vi "OP_Print_TPS_cluster_20171110.vi"() -> ()   [LabVIEW 2013]
uses:
  <vilib>/addons/database/Connection.llb/DB Tools Open Connec (Path).vi
  <vilib>/addons/database/Connection.llb/Conn Execute.vi
  <vilib>/addons/database/Recordset.llb/Rec Fetch Recordset Data (R).vi
  <vilib>/addons/database/Recordset.llb/Rec Destroy - Connection.vi
  <userlib>/caLab/Private/Get_PV-1D.vi
  <vilib>/Utility/file.llb/Write To Spreadsheet File (string).vi
  <userlib>/caLab/Private/Get_PV.vi
  <vilib>/addons/database/NI_Database_API.lvlib
panel:
  in  "T:Slow\nF:Fast":bool
  in  "Switch Tab":bool=TRUE
  out "Tab Control":enum32{"_____", "           "}(tab)
  out "Cluster":T1={"SR Fill Pattern"=[], "Beam Current(mA"=320.769453, "Beam Lifetime(min)"=354.3939151043138, "Beamsize X(um)"=63.15189373514937, "Beamsize Y(um)"=38.03691397287648, "Tune X(from BPM)"=0.1487279843444227, "Tune Y(from BPM)"=0.2309197651663405, "Mode"="Top-Up", "NuX(from BBF) "=0.15142063757609414, "NuY(from BBF)"=0.22496346361412184, "IU22-23gap(R)"=7.0, "IU22-05gap(R)"=7.372, "IU22-05M"=TRUE, "IU22A-09gap(R)"=8.05, "IU22A-09M"=TRUE, "IU22B-09gap(R)"=40.001, "IU22B-09M"=FALSE, "IUT22-21gap(R)"=7.0, "IUT22-21M"=TRUE, "IU22-23M"=TRUE, "IU22A-25gap(R)"=7.0, "IU22A-25M"=TRUE, "IU22B-25gap(R)"=40.0, "IU22B-25M"=FALSE, "EPU48A-41gap(R)"=65.00055, "EPU48A-41gM"=FALSE, "EPU48B-41gap(R)"=27.450000000000003, "EPU48B-41gM"=TRUE, "EPU46-45gap(R)"=44.99850000000001, "EPU46-45gM"=FALSE, "EPU48A-41phase(R)"=0.00055, "EPU48B-41phase(R)"=0.0, "EPU46-45phase(R)"=5e-05, "Grid volt.(V)[S]"=33.0, "Gun mode"="MBM", "Mod.3 HV(kV)[S]"=35.37999999999996, "SR"="SR_DMB_2017_1024_0300LOCO.data", "BR"="Booster_2017_1023_0900.data", "LI"="Linac_2017_0413_1015.data", "LTB"="LTB_JT_2017_0828_1050.data", "BTS"="BTS_2017_1023_0900.data", "RF2 remote"=TRUE, "RF2 OP mode"=TRUE, "RF2 phase.[S]"=-42.0, "RF Freq.(s)"=499655365.67399085, "RF2 gap volt[S]"=1600.0, "RF3 remote"=TRUE, "RF3 OP mode"=TRUE, "RF3 phase.[S]"=1.1999999999999995, "RF3 gap volt.[S]"=1600.0, "BBF V"=TRUE, "BBF H"=TRUE, "BR ext. kicker1(kV)"=17.666, "BR ext. kicker2(kV)"=17.666, "BR ext. sep.1(V)"=322.14, "BR ext. sep.2(V)"=441.1, "BR inj. sep.(V)"=104.95, "BR inj. kicker(kV)"=13.449999999999969, "SR kicker4(kV)"=7.945, "SR kicker3(kV)"=8.02, "SR kicker2(kV)"=8.142, "SR kicker1(kV)"=8.1, "SR inj. sep.2(V)"=397.2, "SR inj. sep.1(V)"=398.04, "Bucket Start"=100.0, "Bucket Last"=450.0, "Bucket Step"=10.0, "Orbit ILK(P)"=TRUE, "IU22-05 Hutch Enable"=TRUE, "IU22A-09M Hutch Enable"=TRUE, "IUT22-21M Hutch Enable"=TRUE, "IU22-23M Hutch Enable"=TRUE, "IU22A-25M Hutch Enable"=TRUE, "EPU48A-41M Hutch Enable"=TRUE, "EPU46-45M Hutch Enable"=FALSE, "EPU46-45 FE Enable"=TRUE, "EPU48A-41 FE Enable"=TRUE, "IU22A-25 FE Enable"=TRUE, "IU22-23 FE Enable"=TRUE, "IUT22-21 FE Enable"=TRUE, "IU22A-09 FE Enable"=TRUE, "IU22-05 FE Enable"=TRUE, "EPU48A-41pM"=FALSE, "EPU48B-41pM"=TRUE, "EPU46-45pM"=FALSE, "Gun volt.(V)[S]"=23.5, "Width count"=75.0, "2ns step"=2.0, "10ps delay"=150.0, "phase shifter"=130.0015, "Taper"=1.0899999999999999, "05XBPMX 1"=14.279, "09XBPMX 1"=-34.837, "21XBPMX 1"=-36.466, "23XBPMX 1"=-38.547000000000004, "25XBPMX 1"=-40.08, "41XBPMX 1"=-513.551, "45XBPMX 1"=-12.86, "05XBPMY 1"=51.999, "09XBPMY 1"=30.004, "21XBPMY 1"=-4.771, "23XBPMY 1"=19.080000000000002, "25XBPMY 1"=-4.366, "41XBPMY 1"=309.241, "45XBPMY 1"=1.842, "FOFB H"="On", "FOFB V"="On", "time string"="15:45:09", "date"="2017/10/28", "date (last kicker ON)"="2017/10/28", "time string (last kicker ON)"="15:43:52", "Radio Buttons 2"=enum."absolute", "09XBPMX 2"="23.77", "09XBPMY 2"="-18.01", "05XBPMY 2"="-459.85", "05XBPMX 2"="-403.56", "21XBPMY 2"="-134.87", "21XBPMX 2"="-31.92", "23XBPMY 2"="233.82", "23XBPMX 2"="11.09", "25XBPMY 2"="5171.53", "25XBPMX 2"="2152.43", "41XBPMY 2"=" closed", "41XBPMX 2"=" PAB ", "45XBPMX 2"=" Hutch ", "45XBPMY 2"=" closed", "05 mode"="Follow", "09A mode"="Follow", "09B mode"="Follow", "21 mode"="Follow", "23 mode"="Follow", "25A mode"="Follow", "25B mode"="Follow", "41A mode"="Follow", "41B mode"="Follow", "46 mode"="Follow", "BeamCurrent History"={"BPM NO.  1_172"=array[4319 elements], array[4319 elements]}, "SR Beam Current in            hours"=12.0, "RF FB"="On", "BPMX Graph 2"={"Array of X axis  平均分配至各段"=[1.0, 1.1666666666666667, 1.3333333333333333, 1.5, 1.6666666666666665, 1.8333333333333333, 2.0, 2.142857142857143, 2.2857142857142856, 2.4285714285714284, 2.571428571428571, 2.7142857142857144, 2.857142857142857, 3.0, 3.142857142857143, 3.2857142857142856, 3.4285714285714284, 3.571428571428571, 3.7142857142857144, 3.857142857142857, 4.0, 4.125, 4.25, 4.375, 4.5, 4.625, 4.75, 4.875, 5.0, 5.125, 5.25, 5.375, 5.5, 5.625, 5.75, 5.875, 6.0, 6.142857142857143, 6.285714285714286, 6.428571428571429, 6.571428571428571, 6.714285714285714, 6.857142857142857, 7.0, 7.142857142857143, 7.285714285714286, 7.428571428571429, 7.571428571428571, 7.714285714285714, 7.857142857142857, 8.0, 8.142857142857142, 8.285714285714286, 8.428571428571429, 8.571428571428571, 8.714285714285714, 8.857142857142858, 9.0, 9.142857142857142, 9.285714285714286, 9.428571428571429, 9.571428571428571, 9.714285714285714, 9.857142857142858, 10.0, 10.142857142857142, 10.285714285714286, 10.428571428571429, 10.571428571428571, 10.714285714285714, 10.857142857142858, 11.0, 11.142857142857142, 11.285714285714286, 11.428571428571429, 11.571428571428571, 11.714285714285714, 11.857142857142858, 12.0, 12.125, 12.25, 12.375, 12.5, 12.625, 12.75, 12.875, 13.0, 13.125, 13.25, 13.375, 13.5, 13.625, 13.75, 13.875, 14.0, 14.142857142857142, 14.285714285714286, 14.428571428571429, 14.571428571428571, 14.714285714285714, 14.857142857142858, 15.0, 15.142857142857142, 15.285714285714286, 15.428571428571429, 15.571428571428571, 15.714285714285714, 15.857142857142858, 16.0, 16.142857142857142, 16.285714285714285, 16.428571428571427, 16.571428571428573, 16.714285714285715, 16.857142857142858, 17.0, 17.142857142857142, 17.285714285714285, 17.428571428571427, 17.571428571428573, 17.714285714285715, 17.857142857142858, 18.0, 18.142857142857142, 18.285714285714285, 18.428571428571427, 18.571428571428573, 18.714285714285715, 18.857142857142858, 19.0, 19.142857142857142, 19.285714285714285, 19.428571428571427, 19.571428571428573, 19.714285714285715, 19.857142857142858, 20.0, 20.125, 20.25, 20.375, 20.5, 20.625, 20.75, 20.875, 21.0, 21.125, 21.25, 21.375, 21.5, 21.625, 21.75, 21.875, 22.0, 22.142857142857142, 22.285714285714285, 22.428571428571427, 22.571428571428573, 22.714285714285715, 22.857142857142858, 23.0, 23.142857142857142, 23.285714285714285, 23.428571428571427, 23.571428571428573, 23.714285714285715, 23.857142857142858, 24.0, 24.166666666666668, 24.333333333333332, 24.5, 24.666666666666668, 24.833333333333332], [-104.35000000000001, -27.61, -81.269, 31.074, 6.062, -136.0, 99.494, -88.141, -46.889, -165.06900000000002, 6.021, -84.98, 1.75, -8.811, 8.532, -133.949, -96.848, 24.799, 5.059, -100.301, 144.643, -9.353, 21.271, -55.053000000000004, 53.308, 191.175, 158.868, 222.566, -123.501, -26.869, 534.8770000000001, 573.141, -225.076, -6.779, 120.711, -75.419, 85.256, 50.948, -59.4, -203.09900000000002, -20.847, 130.465, -112.508, 76.115, 15.039, -35.207, -105.659, -16.897000000000002, 68.91, -141.159, 107.378, 144.351, -55.053000000000004, -193.076, 129.21, 58.157000000000004, -162.566, 153.643, 28.149, 9.358, -84.211, 85.112, 22.422, -31.252, 89.379, -47.49, 54.793, -68.275, 110.611, -118.584, -371.90500000000003, -20.115000000000002, -329.103, -249.097, -146.817, 118.556, -25.749, -98.32600000000001, 55.269, -122.093, 50.967, -55.89, 88.019, -0.462, -608.1560000000001, -139.752, -304.999, -215.022, 93.23400000000001, 44.699, -65.235, 37.049, -3.491, -169.852, 216.458, 50.398, -92.285, -132.13400000000001, -12.869, 66.74, -188.53300000000002, 148.653, -5.112, -71.334, -177.681, 41.168, -12.532, -184.913, 194.919, 52.414, -75.628, -80.415, -36.814, 105.73100000000001, -104.36800000000001, 110.101, 49.669000000000004, -67.327, -157.372, 29.624000000000002, 22.156, -105.663, 47.799, 11.591000000000001, -75.285, -79.821, 34.331, -24.937, -158.703, 177.15, 200.872, -165.849, -60.67, 20.183, -15.311, -111.206, 107.58800000000001, 26.489, 69.547, -41.230000000000004, 81.986, 54.43, 253.076, 378.43600000000004, -117.003, -304.999, 131.013, 2.21, -158.435, 94.489, 63.017, -82.94500000000001, 99.147, 65.752, -37.261, -102.577, 41.791000000000004, 66.599, -163.73, 160.137, -7.15, -51.275, -140.353, 33.772, 54.203, -147.597, 128.696, 58.22, -47.144, -184.493, 56.980000000000004, 67.437, -54.227000000000004, -0.031]}, "BPMY Graph 2"={"Array of X axis  平均分配至各段"=[1.0, 1.1666666666666667, 1.3333333333333333, 1.5, 1.6666666666666665, 1.8333333333333333, 2.0, 2.142857142857143, 2.2857142857142856, 2.4285714285714284, 2.571428571428571, 2.7142857142857144, 2.857142857142857, 3.0, 3.142857142857143, 3.2857142857142856, 3.4285714285714284, 3.571428571428571, 3.7142857142857144, 3.857142857142857, 4.0, 4.125, 4.25, 4.375, 4.5, 4.625, 4.75, 4.875, 5.0, 5.125, 5.25, 5.375, 5.5, 5.625, 5.75, 5.875, 6.0, 6.142857142857143, 6.285714285714286, 6.428571428571429, 6.571428571428571, 6.714285714285714, 6.857142857142857, 7.0, 7.142857142857143, 7.285714285714286, 7.428571428571429, 7.571428571428571, 7.714285714285714, 7.857142857142857, 8.0, 8.142857142857142, 8.285714285714286, 8.428571428571429, 8.571428571428571, 8.714285714285714, 8.857142857142858, 9.0, 9.142857142857142, 9.285714285714286, 9.428571428571429, 9.571428571428571, 9.714285714285714, 9.857142857142858, 10.0, 10.142857142857142, 10.285714285714286, 10.428571428571429, 10.571428571428571, 10.714285714285714, 10.857142857142858, 11.0, 11.142857142857142, 11.285714285714286, 11.428571428571429, 11.571428571428571, 11.714285714285714, 11.857142857142858, 12.0, 12.125, 12.25, 12.375, 12.5, 12.625, 12.75, 12.875, 13.0, 13.125, 13.25, 13.375, 13.5, 13.625, 13.75, 13.875, 14.0, 14.142857142857142, 14.285714285714286, 14.428571428571429, 14.571428571428571, 14.714285714285714, 14.857142857142858, 15.0, 15.142857142857142, 15.285714285714286, 15.428571428571429, 15.571428571428571, 15.714285714285714, 15.857142857142858, 16.0, 16.142857142857142, 16.285714285714285, 16.428571428571427, 16.571428571428573, 16.714285714285715, 16.857142857142858, 17.0, 17.142857142857142, 17.285714285714285, 17.428571428571427, 17.571428571428573, 17.714285714285715, 17.857142857142858, 18.0, 18.142857142857142, 18.285714285714285, 18.428571428571427, 18.571428571428573, 18.714285714285715, 18.857142857142858, 19.0, 19.142857142857142, 19.285714285714285, 19.428571428571427, 19.571428571428573, 19.714285714285715, 19.857142857142858, 20.0, 20.125, 20.25, 20.375, 20.5, 20.625, 20.75, 20.875, 21.0, 21.125, 21.25, 21.375, 21.5, 21.625, 21.75, 21.875, 22.0, 22.142857142857142, 22.285714285714285, 22.428571428571427, 22.571428571428573, 22.714285714285715, 22.857142857142858, 23.0, 23.142857142857142, 23.285714285714285, 23.428571428571427, 23.571428571428573, 23.714285714285715, 23.857142857142858, 24.0, 24.166666666666668, 24.333333333333332, 24.5, 24.666666666666668, 24.833333333333332], [-143.858, -13.775, -13.785, 122.665, -66.475, 31.541, 2.118, -24.67, 28.275000000000002, 0.139, -36.578, -28.396, 48.925000000000004, 9.287, -3.412, 70.053, -21.479, 14.89, -7.234, 5.521, -3.164, 19.558, -37.538000000000004, 37.11, -77.159, -13.755, 77.63, 28.249000000000002, -209.114, -44.569, 92.851, 173.641, -70.156, -22.722, 17.795, -6.59, 25.654, -41.882, 53.713, 9.237, -26.164, 18.357, 63.695, -8.542, 5.183, -5.99, 9.508000000000001, -5.462, -29.446, 36.574, -52.552, 51.439, -48.502, 0.73, -23.836000000000002, -3.648, -9.628, -5.485, -68.679, 95.486, -62.041000000000004, 54.633, -58.791000000000004, 68.305, -49.682, 29.838, -8.459, 3.213, -5.561, -80.617, 58.144, 15.346, -158.743, -40.726, 5.259, 3.258, 41.128, -54.377, 5.01, 18.84, 11.403, -20.73, 21.792, -17.296, 27.29, 0.783, -6.804, -137.476, 116.70700000000001, -6.929, 17.846, -3.586, 11.754, 6.341, 0.292, -0.911, -8.236, -5.312, 14.939, -29.945, 30.573, -9.991, -49.344, 82.117, -27.45, 22.291, -6.636, -9.389, 10.034, -14.218, 14.215, -7.3, 12.409, -44.302, 50.197, -36.089, -9.120000000000001, 45.881, 14.836, -27.324, 10.765, -10.139, -33.252, 2.737, -9.99, -6.019, -53.329, -28.159, 2.676, -36.9, -2.372, 8.92, 13.599, -25.723, -16.436, 7.722, -0.088, -29.122, 32.814, -20.521, 30.155, -45.734, 36.611000000000004, 74.528, 68.482, -22.548000000000002, -31.398, 134.603, -45.587, -0.981, -40.156, 24.441, 20.477, -31.424, 19.5, -11.789, 16.394000000000002, -38.567, 9.523, 0.09, -0.058, -4.8500000000000005, 11.71, 25.637, -10.51, -18.101, -12.389000000000001, 95.417, -138.726, 30.355, 96.245, -48.666000000000004, 40.851, -0.71]}, "gap value："=0, "BR Fill Pattern"=[], "time string (last INJ) "=""} {"SR Beam Current in            hours" min=1.0 max=24.0 step=1.0 format="%#_2f"; "45XBPMY 1" format="%#.2f"; "41XBPMY 1" format="%#.2f"; "25XBPMY 1" format="%#.2f"; "23XBPMY 1" format="%#.2f"; "21XBPMY 1" format="%#.2f"; "09XBPMY 1" format="%#.2f"; "05XBPMY 1" format="%#.2f"; "45XBPMX 1" format="%#.2f"; "41XBPMX 1" format="%#.2f"; "25XBPMX 1" format="%#.2f"; "23XBPMX 1" format="%#.2f"; "21XBPMX 1" format="%#.2f"; "09XBPMX 1" format="%#.2f"; "05XBPMX 1" format="%#.2f"; "Taper" format="%#.4f"; "phase shifter" format="%#.3f"; "10ps delay" format="%#.1f"; "2ns step" format="%#.1f"; "Width count" format="%#.1f"; "Gun volt.(V)[S]" format="%#.1f"; "Bucket Step" format="%#.2f"; "Bucket Last" format="%#.2f"; "Bucket Start" format="%#.2f"; "BR ext. kicker1(kV)" format="%#.2f"; "BR ext. kicker2(kV)" format="%#.2f"; "BR ext. sep.1(V)" format="%#.2f"; "BR ext. sep.2(V)" format="%#.2f"; "BR inj. sep.(V)" format="%#.3f"; "BR inj. kicker(kV)" format="%#.3f"; "SR kicker4(kV)" format="%#.2f"; "SR kicker3(kV)" format="%#.2f"; "SR kicker2(kV)" format="%#.2f"; "SR kicker1(kV)" format="%#.2f"; "SR inj. sep.2(V)" format="%#.2f"; "SR inj. sep.1(V)" format="%#.2f"; "RF3 gap volt.[S]" format="%#.0f"; "RF3 phase.[S]" format="%#.1f"; "RF2 gap volt[S]" format="%#.0f"; "RF Freq.(s)" format="%#.1f"; "RF2 phase.[S]" format="%#.1f"; "Mod.3 HV(kV)[S]" format="%#.3f"; "Grid volt.(V)[S]" format="%#.1f"; "EPU46-45phase(R)" format="%#.4f"; "EPU48B-41phase(R)" format="%#.4f"; "EPU48A-41phase(R)" format="%#.4f"; "EPU46-45gap(R)" format="%#.4f"; "EPU48B-41gap(R)" format="%#.4f"; "EPU48A-41gap(R)" format="%#.4f"; "IU22B-25gap(R)" format="%#.4f"; "IU22A-25gap(R)" format="%#.4f"; "IUT22-21gap(R)" format="%#.4f"; "IU22B-09gap(R)" format="%#.4f"; "IU22A-09gap(R)" format="%#.4f"; "IU22-05gap(R)" format="%#.4f"; "IU22-23gap(R)" format="%#.4f"; "NuY(from BBF)" format="%#.4f"; "NuX(from BBF)" format="%#.4f"; "Tune Y(from BPM)" format="%#.4f"; "Tune X(from BPM)" format="%#.4f"; "Beamsize Y(um)" format="%#.2f"; "Beamsize X(um)" format="%#.2f"; "Beam Lifetime(min)" format="%#.3f"; "Beam Current(mA" format="%#.3f"}
  out "Diff list":string[][](array[string])
  out "EVENTs":i32
  out "check loop":i32
  in  "Check period":i32=10 min=0 max=10
  out "Program Start Time":dbl=3592021508.642459
  out "dT":u32=325
  out "PV list":string[](array[string])=["LI-ES-CPS-01:SETMODE", "LI-ES-CPS-01:PULSEMODE", "LI-ES-BPS-01:SETU:GRID", "LI-ES-BPS-01:SETU:SBM", "LI-ES-BPS-01:SETU:MBM", "LI-RF-CAB-07:SET:MODE", "LI-RF-HVP-11:SET:U", "LI-RF-CAB-09:SET:MODE", "LI-RF-HVP-21:SET:U", "LI-RF-CAB-11:SET:MODE", "LI-RF-HVP-31:SET:U", "LI-RF-WGA-01:SET:POS", "LI-RF-WGA-02:SET:POS", "LI-RF-WGA-03:SET:POS", "LI-RF-SFT-01:SET:POS", "LI-RF-SFT-02:SET:POS", "LI-RF-SFT-03:SET:POS", "LI-RF-CTR-01:ES:SET:DEG", "LI-RF-CTR-01:SP:SET:DEG", "LI-RF-CTR-01:K123:SET:DEG", "LI-RF-CTR-01:K1:SET:DEG", "LI-RF-CTR-01:K3:SET:DEG", "LI-RF-AMP-01:SET:PWR", "LI-RF-AMP-02:SET:PWR", "LI-MA-SPS-01:SET:I", "LI-MA-SPS-02:SET:I", "LI-MA-SPS-03:SET:I", "LI-MA-SPS-04:SET:I", "LI-MA-SPS-05:SET:I", "LI-MA-SPS-06:SET:I", "LI-MA-SPS-07:SET:I", "LI-MA-SPS-08:SET:I", "LI-MA-SPS-09:SET:I", "LI-MA-SPS-10:SET:I", "LI-MA-SPS-11:SET:I", "LI-MA-SPS-12:SET:I", "LI-MA-SPS-13:SET:I", "LI-MA-SPS-14:SET:I", "LI-MA-SPS-15:SET:I", "LI-MA-SPS-16:SET:I", "LI-MA-STP-01:SET:I", "LI-MA-STP-02:SET:I", "LI-MA-STP-03:SET:I", "LI-MA-STP-04:SET:I", "LI-MA-STP-05:SET:I", "LI-MA-STP-06:SET:I", "LI-MA-STP-07:SET:I", "LI-MA-STP-08:SET:I", "LI-MA-STP-09:SET:I", "LI-MA-STP-10:SET:I", "LI-MA-STP-11:SET:I", "LI-MA-STP-12:SET:I", "LI-MA-STP-13:SET:I", "LI-MA-STP-14:SET:I", "LI-MA-STP-15:SET:I", "LI-MA-STP-16:SET:I", "LI-MA-QPS-01:SET:I", "LI-MA-QPS-02:SET:I", "LI-MA-QPS-03:SET:I", "LI-MA-QPS-04:SET:I", "LI-MA-QPS-05:SET:I", "LI-MA-QPS-06:SET:I", "CPCITM-TI-EVRTG:Pulse7DelaySet", "CPCITM-TI-EVRTG:Pulse7WidthSet", "CPCITM-TI-EVRTG:GTX7CtrlGTXPHSet", "CPCITM-TI-EVRTG:GTX7DlySet", "CPCITM-TI-EVRTG:Pulse6DelaySet", "CPCITM-TI-EVRTG:Pulse6WidthSet", "CPCITM-TI-EVRTG:GTX6CtrlGTXPHSet", "CPCITM-TI-EVRTG:GTX6DlySet", "CPCILI-TI-EVR:Pulse2DelaySet", "CPCILI-TI-EVR:Pulse2WidthSet", "CPCILI-TI-EVR:Pulse3DelaySet", "CPCILI-TI-EVR:Pulse3WidthSet", "CPCILI-TI-EVR:Pulse4DelaySet", "CPCILI-TI-EVR:Pulse4WidthSet", "CPCILI-TI-EVR:Pulse5DelaySet", "CPCILI-TI-EVR:Pulse5WidthSet", "CPCILI-TI-EVR:Pulse6DelaySet", "CPCILI-TI-EVR:Pulse6WidthSet", "CPCILI-TI-EVR:Pulse7DelaySet", "CPCILI-TI-EVR:Pulse7WidthSet", "CPCILI-TI-EVR:Pulse8DelaySet", "CPCILI-TI-EVR:Pulse8WidthSet", "CPCILI-TI-EVR:Pulse9DelaySet", "CPCILI-TI-EVR:Pulse9WidthSet", "CPCITM-TI-EVRTG:GTX6DlySet", "CPCITM-TI-EVRTG:GTX7DlySet", "LTB-PS-HC-1:setI", "LTB-PS-HC-2:setI", "LTB-PS-HC-3:setI", "LTB-PS-HC-4:setI", "LTB-PS-HC-5:setI", "LTB-PS-VC-1:setI", "LTB-PS-VC-2:setI", "LTB-PS-VC-3:setI", "LTB-PS-VC-4:setI", "LTB-PS-VC-5:setI", "LTB-PS-VC-6:setI", "LTB-PS-VC-7:setI", "LTB-PS-Q1A:setI", "LTB-PS-Q1B:setI", "LTB-PS-Q1C:setI", "LTB-PS-Q2A:setI", "LTB-PS-Q2B:setI", "LTB-PS-Q2C:setI", "LTB-PS-Q3A:setI", "LTB-PS-Q3B:setI", "LTB-PS-Q4A:setI", "LTB-PS-Q4B:setI", "LTB-PS-QQ:setI", "LTB-PS-BEND-1:setI", "LTB-PS-VC-2a:setI", "LTB-PS-HC-3a:setI", "LTB-PS-HC-3b:setI", "LTB-PS-HC-4a:setI", "LTB-PS-HC-5a:setI", "LI-DI-SLIT-motor:axis2Position1", "LI-DI-SLIT-motor:axis1Position1", "BR-PS-HC-101:setI", "BR-PS-HC-102:setI", "BR-PS-HC-103:setI", "BR-PS-HC-104:setI", "BR-PS-HC-105:setI", "BR-PS-HC-106:setI", "BR-PS-HC-107:setI", "BR-PS-HC-108:setI", "BR-PS-HC-109:setI", "BR-PS-HC-110:setI", "BR-PS-HC-201:setI", "BR-PS-HC-202:setI", "BR-PS-HC-203:setI", "BR-PS-HC-204:setI", "BR-PS-HC-205:setI", "BR-PS-HC-206:setI", "BR-PS-HC-207:setI", "BR-PS-HC-208:setI", "BR-PS-HC-209:setI", "BR-PS-HC-210:setI", "BR-PS-HC-301:setI", "BR-PS-HC-302:setI", "BR-PS-HC-303:setI", "BR-PS-HC-304:setI", "BR-PS-HC-305:setI", "BR-PS-HC-306:setI", "BR-PS-HC-307:setI", "BR-PS-HC-308:setI", "BR-PS-HC-309:setI", "BR-PS-HC-310:setI", "BR-PS-HC-401:setI", "BR-PS-HC-402:setI", "BR-PS-HC-403:setI", "BR-PS-HC-404:setI", "BR-PS-HC-405:setI", "BR-PS-HC-406:setI", "BR-PS-HC-407:setI", "BR-PS-HC-408:setI", "BR-PS-HC-409:setI", "BR-PS-HC-410:setI", "BR-PS-HC-501:setI", "BR-PS-HC-502:setI", "BR-PS-HC-503:setI", "BR-PS-HC-504:setI", "BR-PS-HC-505:setI", "BR-PS-HC-506:setI", "BR-PS-HC-507:setI", "BR-PS-HC-508:setI", "BR-PS-HC-509:setI", "BR-PS-HC-510:setI", "BR-PS-HC-601:setI", "BR-PS-HC-602:setI", "BR-PS-HC-603:setI", "BR-PS-HC-603a:setI", "BR-PS-HC-604:setI", "BR-PS-HC-605:setI", "BR-PS-HC-606:setI", "BR-PS-HC-606a:setI", "BR-PS-HC-607:setI", "BR-PS-HC-608:setI", "BR-PS-HC-609:setI", "BR-PS-HC-610:setI", "BR-PS-VC-101:setI", "BR-PS-VC-102:setI", "BR-PS-VC-103:setI", "BR-PS-VC-104:setI", "BR-PS-VC-105:setI", "BR-PS-VC-106:setI", "BR-PS-VC-201:setI", "BR-PS-VC-202:setI", "BR-PS-VC-203:setI", "BR-PS-VC-204:setI", "BR-PS-VC-205:setI", "BR-PS-VC-206:setI", "BR-PS-VC-301:setI", "BR-PS-VC-302:setI", "BR-PS-VC-303:setI", "BR-PS-VC-304:setI", "BR-PS-VC-305:setI", "BR-PS-VC-306:setI", "BR-PS-VC-401:setI", "BR-PS-VC-402:setI", "BR-PS-VC-403:setI", "BR-PS-VC-404:setI", "BR-PS-VC-405:setI", "BR-PS-VC-406:setI", "BR-PS-VC-501:setI", "BR-PS-VC-502:setI", "BR-PS-VC-503:setI", "BR-PS-VC-504:setI", "BR-PS-VC-505:setI", "BR-PS-VC-506:setI", "BR-PS-VC-601:setI", "BR-PS-VC-602:setI", "BR-PS-VC-602a:setI", "BR-PS-VC-603:setI", "BR-PS-VC-604:setI", "BR-PS-VC-604a:setI", "BR-PS-VC-605:setI", "BR-PS-VC-606:setI", "BR-PS-VC-100a:setI", "BR-PS-SD:setI", "BR-PS-SF:setI", "cpsc_027:AO:SLOW_SET:CH:1", "cpsc_037:AO:SLOW_SET:CH:3", "BR-RF-LLRF:setStationPhase", "TI-INJ-PROC:setTinj", "BR-PS-INJ-SE:setHV", "CPCIPM-TI-EVR:Pulse1DelaySet", "BR-PS-INJ-KI:setHV", "CPCIPM-TI-EVR:Pulse2DelaySet", "BR-PS-QF:setWfDC", "BR-PS-QM:setWfDC", "BR-PS-Q1:setWfDC", "BR-PS-Q2:setWfDC", "BR-PS-BEND:setWfDC", "BTS-PS-HC-1:setI", "BTS-PS-HC-2:setI", "BTS-PS-HC-3:setI", "BTS-PS-HC-4:setI", "BTS-PS-HC-5:setI", "BTS-PS-VC-2:setI", "BTS-PS-VC-3:setI", "BTS-PS-VC-4:setI", "BTS-PS-VC-5:setI", "BTS-PS-VC-6:setI", "BTS-PS-Q1A:setI", "BTS-PS-Q1B:setI", "BTS-PS-Q1C:setI", "BTS-PS-Q2A:setI", "BTS-PS-Q2B:setI", "BTS-PS-Q2C:setI", "BTS-PS-Q3A:setI", "BTS-PS-BEND-1:setI", "BTS-PS-BEND-2:setI", "BR-PS-EXT-K1:setHV", "BR-PS-EXT-K2:setHV", "SR-PS-INJ-SE1:setHV", "SR-PS-INJ-SE2:setHV", "SR-PS-INJ-K1:setHV", "SR-PS-INJ-K2:setHV", "SR-PS-INJ-K3:setHV", "SR-PS-INJ-K4:setHV", "CPCIPM-TI-EVR:Pulse4DelaySet", "CPCIPM-TI-EVR:Pulse5DelaySet", "CPCIPM-TI-EVR:Pulse3DelaySet", "CPCIPM-TI-EVR:Pulse6DelaySet", "CPCIPM-TI-EVR:Pulse7DelaySet", "T560:setADelay", "T560:setBDelay", "T560:setCDelay", "T560:setDDelay", "CPCIPM-TI-EVR:Pulse4DelaySet", "CPCIPM-TI-EVR:Pulse5DelaySet", "BR-PS-EXT-SE1:setHV", "BR-PS-EXT-SE2:setHV", "CPCIPM-TI-EVR:Pulse3DelaySet", "CPCIPM-TI-EVR:Pulse11DelaySet", "SR-PS-BEND:setI", "SR-PS-HC-011:setI", "SR-PS-HC-012:setI", "SR-PS-HC-013:setI", "SR-PS-HC-014:setI", "SR-PS-HC-015:setI", "SR-PS-HC-016:setI", "SR-PS-HC-017:setI", "SR-PS-HC-021:setI", "SR-PS-HC-022:setI", "SR-PS-HC-023:setI", "SR-PS-HC-024:setI", "SR-PS-HC-025:setI", "SR-PS-HC-026:setI", "SR-PS-HC-027:setI", "SR-PS-HC-031:setI", "SR-PS-HC-032:setI", "SR-PS-HC-033:setI", "SR-PS-HC-034:setI", "SR-PS-HC-035:setI", "SR-PS-HC-036:setI", "SR-PS-HC-037:setI", "SR-PS-HC-041:setI", "SR-PS-HC-042:setI", "SR-PS-HC-043:setI", "SR-PS-HC-044:setI", "SR-PS-HC-045:setI", "SR-PS-HC-046:setI", "SR-PS-HC-047:setI", "SR-PS-HC-051:setI", "SR-PS-HC-052:setI", "SR-PS-HC-053:setI", "SR-PS-HC-054:setI", "SR-PS-HC-055:setI", "SR-PS-HC-056:setI", "SR-PS-HC-057:setI", "SR-PS-HC-061:setI", "SR-PS-HC-062:setI", "SR-PS-HC-063:setI", "SR-PS-HC-064:setI", "SR-PS-HC-065:setI", "SR-PS-HC-066:setI", "SR-PS-HC-067:setI", "SR-PS-HC-071:setI", "SR-PS-HC-072:setI", "SR-PS-HC-073:setI", "SR-PS-HC-074:setI", "SR-PS-HC-075:setI", "SR-PS-HC-076:setI", "SR-PS-HC-077:setI", "SR-PS-HC-081:setI", "SR-PS-HC-082:setI", "SR-PS-HC-083:setI", "SR-PS-HC-084:setI", "SR-PS-HC-085:setI", "SR-PS-HC-086:setI", "SR-PS-HC-087:setI", "SR-PS-HC-091:setI", "SR-PS-HC-092:setI", "SR-PS-HC-093:setI", "SR-PS-HC-094:setI", "SR-PS-HC-095:setI", "SR-PS-HC-096:setI", "SR-PS-HC-097:setI", "SR-PS-HC-101:setI", "SR-PS-HC-102:setI", "SR-PS-HC-103:setI", "SR-PS-HC-104:setI", "SR-PS-HC-105:setI", "SR-PS-HC-106:setI", "SR-PS-HC-107:setI", "SR-PS-HC-111:setI", "SR-PS-HC-112:setI", "SR-PS-HC-113:setI", "SR-PS-HC-114:setI", "SR-PS-HC-115:setI", "SR-PS-HC-116:setI", "SR-PS-HC-117:setI", "SR-PS-HC-121:setI", "SR-PS-HC-122:setI", "SR-PS-HC-123:setI", "SR-PS-HC-124:setI", "SR-PS-HC-125:setI", "SR-PS-HC-126:setI", "SR-PS-HC-127:setI", "SR-PS-HC-131:setI", "SR-PS-HC-132:setI", "SR-PS-HC-133:setI", "SR-PS-HC-134:setI", "SR-PS-HC-135:setI", "SR-PS-HC-136:setI", "SR-PS-HC-137:setI", "SR-PS-HC-141:setI", "SR-PS-HC-142:setI", "SR-PS-HC-143:setI", "SR-PS-HC-144:setI", "SR-PS-HC-145:setI", "SR-PS-HC-146:setI", "SR-PS-HC-147:setI", "SR-PS-HC-151:setI", "SR-PS-HC-152:setI", "SR-PS-HC-153:setI", "SR-PS-HC-154:setI", "SR-PS-HC-155:setI", "SR-PS-HC-156:setI", "SR-PS-HC-157:setI", "SR-PS-HC-161:setI", "SR-PS-HC-162:setI", "SR-PS-HC-163:setI", "SR-PS-HC-164:setI", "SR-PS-HC-165:setI", "SR-PS-HC-166:setI", "SR-PS-HC-167:setI", "SR-PS-HC-171:setI", "SR-PS-HC-172:setI", "SR-PS-HC-173:setI", "SR-PS-HC-174:setI", "SR-PS-HC-175:setI", "SR-PS-HC-176:setI", "SR-PS-HC-177:setI", "SR-PS-HC-181:setI", "SR-PS-HC-182:setI", "SR-PS-HC-183:setI", "SR-PS-HC-184:setI", "SR-PS-HC-185:setI", "SR-PS-HC-186:setI", "SR-PS-HC-187:setI", "SR-PS-HC-191:setI", "SR-PS-HC-192:setI", "SR-PS-HC-193:setI", "SR-PS-HC-194:setI", "SR-PS-HC-195:setI", "SR-PS-HC-196:setI", "SR-PS-HC-197:setI", "SR-PS-HC-201:setI", "SR-PS-HC-202:setI", "SR-PS-HC-203:setI", "SR-PS-HC-204:setI", "SR-PS-HC-205:setI", "SR-PS-HC-206:setI", "SR-PS-HC-207:setI", "SR-PS-HC-211:setI", "SR-PS-HC-212:setI", "SR-PS-HC-213:setI", "SR-PS-HC-214:setI", "SR-PS-HC-215:setI", "SR-PS-HC-216:setI", "SR-PS-HC-217:setI", "SR-PS-HC-221:setI", "SR-PS-HC-222:setI", "SR-PS-HC-223:setI", "SR-PS-HC-224:setI", "SR-PS-HC-225:setI", "SR-PS-HC-226:setI", "SR-PS-HC-227:setI", "SR-PS-HC-231:setI", "SR-PS-HC-232:setI", "SR-PS-HC-233:setI", "SR-PS-HC-234:setI", "SR-PS-HC-235:setI", "SR-PS-HC-236:setI", "SR-PS-HC-237:setI", "SR-PS-HC-241:setI", "SR-PS-HC-242:setI", "SR-PS-HC-243:setI", "SR-PS-HC-244:setI", "SR-PS-HC-245:setI", "SR-PS-HC-246:setI", "SR-PS-HC-247:setI", "SR-PS-VC-011:setI", "SR-PS-VC-012:setI", "SR-PS-VC-013:setI", "SR-PS-VC-014:setI", "SR-PS-VC-015:setI", "SR-PS-VC-016:setI", "SR-PS-VC-017:setI", "SR-PS-VC-021:setI", "SR-PS-VC-022:setI", "SR-PS-VC-023:setI", "SR-PS-VC-024:setI", "SR-PS-VC-025:setI", "SR-PS-VC-026:setI", "SR-PS-VC-027:setI", "SR-PS-VC-031:setI", "SR-PS-VC-032:setI", "SR-PS-VC-033:setI", "SR-PS-VC-034:setI", "SR-PS-VC-035:setI", "SR-PS-VC-036:setI", "SR-PS-VC-037:setI", "SR-PS-VC-041:setI", "SR-PS-VC-042:setI", "SR-PS-VC-043:setI", "SR-PS-VC-044:setI", "SR-PS-VC-045:setI", "SR-PS-VC-046:setI", "SR-PS-VC-047:setI", "SR-PS-VC-051:setI", "SR-PS-VC-052:setI", "SR-PS-VC-053:setI", "SR-PS-VC-054:setI", "SR-PS-VC-055:setI", "SR-PS-VC-056:setI", "SR-PS-VC-057:setI", "SR-PS-VC-061:setI", "SR-PS-VC-062:setI", "SR-PS-VC-063:setI", "SR-PS-VC-064:setI", "SR-PS-VC-065:setI", "SR-PS-VC-066:setI", "SR-PS-VC-067:setI", "SR-PS-VC-071:setI", "SR-PS-VC-072:setI", "SR-PS-VC-073:setI", "SR-PS-VC-074:setI", "SR-PS-VC-075:setI", "SR-PS-VC-076:setI", "SR-PS-VC-077:setI", "SR-PS-VC-081:setI", "SR-PS-VC-082:setI", "SR-PS-VC-083:setI", "SR-PS-VC-084:setI", "SR-PS-VC-085:setI", "SR-PS-VC-086:setI", "SR-PS-VC-087:setI", "SR-PS-VC-091:setI", "SR-PS-VC-092:setI", "SR-PS-VC-093:setI", "SR-PS-VC-094:setI", "SR-PS-VC-095:setI", "SR-PS-VC-096:setI", "SR-PS-VC-097:setI", "SR-PS-VC-101:setI", "SR-PS-VC-102:setI", "SR-PS-VC-103:setI", "SR-PS-VC-104:setI", "SR-PS-VC-105:setI", "SR-PS-VC-106:setI", "SR-PS-VC-107:setI", "SR-PS-VC-111:setI", "SR-PS-VC-112:setI", "SR-PS-VC-113:setI", "SR-PS-VC-114:setI", "SR-PS-VC-115:setI", "SR-PS-VC-116:setI", "SR-PS-VC-117:setI", "SR-PS-VC-121:setI", "SR-PS-VC-122:setI", "SR-PS-VC-123:setI", "SR-PS-VC-124:setI", "SR-PS-VC-125:setI", "SR-PS-VC-126:setI", "SR-PS-VC-127:setI", "SR-PS-VC-131:setI", "SR-PS-VC-132:setI", "SR-PS-VC-133:setI", "SR-PS-VC-134:setI", "SR-PS-VC-135:setI", "SR-PS-VC-136:setI", "SR-PS-VC-137:setI", "SR-PS-VC-141:setI", "SR-PS-VC-142:setI", "SR-PS-VC-143:setI", "SR-PS-VC-144:setI", "SR-PS-VC-145:setI", "SR-PS-VC-146:setI", "SR-PS-VC-147:setI", "SR-PS-VC-151:setI", "SR-PS-VC-152:setI", "SR-PS-VC-153:setI", "SR-PS-VC-154:setI", "SR-PS-VC-155:setI", "SR-PS-VC-156:setI", "SR-PS-VC-157:setI", "SR-PS-VC-161:setI", "SR-PS-VC-162:setI", "SR-PS-VC-163:setI", "SR-PS-VC-164:setI", "SR-PS-VC-165:setI", "SR-PS-VC-166:setI", "SR-PS-VC-167:setI", "SR-PS-VC-171:setI", "SR-PS-VC-172:setI", "SR-PS-VC-173:setI", "SR-PS-VC-174:setI", "SR-PS-VC-175:setI", "SR-PS-VC-176:setI", "SR-PS-VC-177:setI", "SR-PS-VC-181:setI", "SR-PS-VC-182:setI", "SR-PS-VC-183:setI", "SR-PS-VC-184:setI", "SR-PS-VC-185:setI", "SR-PS-VC-186:setI", "SR-PS-VC-187:setI", "SR-PS-VC-191:setI", "SR-PS-VC-192:setI", "SR-PS-VC-193:setI", "SR-PS-VC-194:setI", "SR-PS-VC-195:setI", "SR-PS-VC-196:setI", "SR-PS-VC-197:setI", "SR-PS-VC-201:setI", "SR-PS-VC-202:setI", "SR-PS-VC-203:setI", "SR-PS-VC-204:setI", "SR-PS-VC-205:setI", "SR-PS-VC-206:setI", "SR-PS-VC-207:setI", "SR-PS-VC-211:setI", "SR-PS-VC-212:setI", "SR-PS-VC-213:setI", "SR-PS-VC-214:setI", "SR-PS-VC-215:setI", "SR-PS-VC-216:setI", "SR-PS-VC-217:setI", "SR-PS-VC-221:setI", "SR-PS-VC-222:setI", "SR-PS-VC-223:setI", "SR-PS-VC-224:setI", "SR-PS-VC-225:setI", "SR-PS-VC-226:setI", "SR-PS-VC-227:setI", "SR-PS-VC-231:setI", "SR-PS-VC-232:setI", "SR-PS-VC-233:setI", "SR-PS-VC-234:setI", "SR-PS-VC-235:setI", "SR-PS-VC-236:setI", "SR-PS-VC-237:setI", "SR-PS-VC-241:setI", "SR-PS-VC-242:setI", "SR-PS-VC-243:setI", "SR-PS-VC-244:setI", "SR-PS-VC-245:setI", "SR-PS-VC-246:setI", "SR-PS-VC-247:setI", "SR-PS-QL1-0101:setI", "SR-PS-QL2-0102:setI", "SR-PS-QL3-0103:setI", "SR-PS-QS4-0104:setI", "SR-PS-QS5-0105:setI", "SR-PS-QS5-0106:setI", "SR-PS-QS4-0107:setI", "SR-PS-QS3-0108:setI", "SR-PS-QS2-0109:setI", "SR-PS-QS1-0110:setI", "SR-PS-QS1-0201:setI", "SR-PS-QS2-0202:setI", "SR-PS-QS3-0203:setI", "SR-PS-QS4-0204:setI", "SR-PS-QS5-0205:setI", "SR-PS-QS5-0206:setI", "SR-PS-QS4-0207:setI", "SR-PS-QS3-0208:setI", "SR-PS-QS2-0209:setI", "SR-PS-QS1-0210:setI", "SR-PS-QS1-0301:setI", "SR-PS-QS2-0302:setI", "SR-PS-QS3-0303:setI", "SR-PS-QS4-0304:setI", "SR-PS-QS5-0305:setI", "SR-PS-QS5-0306:setI", "SR-PS-QS4-0307:setI", "SR-PS-QS3-0308:setI", "SR-PS-QS2-0309:setI", "SR-PS-QS1-0310:setI", "SR-PS-QS1-0401:setI", "SR-PS-QS2-0402:setI", "SR-PS-QS3-0403:setI", "SR-PS-QS4-0404:setI", "SR-PS-QS5-0405:setI", "SR-PS-QS5-0406:setI", "SR-PS-QS4-0407:setI", "SR-PS-QL3-0408:setI", "SR-PS-QL2-0409:setI", "SR-PS-QL1-0410:setI", "SR-PS-QL1-0501:setI", "SR-PS-QL2-0502:setI", "SR-PS-QL3-0503:setI", "SR-PS-QS4-0504:setI", "SR-PS-QS5-0505:setI", "SR-PS-QS5-0506:setI", "SR-PS-QS4-0507:setI", "SR-PS-QS3-0508:setI", "SR-PS-QS2-0509:setI", "SR-PS-QS1-0510:setI", "SR-PS-QS1-0601:setI", "SR-PS-QS2-0602:setI", "SR-PS-QS3-0603:setI", "SR-PS-QS4-0604:setI", "SR-PS-QS5-0605:setI", "SR-PS-QS5-0606:setI", "SR-PS-QS4-0607:setI", "SR-PS-QS3-0608:setI", "SR-PS-QS2-0609:setI", "SR-PS-QS1-0610:setI", "SR-PS-QS1-0701:setI", "SR-PS-QS2-0702:setI", "SR-PS-QS3-0703:setI", "SR-PS-QS4-0704:setI", "SR-PS-QS5-0705:setI", "SR-PS-QS5-0706:setI", "SR-PS-QS4-0707:setI", "SR-PS-QS3-0708:setI", "SR-PS-QS2-0709:setI", "SR-PS-QS1-0710:setI", "SR-PS-QS1-0801:setI", "SR-PS-QS2-0802:setI", "SR-PS-QS3-0803:setI", "SR-PS-QS4-0804:setI", "SR-PS-QS5-0805:setI", "SR-PS-QS5-0806:setI", "SR-PS-QS4-0807:setI", "SR-PS-QL3-0808:setI", "SR-PS-QL2-0809:setI", "SR-PS-QL1-0810:setI", "SR-PS-QL1-0901:setI", "SR-PS-QL2-0902:setI", "SR-PS-QL3-0903:setI", "SR-PS-QS4-0904:setI", "SR-PS-QS5-0905:setI", "SR-PS-QS5-0906:setI", "SR-PS-QS4-0907:setI", "SR-PS-QS3-0908:setI", "SR-PS-QS2-0909:setI", "SR-PS-QS1-0910:setI", "SR-PS-QS1-1001:setI", "SR-PS-QS2-1002:setI", "SR-PS-QS3-1003:setI", "SR-PS-QS4-1004:setI", "SR-PS-QS5-1005:setI", "SR-PS-QS5-1006:setI", "SR-PS-QS4-1007:setI", "SR-PS-QS3-1008:setI", "SR-PS-QS2-1009:setI", "SR-PS-QS1-1010:setI", "SR-PS-QS1-1101:setI", "SR-PS-QS2-1102:setI", "SR-PS-QS3-1103:setI", "SR-PS-QS4-1104:setI", "SR-PS-QS5-1105:setI", "SR-PS-QS5-1106:setI", "SR-PS-QS4-1107:setI", "SR-PS-QS3-1108:setI", "SR-PS-QS2-1109:setI", "SR-PS-QS1-1110:setI", "SR-PS-QS1-1201:setI", "SR-PS-QS2-1202:setI", "SR-PS-QS3-1203:setI", "SR-PS-QS4-1204:setI", "SR-PS-QS5-1205:setI", "SR-PS-QS5-1206:setI", "SR-PS-QS4-1207:setI", "SR-PS-QL3-1208:setI", "SR-PS-QL2-1209:setI", "SR-PS-QL1-1210:setI", "SR-PS-QL1-1301:setI", "SR-PS-QL2-1302:setI", "SR-PS-QL3-1303:setI", "SR-PS-QS4-1304:setI", "SR-PS-QS5-1305:setI", "SR-PS-QS5-1306:setI", "SR-PS-QS4-1307:setI", "SR-PS-QS3-1308:setI", "SR-PS-QS2-1309:setI", "SR-PS-QS1-1310:setI", "SR-PS-QS1-1401:setI", "SR-PS-QS2-1402:setI", "SR-PS-QS3-1403:setI", "SR-PS-QS4-1404:setI", "SR-PS-QS5-1405:setI", "SR-PS-QS5-1406:setI", "SR-PS-QS4-1407:setI", "SR-PS-QS3-1408:setI", "SR-PS-QS2-1409:setI", "SR-PS-QS1-1410:setI", "SR-PS-QS1-1501:setI", "SR-PS-QS2-1502:setI", "SR-PS-QS3-1503:setI", "SR-PS-QS4-1504:setI", "SR-PS-QS5-1505:setI", "SR-PS-QS5-1506:setI", "SR-PS-QS4-1507:setI", "SR-PS-QS3-1508:setI", "SR-PS-QS2-1509:setI", "SR-PS-QS1-1510:setI", "SR-PS-QS1-1601:setI", "SR-PS-QS2-1602:setI", "SR-PS-QS3-1603:setI", "SR-PS-QS4-1604:setI", "SR-PS-QS5-1605:setI", "SR-PS-QS5-1606:setI", "SR-PS-QS4-1607:setI", "SR-PS-QL3-1608:setI", "SR-PS-QL2-1609:setI", "SR-PS-QL1-1610:setI", "SR-PS-QL1-1701:setI", "SR-PS-QL2-1702:setI", "SR-PS-QL3-1703:setI", "SR-PS-QS4-1704:setI", "SR-PS-QS5-1705:setI", "SR-PS-QS5-1706:setI", "SR-PS-QS4-1707:setI", "SR-PS-QS3-1708:setI", "SR-PS-QS2-1709:setI", "SR-PS-QS1-1710:setI", "SR-PS-QS1-1801:setI", "SR-PS-QS2-1802:setI", "SR-PS-QS3-1803:setI", "SR-PS-QS4-1804:setI", "SR-PS-QS5-1805:setI", "SR-PS-QS5-1806:setI", "SR-PS-QS4-1807:setI", "SR-PS-QS3-1808:setI", "SR-PS-QS2-1809:setI", "SR-PS-QS1-1810:setI", "SR-PS-QS1-1901:setI", "SR-PS-QS2-1902:setI", "SR-PS-QS3-1903:setI", "SR-PS-QS4-1904:setI", "SR-PS-QS5-1905:setI", "SR-PS-QS5-1906:setI", "SR-PS-QS4-1907:setI", "SR-PS-QS3-1908:setI", "SR-PS-QS2-1909:setI", "SR-PS-QS1-1910:setI", "SR-PS-QS1-2001:setI", "SR-PS-QS2-2002:setI", "SR-PS-QS3-2003:setI", "SR-PS-QS4-2004:setI", "SR-PS-QS5-2005:setI", "SR-PS-QS5-2006:setI", "SR-PS-QS4-2007:setI", "SR-PS-QL3-2008:setI", "SR-PS-QL2-2009:setI", "SR-PS-QL1-2010:setI", "SR-PS-QL1-2101:setI", "SR-PS-QL2-2102:setI", "SR-PS-QL3-2103:setI", "SR-PS-QS4-2104:setI", "SR-PS-QS5-2105:setI", "SR-PS-QS5-2106:setI", "SR-PS-QS4-2107:setI", "SR-PS-QS3-2108:setI", "SR-PS-QS2-2109:setI", "SR-PS-QS1-2110:setI", "SR-PS-QS1-2201:setI", "SR-PS-QS2-2202:setI", "SR-PS-QS3-2203:setI", "SR-PS-QS4-2204:setI", "SR-PS-QS5-2205:setI", "SR-PS-QS5-2206:setI", "SR-PS-QS4-2207:setI", "SR-PS-QS3-2208:setI", "SR-PS-QS2-2209:setI", "SR-PS-QS1-2210:setI", "SR-PS-QS1-2301:setI", "SR-PS-QS2-2302:setI", "SR-PS-QS3-2303:setI", "SR-PS-QS4-2304:setI", "SR-PS-QS5-2305:setI", "SR-PS-QS5-2306:setI", "SR-PS-QS4-2307:setI", "SR-PS-QS3-2308:setI", "SR-PS-QS2-2309:setI", "SR-PS-QS1-2310:setI", "SR-PS-QS1-2401:setI", "SR-PS-QS2-2402:setI", "SR-PS-QS3-2403:setI", "SR-PS-QS4-2404:setI", "SR-PS-QS5-2405:setI", "SR-PS-QS5-2406:setI", "SR-PS-QS4-2407:setI", "SR-PS-QL3-2408:setI", "SR-PS-QL2-2409:setI", "SR-PS-QL1-2410:setI", "SR-PS-S1-011:setI", "SR-PS-S2-012:setI", "SR-PS-SD-013:setI", "SR-PS-SF-014:setI", "SR-PS-SD-015:setI", "SR-PS-S4-016:setI", "SR-PS-S3-017:setI", "SR-PS-S5-021:setI", "SR-PS-S6-022:setI", "SR-PS-SD-023:setI", "SR-PS-SF-024:setI", "SR-PS-SD-025:setI", "SR-PS-S6-026:setI", "SR-PS-S5-027:setI", "SR-PS-S5-031:setI", "SR-PS-S6-032:setI", "SR-PS-SD-033:setI", "SR-PS-SF-034:setI", "SR-PS-SD-035:setI", "SR-PS-S6-036:setI", "SR-PS-S5-037:setI", "SR-PS-S3-041:setI", "SR-PS-S4-042:setI", "SR-PS-SD-043:setI", "SR-PS-SF-044:setI", "SR-PS-SD-045:setI", "SR-PS-S2-046:setI", "SR-PS-S1-047:setI", "SR-PS-S1-051:setI", "SR-PS-S2-052:setI", "SR-PS-SD-053:setI", "SR-PS-SF-054:setI", "SR-PS-SD-055:setI", "SR-PS-S4-056:setI", "SR-PS-S3-057:setI", "SR-PS-S5-061:setI", "SR-PS-S6-062:setI", "SR-PS-SD-063:setI", "SR-PS-SF-064:setI", "SR-PS-SD-065:setI", "SR-PS-S6-066:setI", "SR-PS-S5-067:setI", "SR-PS-S5-071:setI", "SR-PS-S6-072:setI", "SR-PS-SD-073:setI", "SR-PS-SF-074:setI", "SR-PS-SD-075:setI", "SR-PS-S6-076:setI", "SR-PS-S5-077:setI", "SR-PS-S3-081:setI", "SR-PS-S4-082:setI", "SR-PS-SD-083:setI", "SR-PS-SF-084:setI", "SR-PS-SD-085:setI", "SR-PS-S2-086:setI", "SR-PS-S1-087:setI", "SR-PS-S1-091:setI", "SR-PS-S2-092:setI", "SR-PS-SD-093:setI", "SR-PS-SF-094:setI", "SR-PS-SD-095:setI", "SR-PS-S4-096:setI", "SR-PS-S3-097:setI", "SR-PS-S5-101:setI", "SR-PS-S6-102:setI", "SR-PS-SD-103:setI", "SR-PS-SF-104:setI", "SR-PS-SD-105:setI", "SR-PS-S6-106:setI", "SR-PS-S5-107:setI", "SR-PS-S5-111:setI", "SR-PS-S6-112:setI", "SR-PS-SD-113:setI", "SR-PS-SF-114:setI", "SR-PS-SD-115:setI", "SR-PS-S6-116:setI", "SR-PS-S5-117:setI", "SR-PS-S3-121:setI", "SR-PS-S4-122:setI", "SR-PS-SD-123:setI", "SR-PS-SF-124:setI", "SR-PS-SD-125:setI", "SR-PS-S2-126:setI", "SR-PS-S1-127:setI", "SR-PS-S1-131:setI", "SR-PS-S2-132:setI", "SR-PS-SD-133:setI", "SR-PS-SF-134:setI", "SR-PS-SD-135:setI", "SR-PS-S4-136:setI", "SR-PS-S3-137:setI", "SR-PS-S5-141:setI", "SR-PS-S6-142:setI", "SR-PS-SD-143:setI", "SR-PS-SF-144:setI", "SR-PS-SD-145:setI", "SR-PS-S6-146:setI", "SR-PS-S5-147:setI", "SR-PS-S5-151:setI", "SR-PS-S6-152:setI", "SR-PS-SD-153:setI", "SR-PS-SF-154:setI", "SR-PS-SD-155:setI", "SR-PS-S6-156:setI", "SR-PS-S5-157:setI", "SR-PS-S3-161:setI", "SR-PS-S4-162:setI", "SR-PS-SD-163:setI", "SR-PS-SF-164:setI", "SR-PS-SD-165:setI", "SR-PS-S2-166:setI", "SR-PS-S1-167:setI", "SR-PS-S1-171:setI", "SR-PS-S2-172:setI", "SR-PS-SD-173:setI", "SR-PS-SF-174:setI", "SR-PS-SD-175:setI", "SR-PS-S4-176:setI", "SR-PS-S3-177:setI", "SR-PS-S5-181:setI", "SR-PS-S6-182:setI", "SR-PS-SD-183:setI", "SR-PS-SF-184:setI", "SR-PS-SD-185:setI", "SR-PS-S6-186:setI", "SR-PS-S5-187:setI", "SR-PS-S5-191:setI", "SR-PS-S6-192:setI", "SR-PS-SD-193:setI", "SR-PS-SF-194:setI", "SR-PS-SD-195:setI", "SR-PS-S6-196:setI", "SR-PS-S5-197:setI", "SR-PS-S3-201:setI", "SR-PS-S4-202:setI", "SR-PS-SD-203:setI", "SR-PS-SF-204:setI", "SR-PS-SD-205:setI", "SR-PS-S2-206:setI", "SR-PS-S1-207:setI", "SR-PS-S1-211:setI", "SR-PS-S2-212:setI", "SR-PS-SD-213:setI", "SR-PS-SF-214:setI", "SR-PS-SD-215:setI", "SR-PS-S4-216:setI", "SR-PS-S3-217:setI", "SR-PS-S5-221:setI", "SR-PS-S6-222:setI", "SR-PS-SD-223:setI", "SR-PS-SF-224:setI", "SR-PS-SD-225:setI", "SR-PS-S6-226:setI", "SR-PS-S5-227:setI", "SR-PS-S5-231:setI", "SR-PS-S6-232:setI", "SR-PS-SD-233:setI", "SR-PS-SF-234:setI", "SR-PS-SD-235:setI", "SR-PS-S6-236:setI", "SR-PS-S5-237:setI", "SR-PS-S3-241:setI", "SR-PS-S4-242:setI", "SR-PS-SD-243:setI", "SR-PS-SF-244:setI", "SR-PS-SD-245:setI", "SR-PS-S2-246:setI", "SR-PS-S1-247:setI", "SR-PS-SKEW-011:setI", "SR-PS-SKEW-012:setI", "SR-PS-SKEW-013:setI", "SR-PS-SKEW-014:setI", "SR-PS-SKEW-015:setI", "SR-PS-SKEW-016:setI", "SR-PS-SKEW-017:setI", "SR-PS-SKEW-021:setI", "SR-PS-SKEW-022:setI", "SR-PS-SKEW-023:setI", "SR-PS-SKEW-024:setI", "SR-PS-SKEW-025:setI", "SR-PS-SKEW-026:setI", "SR-PS-SKEW-027:setI", "SR-PS-SKEW-031:setI", "SR-PS-SKEW-032:setI", "SR-PS-SKEW-033:setI", "SR-PS-SKEW-034:setI", "SR-PS-SKEW-035:setI", "SR-PS-SKEW-036:setI", "SR-PS-SKEW-037:setI", "SR-PS-SKEW-041:setI", "SR-PS-SKEW-042:setI", "SR-PS-SKEW-043:setI", "SR-PS-SKEW-044:setI", "SR-PS-SKEW-045:setI", "SR-PS-SKEW-046:setI", "SR-PS-SKEW-047:setI", "SR-PS-SKEW-051:setI", "SR-PS-SKEW-052:setI", "SR-PS-SKEW-053:setI", "SR-PS-SKEW-054:setI", "SR-PS-SKEW-055:setI", "SR-PS-SKEW-056:setI", "SR-PS-SKEW-057:setI", "SR-PS-SKEW-061:setI", "SR-PS-SKEW-062:setI", "SR-PS-SKEW-063:setI", "SR-PS-SKEW-064:setI", "SR-PS-SKEW-065:setI", "SR-PS-SKEW-066:setI", "SR-PS-SKEW-067:setI", "SR-PS-SKEW-071:setI", "SR-PS-SKEW-072:setI", "SR-PS-SKEW-073:setI", "SR-PS-SKEW-074:setI", "SR-PS-SKEW-075:setI", "SR-PS-SKEW-076:setI", "SR-PS-SKEW-077:setI", "SR-PS-SKEW-081:setI", "SR-PS-SKEW-082:setI", "SR-PS-SKEW-083:setI", "SR-PS-SKEW-084:setI", "SR-PS-SKEW-085:setI", "SR-PS-SKEW-086:setI", "SR-PS-SKEW-087:setI", "SR-PS-SKEW-091:setI", "SR-PS-SKEW-092:setI", "SR-PS-SKEW-093:setI", "SR-PS-SKEW-094:setI", "SR-PS-SKEW-095:setI", "SR-PS-SKEW-096:setI", "SR-PS-SKEW-097:setI", "SR-PS-SKEW-101:setI", "SR-PS-SKEW-102:setI", "SR-PS-SKEW-103:setI", "SR-PS-SKEW-104:setI", "SR-PS-SKEW-105:setI", "SR-PS-SKEW-106:setI", "SR-PS-SKEW-107:setI", "SR-PS-SKEW-111:setI", "SR-PS-SKEW-112:setI", "SR-PS-SKEW-113:setI", "SR-PS-SKEW-114:setI", "SR-PS-SKEW-115:setI", "SR-PS-SKEW-116:setI", "SR-PS-SKEW-117:setI", "SR-PS-SKEW-121:setI", "SR-PS-SKEW-122:setI", "SR-PS-SKEW-123:setI", "SR-PS-SKEW-124:setI", "SR-PS-SKEW-125:setI", "SR-PS-SKEW-126:setI", "SR-PS-SKEW-127:setI", "SR-PS-SKEW-131:setI", "SR-PS-SKEW-132:setI", "SR-PS-SKEW-133:setI", "SR-PS-SKEW-134:setI", "SR-PS-SKEW-135:setI", "SR-PS-SKEW-136:setI", "SR-PS-SKEW-137:setI", "SR-PS-SKEW-141:setI", "SR-PS-SKEW-142:setI", "SR-PS-SKEW-143:setI", "SR-PS-SKEW-144:setI", "SR-PS-SKEW-145:setI", "SR-PS-SKEW-146:setI", "SR-PS-SKEW-147:setI", "SR-PS-SKEW-151:setI", "SR-PS-SKEW-152:setI", "SR-PS-SKEW-153:setI", "SR-PS-SKEW-154:setI", "SR-PS-SKEW-155:setI", "SR-PS-SKEW-156:setI", "SR-PS-SKEW-157:setI", "SR-PS-SKEW-161:setI", "SR-PS-SKEW-162:setI", "SR-PS-SKEW-163:setI", "SR-PS-SKEW-164:setI", "SR-PS-SKEW-165:setI", "SR-PS-SKEW-166:setI", "SR-PS-SKEW-167:setI", "SR-PS-SKEW-171:setI", "SR-PS-SKEW-172:setI", "SR-PS-SKEW-173:setI", "SR-PS-SKEW-174:setI", "SR-PS-SKEW-175:setI", "SR-PS-SKEW-176:setI", "SR-PS-SKEW-177:setI", "SR-PS-SKEW-181:setI", "SR-PS-SKEW-182:setI", "SR-PS-SKEW-183:setI", "SR-PS-SKEW-184:setI", "SR-PS-SKEW-185:setI", "SR-PS-SKEW-186:setI", "SR-PS-SKEW-187:setI", "SR-PS-SKEW-191:setI", "SR-PS-SKEW-192:setI", "SR-PS-SKEW-193:setI", "SR-PS-SKEW-194:setI", "SR-PS-SKEW-195:setI", "SR-PS-SKEW-196:setI", "SR-PS-SKEW-197:setI", "SR-PS-SKEW-201:setI", "SR-PS-SKEW-202:setI", "SR-PS-SKEW-203:setI", "SR-PS-SKEW-204:setI", "SR-PS-SKEW-205:setI", "SR-PS-SKEW-206:setI", "SR-PS-SKEW-207:setI", "SR-PS-SKEW-211:setI", "SR-PS-SKEW-212:setI", "SR-PS-SKEW-213:setI", "SR-PS-SKEW-214:setI", "SR-PS-SKEW-215:setI", "SR-PS-SKEW-216:setI", "SR-PS-SKEW-217:setI", "SR-PS-SKEW-221:setI", "SR-PS-SKEW-222:setI", "SR-PS-SKEW-223:setI", "SR-PS-SKEW-224:setI", "SR-PS-SKEW-225:setI", "SR-PS-SKEW-226:setI", "SR-PS-SKEW-227:setI", "SR-PS-SKEW-231:setI", "SR-PS-SKEW-232:setI", "SR-PS-SKEW-233:setI", "SR-PS-SKEW-234:setI", "SR-PS-SKEW-235:setI", "SR-PS-SKEW-236:setI", "SR-PS-SKEW-237:setI", "SR-PS-SKEW-241:setI", "SR-PS-SKEW-242:setI", "SR-PS-SKEW-243:setI", "SR-PS-SKEW-244:setI", "SR-PS-SKEW-245:setI", "SR-PS-SKEW-246:setI", "SR-PS-SKEW-247:setI", "SR-RF2-LLRF:setGapVoltage", "SR-RF2-LLRF:setStationPhase", "SR-RF3-LLRF:setGapVoltage", "SR-RF3-LLRF:setStationPhase", "SR-PS-DMB09-Q1:setI", "SR-PS-DMB09-Q2:setI", "SR-PS-DMB09-Q3:setI", "SR-PS-DMB25-Q1:setI", "SR-PS-DMB25-Q2:setI", "SR-PS-DMB25-Q3:setI", "SR-PS-DMB41-Q1:setI", "SR-PS-DMB41-Q2:setI", "SR-PS-DMB41-Q3:setI", "SR-PS-DMB09-HC1:setI", "SR-PS-DMB09-HC2:setI", "SR-PS-DMB09-VC1:setI", "SR-PS-DMB09-VC2:setI", "SR-PS-DMB25-HC1:setI", "SR-PS-DMB25-HC2:setI", "SR-PS-DMB25-VC1:setI", "SR-PS-DMB25-VC2:setI", "SR-PS-DMB41-HC1:setI", "SR-PS-DMB41-HC2:setI", "SR-PS-DMB41-VC1:setI", "SR-PS-DMB41-VC2:setI", "SR-ID-IU22-05:setGap", "SR-ID-IU22A-09:setGap", "SR-ID-IU22B-09:setGap", "SR-ID-IUT22-21:setGap", "SR-ID-IU22-23:setGap", "SR-ID-IU22A-25:setGap", "SR-ID-IU22B-25:setGap", "SR-ID-EPU48A-41:setGap", "SR-ID-EPU48A-41:setPhase", "SR-ID-EPU48B-41:setGap", "SR-ID-EPU48B-41:setPhase", "SR-ID-EPU46-45:setGap", "SR-ID-EPU46-45:setPhase", "SR-ID-IUT22-21:setGapTaper", "SR-ID-EPU48PS-41:setGap", "SR-ID-IU22-05:gapMotorOff", "SR-ID-IU22A-09:gapMotorOff", "SR-ID-IU22B-09:gapMotorOff", "SR-ID-IUT22-21:gapMotorOff", "SR-ID-IU22-23:gapMotorOff", "SR-ID-IU22A-25:gapMotorOff", "SR-ID-IU22B-25:gapMotorOff", "SR-ID-EPU48A-41:gapMotorOff", "SR-ID-EPU48B-41:gapMotorOff", "SR-ID-EPU46-45:gapMotorOff", "SR-ID-EPU48A-41:phaseMotorOff", "SR-ID-EPU48B-41:phaseMotorOff", "SR-ID-EPU46-45:phaseMotorOff", "SR-DI-FOFB-H:setStatus", "SR-DI-FOFB-V:setStatus", "IGPF:TPSX:FBCTRL", "IGPF:TPSY:FBCTRL", "TPS-SR-022:bpm3:ilk:enabled", "SR-DI-ANGLE-ILK:StatusX", "SR-DI-ANGLE-ILK:StatusY", "SR-DI-RF-FB:setStatus", "SR-ID-EPU48-TFF:status", "SR-ID-EPU48-CFF:status", "SR-ID-EPU46-TFF:status", "SR-ID-EPU46-CFF:status", "TI-INJ-PROC:TopupHiLowStart"]
  out "result":string="Beam Trip Events \nTatal Counts: 0"
  in  "last ? Hrs":dbl=12.0 min=1.0 max=24.0 step=1.0
  in  "Trip Evt B":bool
  in  "Show Check list Button":bool=TRUE
  in  "View Diff Button":bool
  in  "Save Lattice Button":bool
  in  "Refresh B":bool
  out "x = y?":bool
  out "NOW time":string="15:45:10"
  out "NOW date":string="2017/10/28"
  in  "Save Button":bool
  out "error out 3":errorcluster
  in  "stop":bool
  out "time kickeron":string="15:43:52"
  out "date kickeron":string="2017/10/28"
  out "Orbit ILK(A)":bool
  out "Orbit INT. Ang Active":bool
  out "Orbit INT.Ang. On":bool
  out "Orbit INT. Pos Active":bool
  out "Orbit INT.Pos. On":bool
  in  "Copy Button":bool
  in  "Print Button":bool
  in  "Help Button":bool
  in  "Open Button":bool
  # "TPS OP Handover Information"
  # "Others"
  # "Additional Functions"
  # "Time："
  # "follow"
  # "歷史電流圖\ntrip次數?\n輻射劑量?\n平均氣壓\n目前最高累計劑量\n最近一次觸發時BR電流及WCM數值"
  # "Valve  Status"
  # "TFF"
  # "CFF"
  # "SM Status"
  # "TPS Operational Handover Information v1.4.7"
  # "SR Status"
  # "Feedback"
  # "Pulse Mag"
  # "LINAC"
  # "x8(ns)"
  # "x2(ns)"
  # "x0.01(ns)"
  # "RF Status"
  # "Hz"
  # "(kV)"
  # "(kV)"
  # "Changeliang@LOP.NSRRC"
  # "BR Fill Pattern"
  # "SR Fill Pattern"
  # "Lattice Files in Using"
  # "ID &Beamline [R]"
  # "Gap\nmm"
  # "Motor"
  # "Phase"
  # "FE/Hutch"
  # "Mode"
  # "Phase\nShifter"
  # "XBPM1X\num"
  # "XBPM1Y\num"
  # "XBPM2X\num"
  # "XBPM2Y\num"
  # "Note"
  # "05"
  # "09"
  # "Taper(enc)"
  # "21"
  # "23"
  # "25"
  # "41"
  # "45"
  # "SR Orbit"
  # "BPMX"
  # "BPMY"
  # "SR Beam Current History"
  # "ns"
  # "threshold:0.05mA"
  # "Adjusted History\n#Note: This file recorded PVs(set values) that were changed during this time.\n#(RF frequency was not recorded in this file)"
  # "Event Time"
  # "PV_name"
  # "Ori_Value"
  # "New_Value"
  # "hrs"
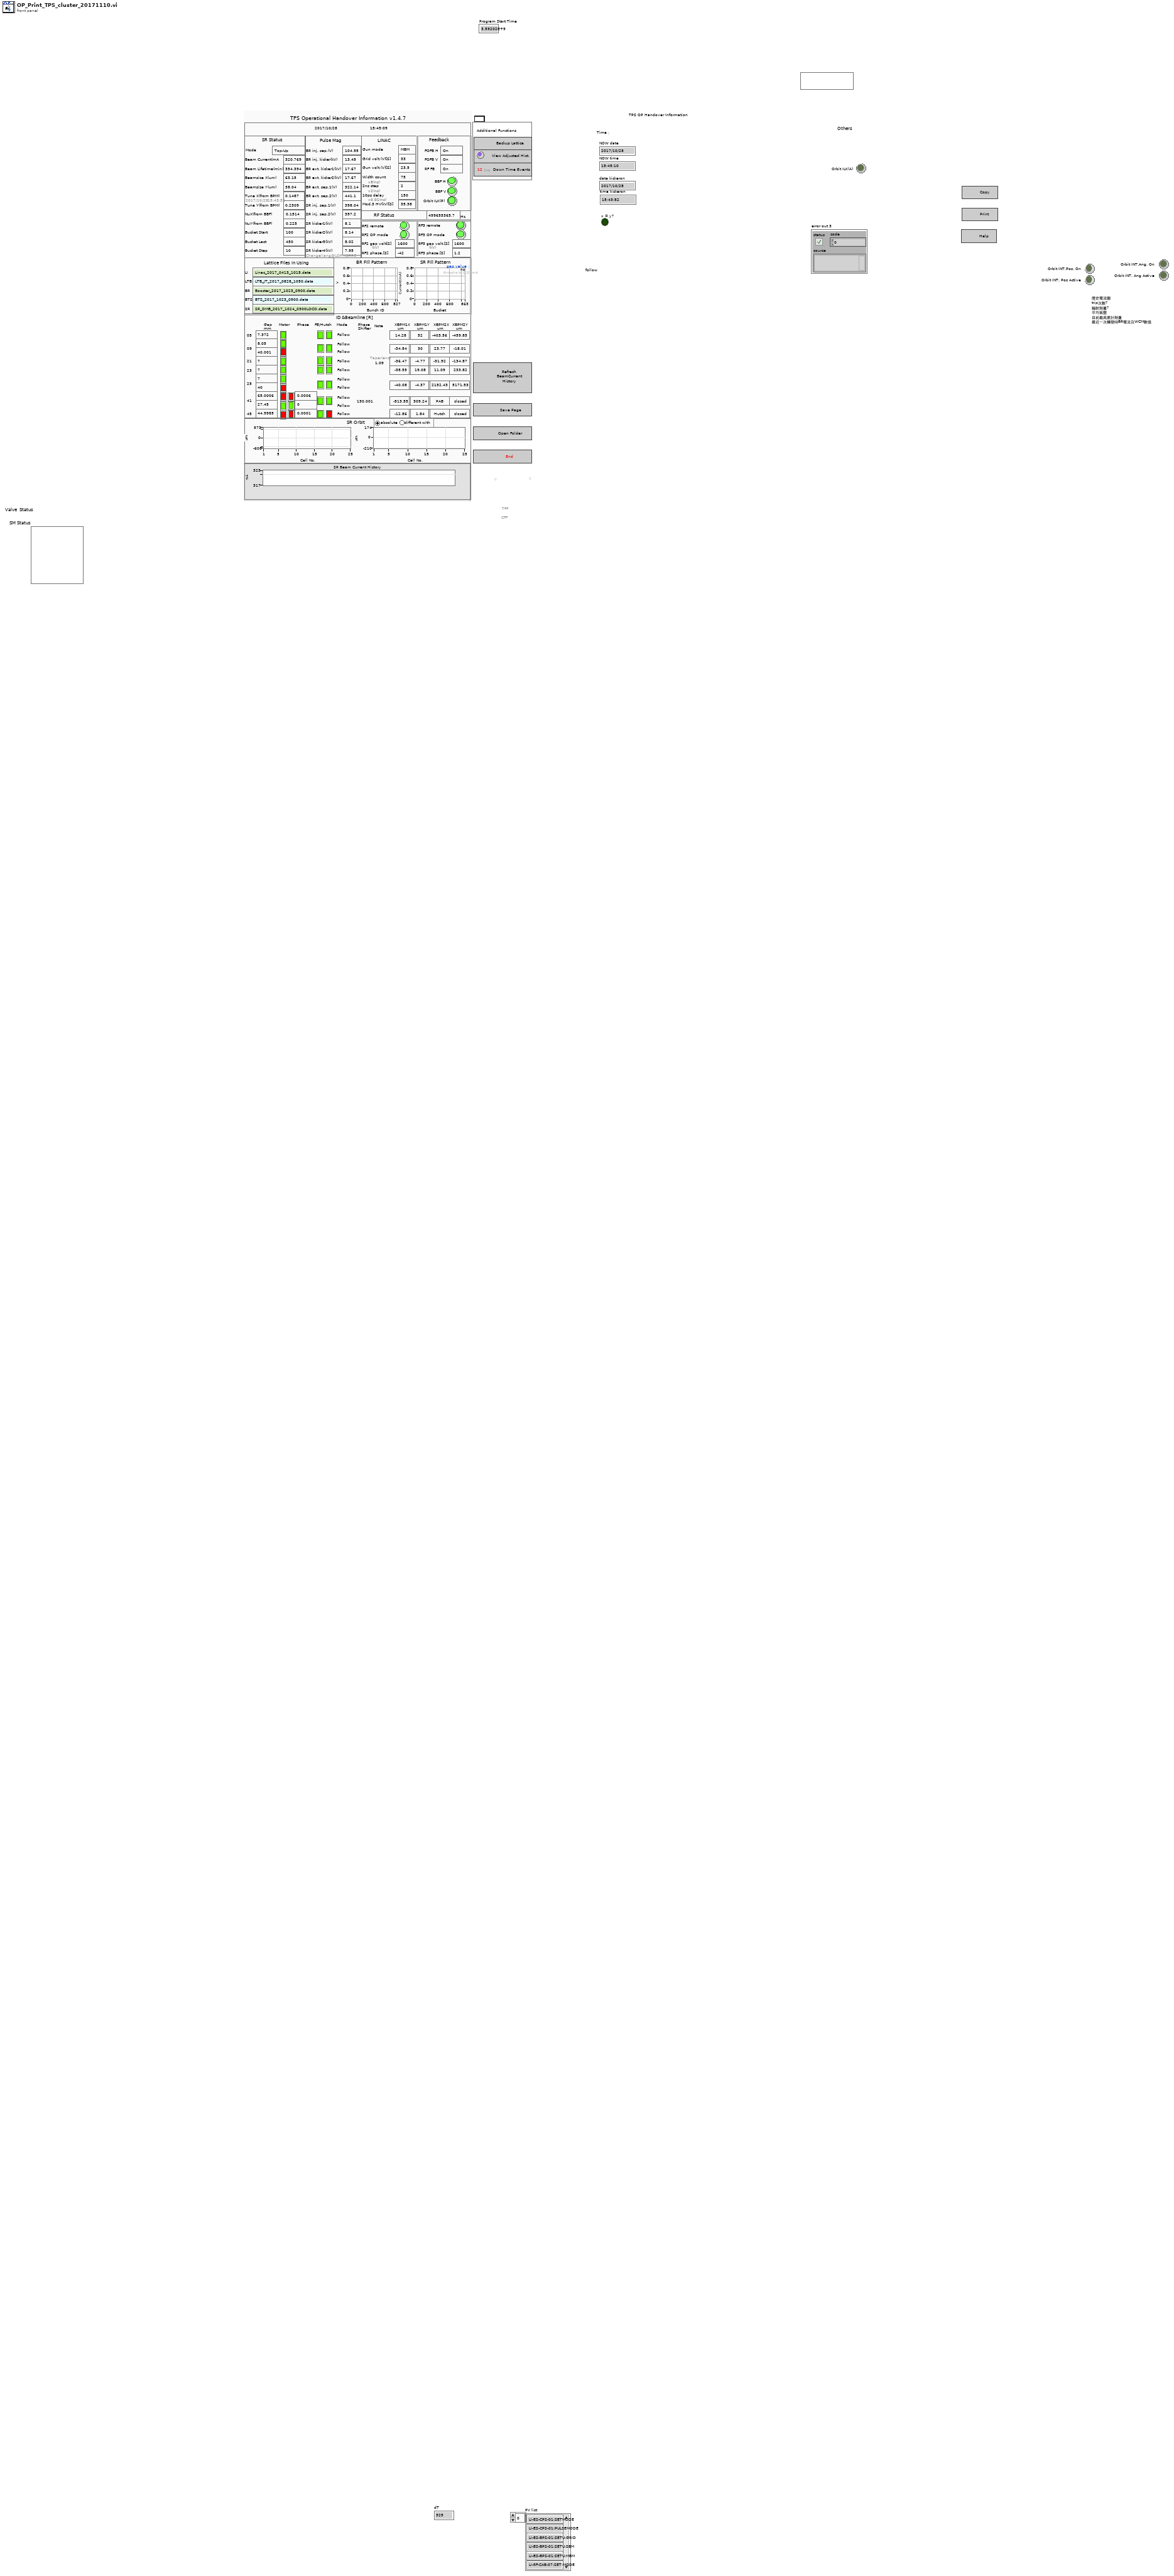
[diagram p1: front panel]
types:
  T1 = cluster{"SR Fill Pattern":dbl[], "Beam Current(mA":dbl, "Beam Lifetime(min)":dbl, "Beamsize X(um)":dbl, "Beamsize Y(um)":dbl, "Tune X(from BPM)":dbl, "Tune Y(from BPM)":dbl, "Mode":string, "NuX(from BBF) ":dbl, "NuY(from BBF)":dbl, "IU22-23gap(R)":dbl, "IU22-05gap(R)":dbl, "IU22-05M":bool, "IU22A-09gap(R)":dbl, "IU22A-09M":bool, "IU22B-09gap(R)":dbl, "IU22B-09M":bool, "IUT22-21gap(R)":dbl, "IUT22-21M":bool, "IU22-23M":bool, "IU22A-25gap(R)":dbl, "IU22A-25M":bool, "IU22B-25gap(R)":dbl, "IU22B-25M":bool, "EPU48A-41gap(R)":dbl, "EPU48A-41gM":bool, "EPU48B-41gap(R)":dbl, "EPU48B-41gM":bool, "EPU46-45gap(R)":dbl, "EPU46-45gM":bool, "EPU48A-41phase(R)":dbl, "EPU48B-41phase(R)":dbl, "EPU46-45phase(R)":dbl, "Grid volt.(V)[S]":dbl, "Gun mode":string, "Mod.3 HV(kV)[S]":dbl, "SR":string, "BR":string, "LI":string, "LTB":string, "BTS":string, "RF2 remote":bool, "RF2 OP mode":bool, "RF2 phase.[S]":dbl, "RF Freq.(s)":dbl, "RF2 gap volt[S]":dbl, "RF3 remote":bool, "RF3 OP mode":bool, "RF3 phase.[S]":dbl, "RF3 gap volt.[S]":dbl, "BBF V":bool, "BBF H":bool, "BR ext. kicker1(kV)":dbl, "BR ext. kicker2(kV)":dbl, "BR ext. sep.1(V)":dbl, "BR ext. sep.2(V)":dbl, "BR inj. sep.(V)":dbl, "BR inj. kicker(kV)":dbl, "SR kicker4(kV)":dbl, "SR kicker3(kV)":dbl, "SR kicker2(kV)":dbl, "SR kicker1(kV)":dbl, "SR inj. sep.2(V)":dbl, "SR inj. sep.1(V)":dbl, "Bucket Start":dbl, "Bucket Last":dbl, "Bucket Step":dbl, "Orbit ILK(P)":bool, "IU22-05 Hutch Enable":bool, "IU22A-09M Hutch Enable":bool, "IUT22-21M Hutch Enable":bool, "IU22-23M Hutch Enable":bool, "IU22A-25M Hutch Enable":bool, "EPU48A-41M Hutch Enable":bool, "EPU46-45M Hutch Enable":bool, "EPU46-45 FE Enable":bool, "EPU48A-41 FE Enable":bool, "IU22A-25 FE Enable":bool, "IU22-23 FE Enable":bool, "IUT22-21 FE Enable":bool, "IU22A-09 FE Enable":bool, "IU22-05 FE Enable":bool, "EPU48A-41pM":bool, "EPU48B-41pM":bool, "EPU46-45pM":bool, "Gun volt.(V)[S]":dbl, "Width count":dbl, "2ns step":dbl, "10ps delay":dbl, "phase shifter":dbl, "Taper":dbl, "05XBPMX 1":dbl, "09XBPMX 1":dbl, "21XBPMX 1":dbl, "23XBPMX 1":dbl, "25XBPMX 1":dbl, "41XBPMX 1":dbl, "45XBPMX 1":dbl, "05XBPMY 1":dbl, "09XBPMY 1":dbl, "21XBPMY 1":dbl, "23XBPMY 1":dbl, "25XBPMY 1":dbl, "41XBPMY 1":dbl, "45XBPMY 1":dbl, "FOFB H":string, "FOFB V":string, "time string":string, "date":string, "date (last kicker ON)":string, "time string (last kicker ON)":string, "Radio Buttons 2":enum32{"absolute", "different with"}, "09XBPMX 2":string, "09XBPMY 2":string, "05XBPMY 2":string, "05XBPMX 2":string, "21XBPMY 2":string, "21XBPMX 2":string, "23XBPMY 2":string, "23XBPMX 2":string, "25XBPMY 2":string, "25XBPMX 2":string, "41XBPMY 2":string, "41XBPMX 2":string, "45XBPMX 2":string, "45XBPMY 2":string, "05 mode":string, "09A mode":string, "09B mode":string, "21 mode":string, "23 mode":string, "25A mode":string, "25B mode":string, "41A mode":string, "41B mode":string, "46 mode":string, "BeamCurrent History":cluster{"BPM NO.  1_172":dbl[], dbl[]}, "SR Beam Current in            hours":dbl, "RF FB":string, "BPMX Graph 2":cluster{"Array of X axis  平均分配至各段":dbl[], dbl[]}, "BPMY Graph 2":cluster{"Array of X axis  平均分配至各段":dbl[], dbl[]}, "gap value：":i32, "BR Fill Pattern":dbl[], "time string (last INJ) ":string}
  T2 = typedef "NI_Database_API.lvlib/Conn ObjectReference.ctl" = refnum<k1>
  T3 = typedef "NI_Database_API.lvlib/Rec ObjectReference.ctl" = refnum<k1>
  T4 = typedef "imagedata.ctl" = cluster{"image type":i32, "image depth":i32, "image":u8[], "mask":u8[], "colors":u32[], "Rectangle":cluster{"left":i16, "top":i16, "right":i16, "bottom":i16}}
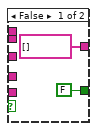
[diagram p3: hidden frame]
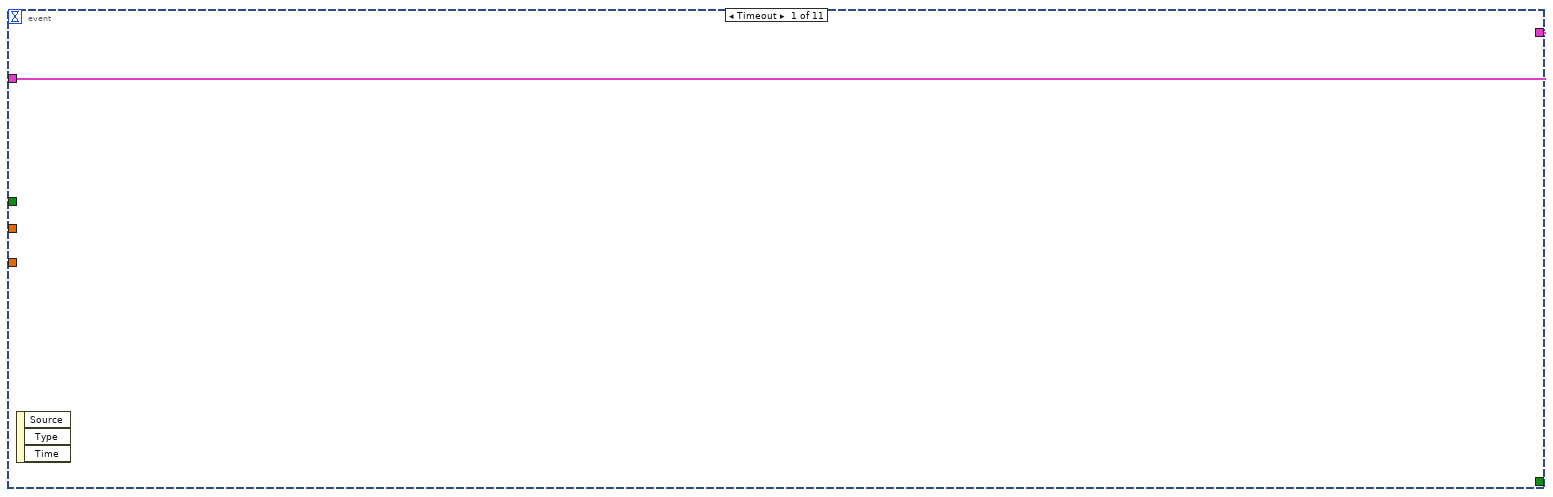
[diagram p6: hidden frame]
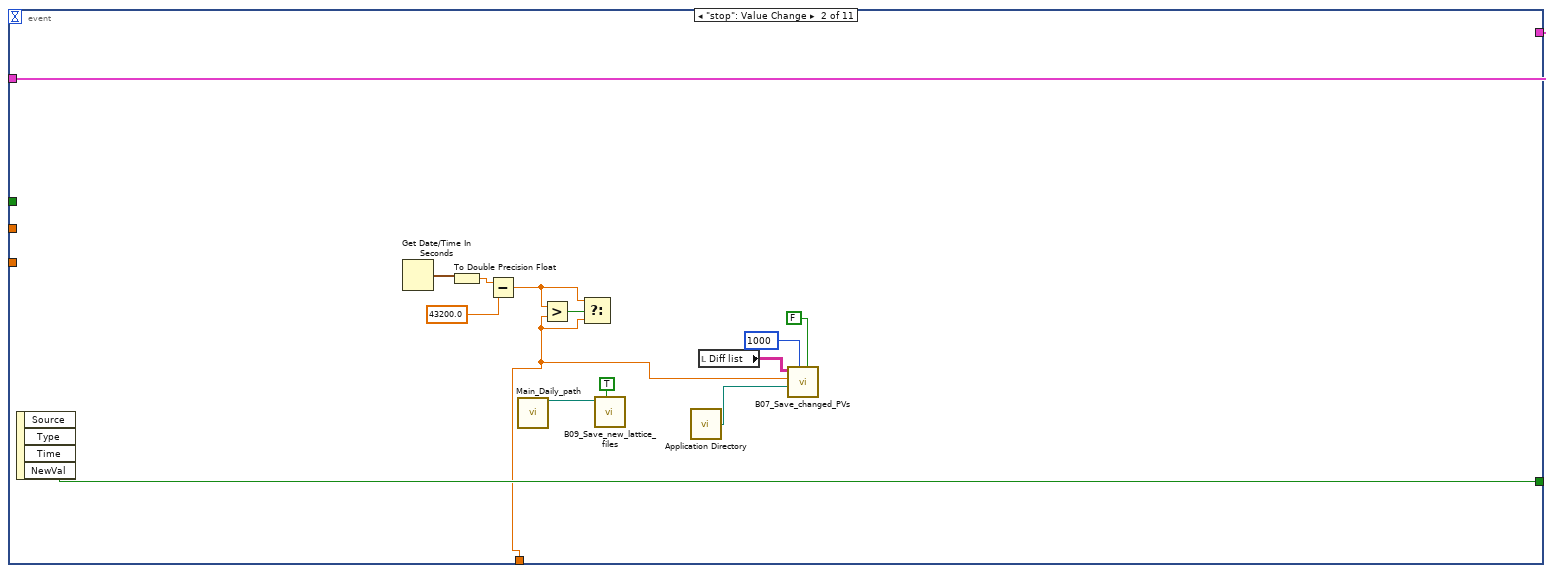
[diagram p7: hidden frame]
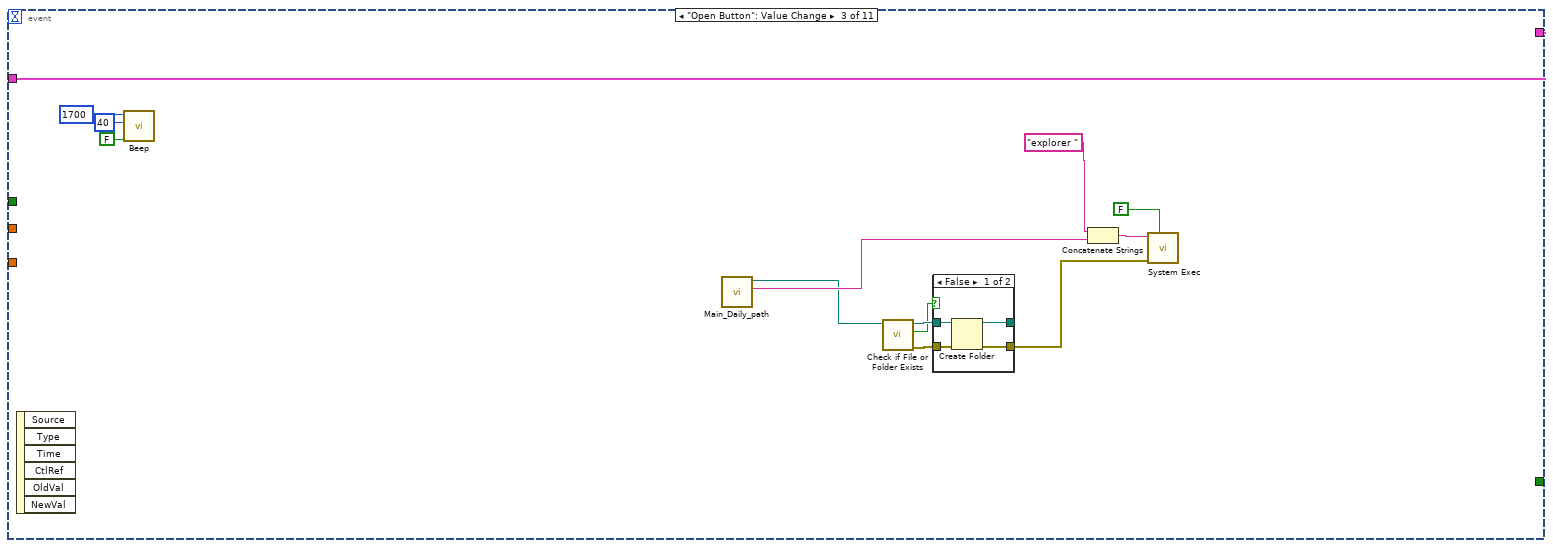
[diagram p8: hidden frame]
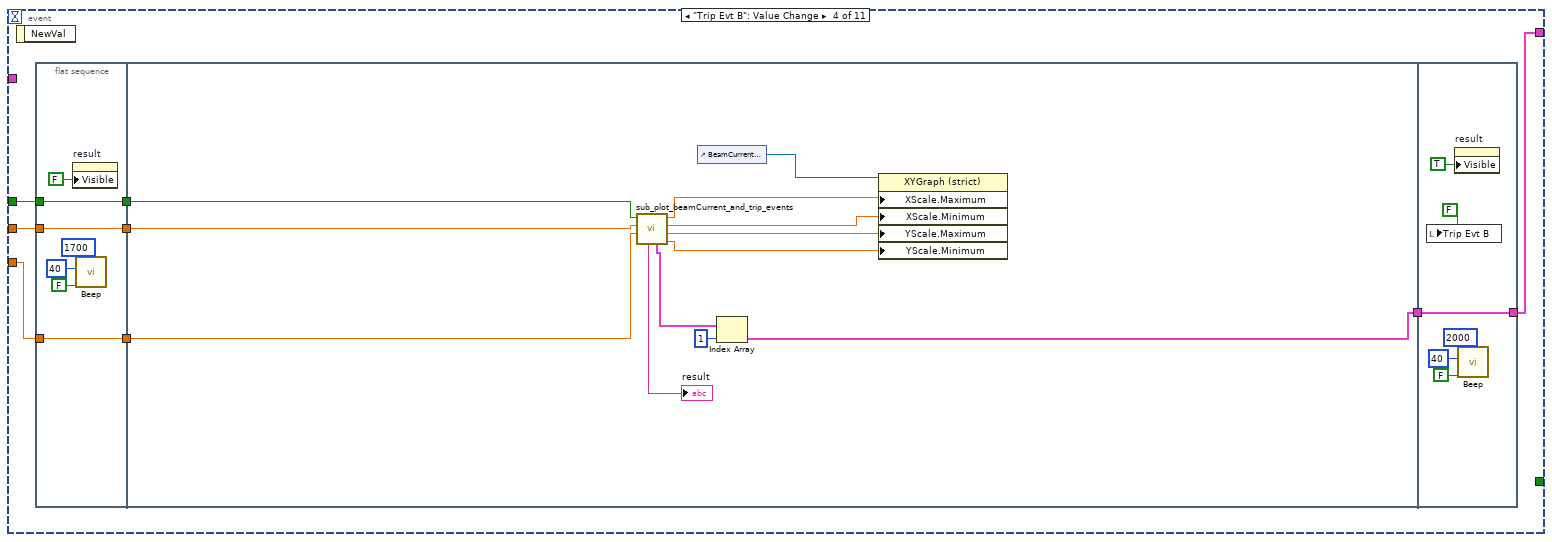
[diagram p10: hidden frame]
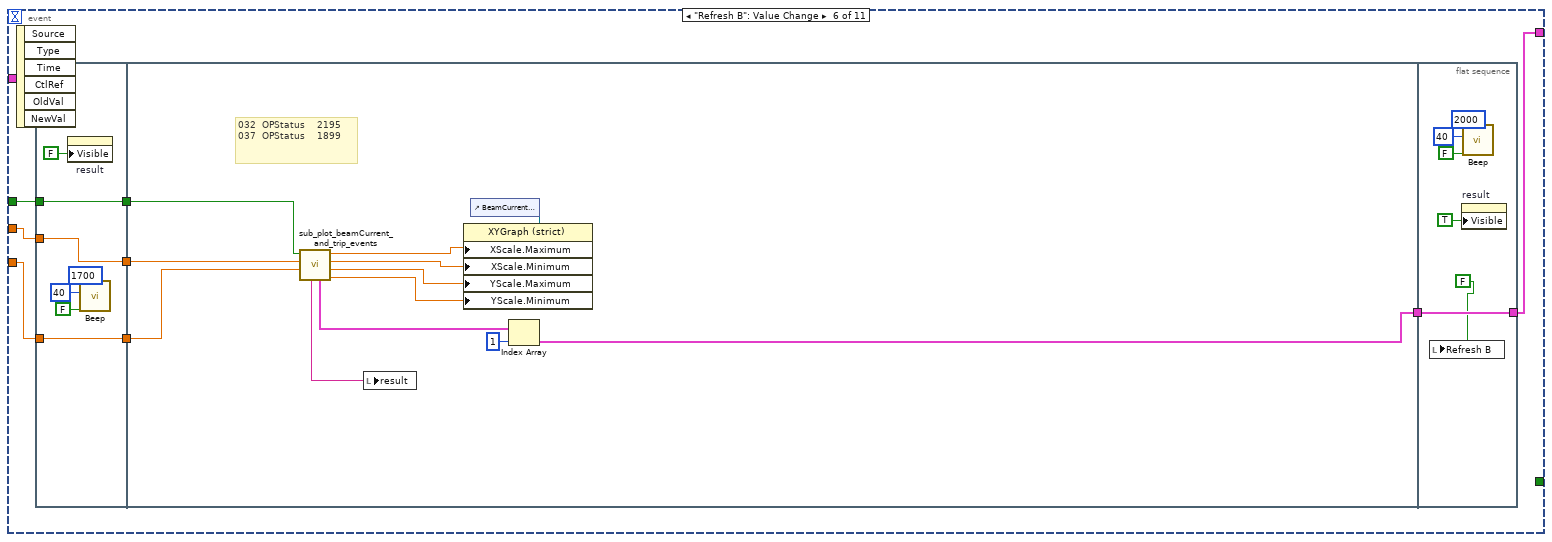
[diagram p11: hidden frame]
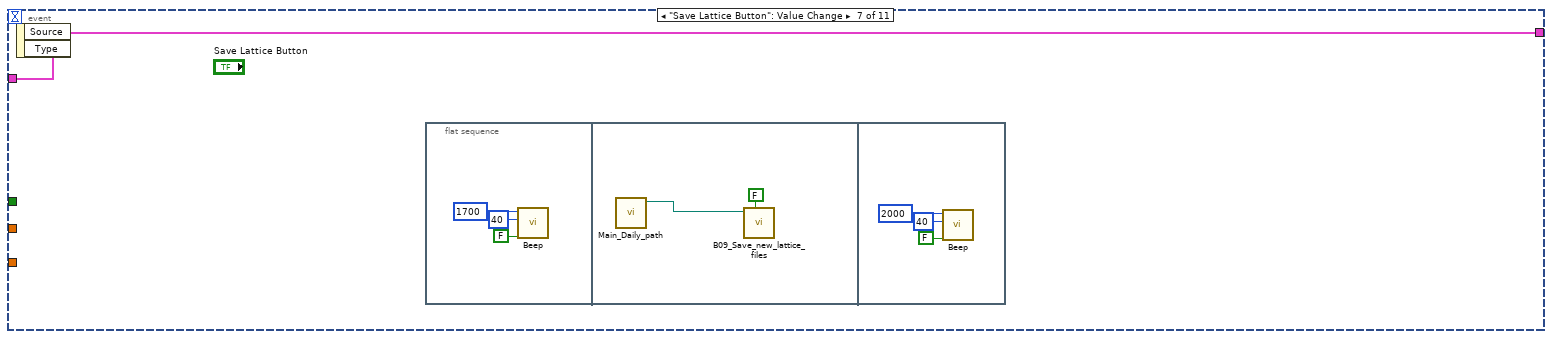
[diagram p12: hidden frame]
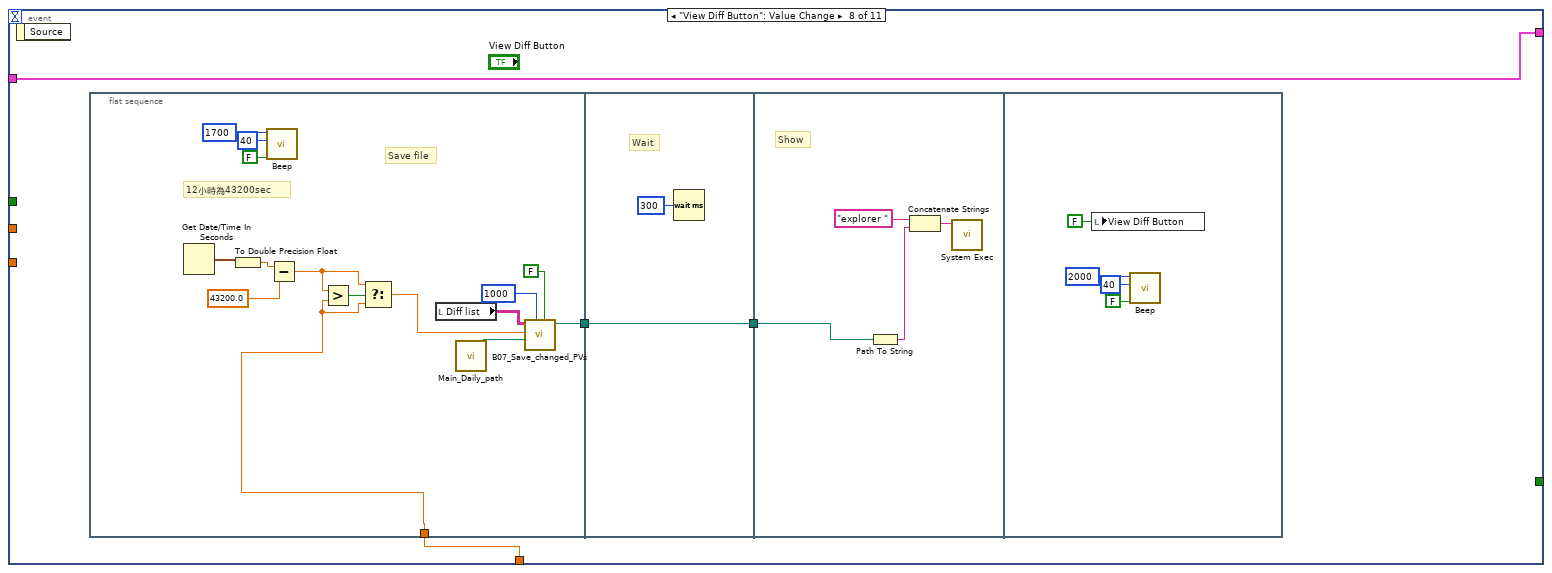
[diagram p13: hidden frame]
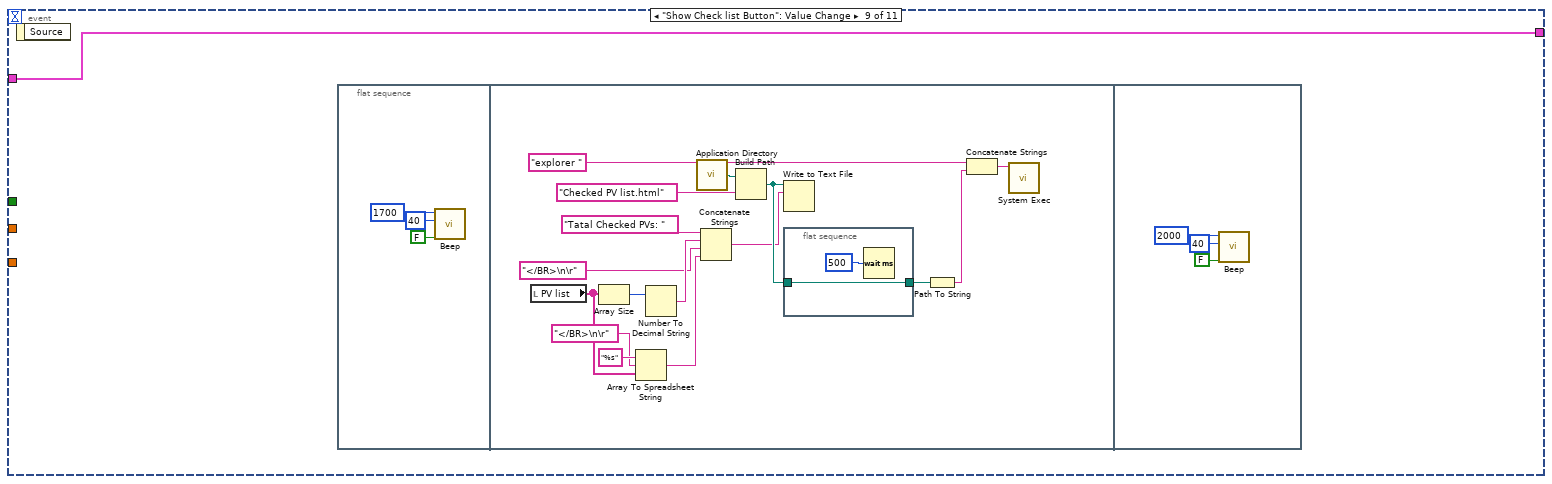
[diagram p14: hidden frame]
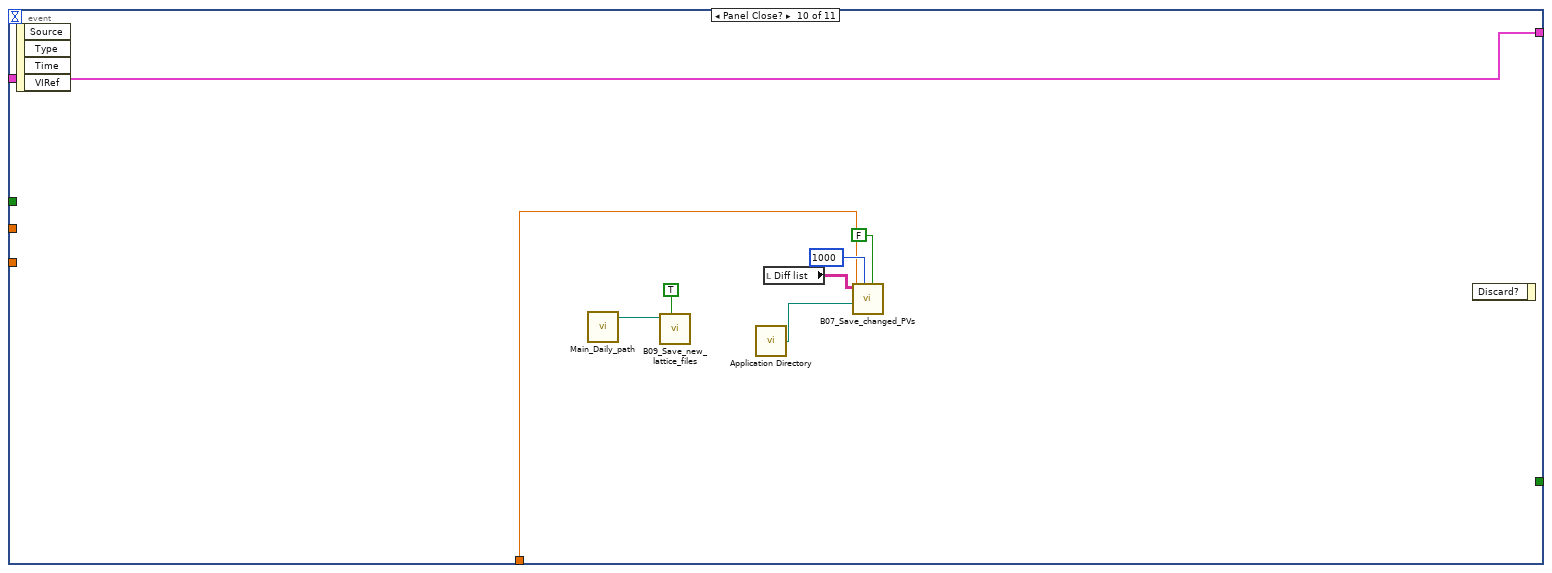
[diagram p15: hidden frame]
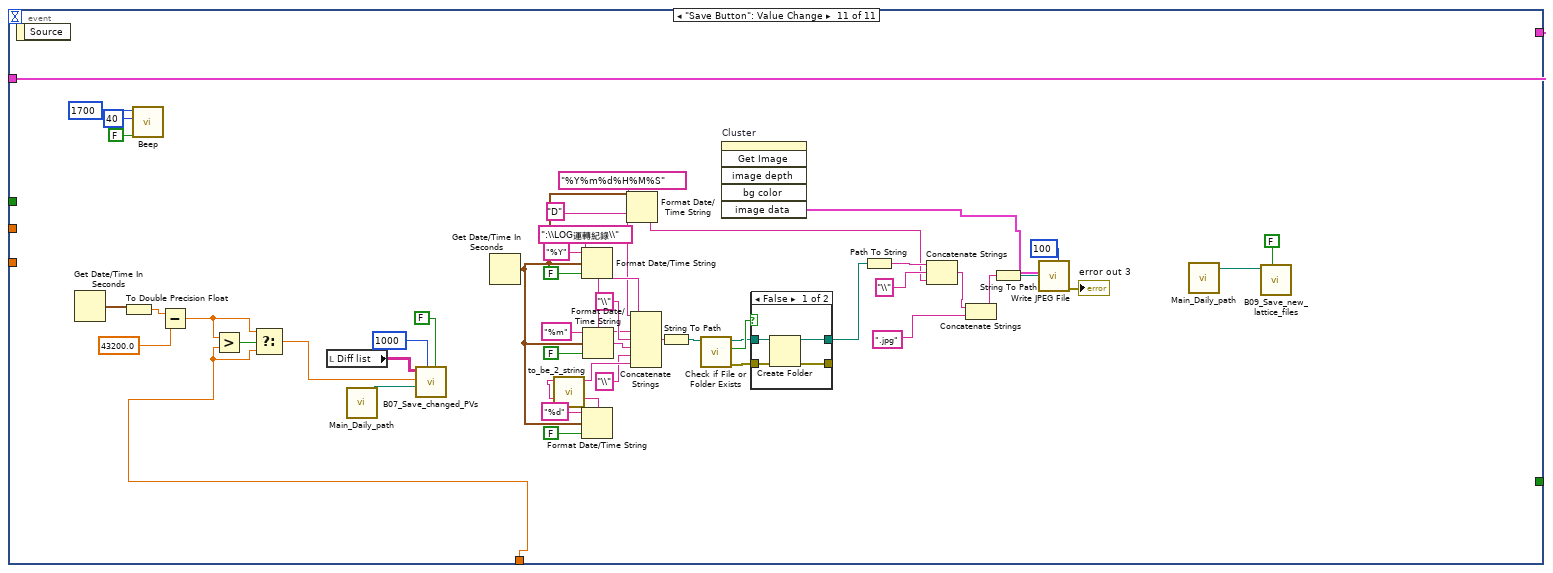
[diagram p16: hidden frame]
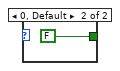
[diagram p18: hidden frame]
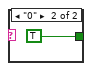
[diagram p19: hidden frame]
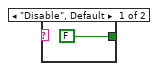
[diagram p20: hidden frame]
diagram:
  w1 = string[] ["BR-PS-HC-101:setI", "BR-PS-HC-102:setI", "BR-PS-HC-103:setI", "BR-PS-HC-104:setI", "BR-PS-HC-105:setI", "BR-PS-HC-106:setI", "BR-PS-HC-107:setI", "BR-PS-HC-108:setI", "BR-PS-HC-109:setI", "BR-PS-HC-110:setI", "BR-PS-HC-201:setI", "BR-PS-HC-202:setI", "BR-PS-HC-203:setI", "BR-PS-HC-204:setI", "BR-PS-HC-205:setI", "BR-PS-HC-206:setI", "BR-PS-HC-207:setI", "BR-PS-HC-208:setI", "BR-PS-HC-209:setI", "BR-PS-HC-210:setI", "BR-PS-HC-301:setI", "BR-PS-HC-302:setI", "BR-PS-HC-303:setI", "BR-PS-HC-304:setI", "BR-PS-HC-305:setI", "BR-PS-HC-306:setI", "BR-PS-HC-307:setI", "BR-PS-HC-308:setI", "BR-PS-HC-309:setI", "BR-PS-HC-310:setI", "BR-PS-HC-401:setI", "BR-PS-HC-402:setI", "BR-PS-HC-403:setI", "BR-PS-HC-404:setI", "BR-PS-HC-405:setI", "BR-PS-HC-406:setI", "BR-PS-HC-407:setI", "BR-PS-HC-408:setI", "BR-PS-HC-409:setI", "BR-PS-HC-410:setI", "BR-PS-HC-501:setI", "BR-PS-HC-502:setI", "BR-PS-HC-503:setI", "BR-PS-HC-504:setI", "BR-PS-HC-505:setI", "BR-PS-HC-506:setI", "BR-PS-HC-507:setI", "BR-PS-HC-508:setI", "BR-PS-HC-509:setI", "BR-PS-HC-510:setI", "BR-PS-HC-601:setI", "BR-PS-HC-602:setI", "BR-PS-HC-603:setI", "BR-PS-HC-603a:setI", "BR-PS-HC-604:setI", "BR-PS-HC-605:setI", "BR-PS-HC-606:setI", "BR-PS-HC-606a:setI", "BR-PS-HC-607:setI", "BR-PS-HC-608:setI", "BR-PS-HC-609:setI", "BR-PS-HC-610:setI", "BR-PS-VC-101:setI", "BR-PS-VC-102:setI", "BR-PS-VC-103:setI", "BR-PS-VC-104:setI", "BR-PS-VC-105:setI", "BR-PS-VC-106:setI", "BR-PS-VC-201:setI", "BR-PS-VC-202:setI", "BR-PS-VC-203:setI", "BR-PS-VC-204:setI", "BR-PS-VC-205:setI", "BR-PS-VC-206:setI", "BR-PS-VC-301:setI", "BR-PS-VC-302:setI", "BR-PS-VC-303:setI", "BR-PS-VC-304:setI", "BR-PS-VC-305:setI", "BR-PS-VC-306:setI", "BR-PS-VC-401:setI", "BR-PS-VC-402:setI", "BR-PS-VC-403:setI", "BR-PS-VC-404:setI", "BR-PS-VC-405:setI", "BR-PS-VC-406:setI", "BR-PS-VC-501:setI", "BR-PS-VC-502:setI", "BR-PS-VC-503:setI", "BR-PS-VC-504:setI", "BR-PS-VC-505:setI", "BR-PS-VC-506:setI", "BR-PS-VC-601:setI", "BR-PS-VC-602:setI", "BR-PS-VC-602a:setI", "BR-PS-VC-603:setI", "BR-PS-VC-604:setI", "BR-PS-VC-604a:setI", "BR-PS-VC-605:setI", "BR-PS-VC-606:setI", "BR-PS-VC-100a:setI", "BR-PS-SD:setI", "BR-PS-SF:setI", "cpsc_027:AO:SLOW_SET:CH:1", "BR-RF-LLRF:setStationPhase", "TI-INJ-PROC:setTinj", "BR-PS-INJ-SE:setHV", "CPCIPM-TI-EVR:Pulse1DelaySet", "BR-PS-INJ-KI:setHV", "CPCIPM-TI-EVR:Pulse2DelaySet", "BR-PS-QF:setWfDC", "BR-PS-QM:setWfDC", "BR-PS-Q1:setWfDC", "BR-PS-Q2:setWfDC", "BR-PS-BEND:setWfDC"]  # PV nanes (BR_without_Wf, cpsc_037:AO:SLOW_SET:CH:3)
  w2 = string[] ["LI-ES-CPS-01:SETMODE", "LI-ES-CPS-01:PULSEMODE", "LI-ES-BPS-01:SETU:GRID", "LI-ES-BPS-01:SETU:SBM", "LI-ES-BPS-01:SETU:MBM", "LI-RF-CAB-07:SET:MODE", "LI-RF-HVP-11:SET:U", "LI-RF-CAB-09:SET:MODE", "LI-RF-HVP-21:SET:U", "LI-RF-HVP-31:SET:U", "LI-RF-WGA-01:SET:POS", "LI-RF-WGA-02:SET:POS", "LI-RF-WGA-03:SET:POS", "LI-RF-SFT-01:SET:POS", "LI-RF-SFT-02:SET:POS", "LI-RF-SFT-03:SET:POS", "LI-RF-CTR-01:ES:SET:DEG", "LI-RF-CTR-01:SP:SET:DEG", "LI-RF-CTR-01:K123:SET:DEG", "LI-RF-CTR-01:K1:SET:DEG", "LI-RF-CTR-01:K3:SET:DEG", "LI-RF-AMP-01:SET:PWR", "LI-RF-AMP-02:SET:PWR", "LI-MA-SPS-01:SET:I", "LI-MA-SPS-02:SET:I", "LI-MA-SPS-03:SET:I", "LI-MA-SPS-04:SET:I", "LI-MA-SPS-05:SET:I", "LI-MA-SPS-06:SET:I", "LI-MA-SPS-07:SET:I", "LI-MA-SPS-08:SET:I", "LI-MA-SPS-09:SET:I", "LI-MA-SPS-10:SET:I", "LI-MA-SPS-11:SET:I", "LI-MA-SPS-12:SET:I", "LI-MA-SPS-13:SET:I", "LI-MA-SPS-14:SET:I", "LI-MA-SPS-15:SET:I", "LI-MA-SPS-16:SET:I", "LI-MA-STP-01:SET:I", "LI-MA-STP-02:SET:I", "LI-MA-STP-03:SET:I", "LI-MA-STP-04:SET:I", "LI-MA-STP-05:SET:I", "LI-MA-STP-06:SET:I", "LI-MA-STP-07:SET:I", "LI-MA-STP-08:SET:I", "LI-MA-STP-09:SET:I", "LI-MA-STP-10:SET:I", "LI-MA-STP-11:SET:I", "LI-MA-STP-12:SET:I", "LI-MA-STP-13:SET:I", "LI-MA-STP-14:SET:I", "LI-MA-STP-15:SET:I", "LI-MA-STP-16:SET:I", "LI-MA-QPS-01:SET:I", "LI-MA-QPS-02:SET:I", "LI-MA-QPS-03:SET:I", "LI-MA-QPS-04:SET:I", "LI-MA-QPS-05:SET:I", "LI-MA-QPS-06:SET:I", "CPCITM-TI-EVRTG:Pulse7DelaySet", "CPCITM-TI-EVRTG:Pulse7WidthSet", "CPCITM-TI-EVRTG:GTX7DlySet", "CPCITM-TI-EVRTG:Pulse6DelaySet", "CPCITM-TI-EVRTG:Pulse6WidthSet", "CPCITM-TI-EVRTG:GTX6DlySet", "CPCILI-TI-EVR:Pulse2DelaySet", "CPCILI-TI-EVR:Pulse2WidthSet", "CPCILI-TI-EVR:Pulse3DelaySet", "CPCILI-TI-EVR:Pulse3WidthSet", "CPCILI-TI-EVR:Pulse4DelaySet", "CPCILI-TI-EVR:Pulse4WidthSet", "CPCILI-TI-EVR:Pulse5DelaySet", "CPCILI-TI-EVR:Pulse5WidthSet", "CPCILI-TI-EVR:Pulse6DelaySet", "CPCILI-TI-EVR:Pulse6WidthSet", "CPCILI-TI-EVR:Pulse7DelaySet", "CPCILI-TI-EVR:Pulse7WidthSet", "CPCILI-TI-EVR:Pulse8DelaySet", "CPCILI-TI-EVR:Pulse8WidthSet", "CPCILI-TI-EVR:Pulse9DelaySet", "CPCILI-TI-EVR:Pulse9WidthSet", "CPCITM-TI-EVRTG:GTX6DlySet", "CPCITM-TI-EVRTG:GTX7DlySet"]  # PV nanes(LINAC) without 3 set
  w3 = string[] ["TI-INJ-PROC:TopupHiLowStart", "TI-INJ-PROC:setBucketAddressStart", "TI-INJ-PROC:setBucketAddressLast", "TI-INJ-PROC:setBucketAddressStep", "TI-INJ-PROC:setPreCycle", "TI-INJ-PROC:setPostCycle", "TI-INJ-PROC:setBeamCurrentTopupHi", "TI-INJ-PROC:setBeamCurrentTopupLo", "TI-INJ-PROC:setSingleBunchAddr", "TI-INJ-PROC:setSingleInjCycle", "TI-INJ-PROC:setSingleBeamCurrent"]  # PV nanes(Others)
  w4 = string[] ["SR-ID-IU22-05:setECMode", "SR-ID-IU22A-09:setECMode", "SR-ID-IU22B-09:setECMode", "SR-ID-IUT22-21:setECMode", "SR-ID-IU22-23:setECMode", "SR-ID-IU22A-25:setECMode", "SR-ID-IU22B-25:setECMode", "SR-ID-EPU48A-41:setECMode", "SR-ID-EPU48B-41:setECMode", "SR-ID-EPU46-45:setECMode"]  # ID_mode
  (unwired) "cpsc_037:AO:SLOW_SET:CH:3" ("regular expression")
  w5 = string[] ["SR-DI-XPC-40:cam:AcquireTime", "SR-DI-XPC-40:cam:Gain"]  # Port40
  w6 = string[] ["LI:controlState0", "TI-INJ-PROC:trig-BRAC-ONOFF", "SR:controlState0"]  # Power Saving
  (unwired) "CPCITM-TI-EVRTG:GTX6CtrlGTXPHSet" ("regular expression")
  (unwired) "CPCITM-TI-EVRTG:GTX7CtrlGTXPHSet" ("regular expression")
  w9 = string[] ["SR-ID-IU22-05:gapMotorOff", "SR-ID-IU22A-09:gapMotorOff", "SR-ID-IU22B-09:gapMotorOff", "SR-ID-IUT22-21:gapMotorOff", "SR-ID-IU22-23:gapMotorOff", "SR-ID-IU22A-25:gapMotorOff", "SR-ID-IU22B-25:gapMotorOff", "SR-ID-EPU48A-41:gapMotorOff", "SR-ID-EPU48B-41:gapMotorOff", "SR-ID-EPU46-45:gapMotorOff", "SR-ID-EPU48A-41:phaseMotorOff", "SR-ID-EPU48B-41:phaseMotorOff", "SR-ID-EPU46-45:phaseMotorOff"]  # ID MO
  w8 = string[] ["SR-ID-IU22-05:setGap", "SR-ID-IU22A-09:setGap", "SR-ID-IU22B-09:setGap", "SR-ID-IUT22-21:setGap", "SR-ID-IU22-23:setGap", "SR-ID-IU22A-25:setGap", "SR-ID-IU22B-25:setGap", "SR-ID-EPU48A-41:setGap", "SR-ID-EPU48A-41:setPhase", "SR-ID-EPU48B-41:setGap", "SR-ID-EPU48B-41:setPhase", "SR-ID-EPU46-45:setGap", "SR-ID-EPU46-45:setPhase", "SR-ID-IUT22-21:getGapTaper", "SR-ID-EPU48PS-41:setGap", "SR-ID-IUT22-21:setGapMode"]  # PV nanes(ID gap_phase_Taper_)
  w17 = string[] ["SR-PS-BEND:setI", "SR-PS-HC-011:setI", "SR-PS-HC-012:setI", "SR-PS-HC-013:setI", "SR-PS-HC-014:setI", "SR-PS-HC-015:setI", "SR-PS-HC-016:setI", "SR-PS-HC-017:setI", "SR-PS-HC-021:setI", "SR-PS-HC-022:setI", "SR-PS-HC-023:setI", "SR-PS-HC-024:setI", "SR-PS-HC-025:setI", "SR-PS-HC-026:setI", "SR-PS-HC-027:setI", "SR-PS-HC-031:setI", "SR-PS-HC-032:setI", "SR-PS-HC-033:setI", "SR-PS-HC-034:setI", "SR-PS-HC-035:setI", "SR-PS-HC-036:setI", "SR-PS-HC-037:setI", "SR-PS-HC-041:setI", "SR-PS-HC-042:setI", "SR-PS-HC-043:setI", "SR-PS-HC-044:setI", "SR-PS-HC-045:setI", "SR-PS-HC-046:setI", "SR-PS-HC-047:setI", "SR-PS-HC-051:setI", "SR-PS-HC-052:setI", "SR-PS-HC-053:setI", "SR-PS-HC-054:setI", "SR-PS-HC-055:setI", "SR-PS-HC-056:setI", "SR-PS-HC-057:setI", "SR-PS-HC-061:setI", "SR-PS-HC-062:setI", "SR-PS-HC-063:setI", "SR-PS-HC-064:setI", "SR-PS-HC-065:setI", "SR-PS-HC-066:setI", "SR-PS-HC-067:setI", "SR-PS-HC-071:setI", "SR-PS-HC-072:setI", "SR-PS-HC-073:setI", "SR-PS-HC-074:setI", "SR-PS-HC-075:setI", "SR-PS-HC-076:setI", "SR-PS-HC-077:setI", "SR-PS-HC-081:setI", "SR-PS-HC-082:setI", "SR-PS-HC-083:setI", "SR-PS-HC-084:setI", "SR-PS-HC-085:setI", "SR-PS-HC-086:setI", "SR-PS-HC-087:setI", "SR-PS-HC-091:setI", "SR-PS-HC-092:setI", "SR-PS-HC-093:setI", "SR-PS-HC-094:setI", "SR-PS-HC-095:setI", "SR-PS-HC-096:setI", "SR-PS-HC-097:setI", "SR-PS-HC-101:setI", "SR-PS-HC-102:setI", "SR-PS-HC-103:setI", "SR-PS-HC-104:setI", "SR-PS-HC-105:setI", "SR-PS-HC-106:setI", "SR-PS-HC-107:setI", "SR-PS-HC-111:setI", "SR-PS-HC-112:setI", "SR-PS-HC-113:setI", "SR-PS-HC-114:setI", "SR-PS-HC-115:setI", "SR-PS-HC-116:setI", "SR-PS-HC-117:setI", "SR-PS-HC-121:setI", "SR-PS-HC-122:setI", "SR-PS-HC-123:setI", "SR-PS-HC-124:setI", "SR-PS-HC-125:setI", "SR-PS-HC-126:setI", "SR-PS-HC-127:setI", "SR-PS-HC-131:setI", "SR-PS-HC-132:setI", "SR-PS-HC-133:setI", "SR-PS-HC-134:setI", "SR-PS-HC-135:setI", "SR-PS-HC-136:setI", "SR-PS-HC-137:setI", "SR-PS-HC-141:setI", "SR-PS-HC-142:setI", "SR-PS-HC-143:setI", "SR-PS-HC-144:setI", "SR-PS-HC-145:setI", "SR-PS-HC-146:setI", "SR-PS-HC-147:setI", "SR-PS-HC-151:setI", "SR-PS-HC-152:setI", "SR-PS-HC-153:setI", "SR-PS-HC-154:setI", "SR-PS-HC-155:setI", "SR-PS-HC-156:setI", "SR-PS-HC-157:setI", "SR-PS-HC-161:setI", "SR-PS-HC-162:setI", "SR-PS-HC-163:setI", "SR-PS-HC-164:setI", "SR-PS-HC-165:setI", "SR-PS-HC-166:setI", "SR-PS-HC-167:setI", "SR-PS-HC-171:setI", "SR-PS-HC-172:setI", "SR-PS-HC-173:setI", "SR-PS-HC-174:setI", "SR-PS-HC-175:setI", "SR-PS-HC-176:setI", "SR-PS-HC-177:setI", "SR-PS-HC-181:setI", "SR-PS-HC-182:setI", "SR-PS-HC-183:setI", "SR-PS-HC-184:setI", "SR-PS-HC-185:setI", "SR-PS-HC-186:setI", "SR-PS-HC-187:setI", "SR-PS-HC-191:setI", "SR-PS-HC-192:setI", "SR-PS-HC-193:setI", "SR-PS-HC-194:setI", "SR-PS-HC-195:setI", "SR-PS-HC-196:setI", "SR-PS-HC-197:setI", "SR-PS-HC-201:setI", "SR-PS-HC-202:setI", "SR-PS-HC-203:setI", "SR-PS-HC-204:setI", "SR-PS-HC-205:setI", "SR-PS-HC-206:setI", "SR-PS-HC-207:setI", "SR-PS-HC-211:setI", "SR-PS-HC-212:setI", "SR-PS-HC-213:setI", "SR-PS-HC-214:setI", "SR-PS-HC-215:setI", "SR-PS-HC-216:setI", "SR-PS-HC-217:setI", "SR-PS-HC-221:setI", "SR-PS-HC-222:setI", "SR-PS-HC-223:setI", "SR-PS-HC-224:setI", "SR-PS-HC-225:setI", "SR-PS-HC-226:setI", "SR-PS-HC-227:setI", "SR-PS-HC-231:setI", "SR-PS-HC-232:setI", "SR-PS-HC-233:setI", "SR-PS-HC-234:setI", "SR-PS-HC-235:setI", "SR-PS-HC-236:setI", "SR-PS-HC-237:setI", "SR-PS-HC-241:setI", "SR-PS-HC-242:setI", "SR-PS-HC-243:setI", "SR-PS-HC-244:setI", "SR-PS-HC-245:setI", "SR-PS-HC-246:setI", "SR-PS-HC-247:setI", "SR-PS-VC-011:setI", "SR-PS-VC-012:setI", "SR-PS-VC-013:setI", "SR-PS-VC-014:setI", "SR-PS-VC-015:setI", "SR-PS-VC-016:setI", "SR-PS-VC-017:setI", "SR-PS-VC-021:setI", "SR-PS-VC-022:setI", "SR-PS-VC-023:setI", "SR-PS-VC-024:setI", "SR-PS-VC-025:setI", "SR-PS-VC-026:setI", "SR-PS-VC-027:setI", "SR-PS-VC-031:setI", "SR-PS-VC-032:setI", "SR-PS-VC-033:setI", "SR-PS-VC-034:setI", "SR-PS-VC-035:setI", "SR-PS-VC-036:setI", "SR-PS-VC-037:setI", "SR-PS-VC-041:setI", "SR-PS-VC-042:setI", "SR-PS-VC-043:setI", "SR-PS-VC-044:setI", "SR-PS-VC-045:setI", "SR-PS-VC-046:setI", "SR-PS-VC-047:setI", "SR-PS-VC-051:setI", "SR-PS-VC-052:setI", "SR-PS-VC-053:setI", "SR-PS-VC-054:setI", "SR-PS-VC-055:setI", "SR-PS-VC-056:setI", "SR-PS-VC-057:setI", "SR-PS-VC-061:setI", "SR-PS-VC-062:setI", "SR-PS-VC-063:setI", "SR-PS-VC-064:setI", "SR-PS-VC-065:setI", "SR-PS-VC-066:setI", "SR-PS-VC-067:setI", "SR-PS-VC-071:setI", "SR-PS-VC-072:setI", "SR-PS-VC-073:setI", "SR-PS-VC-074:setI", "SR-PS-VC-075:setI", "SR-PS-VC-076:setI", "SR-PS-VC-077:setI", "SR-PS-VC-081:setI", "SR-PS-VC-082:setI", "SR-PS-VC-083:setI", "SR-PS-VC-084:setI", "SR-PS-VC-085:setI", "SR-PS-VC-086:setI", "SR-PS-VC-087:setI", "SR-PS-VC-091:setI", "SR-PS-VC-092:setI", "SR-PS-VC-093:setI", "SR-PS-VC-094:setI", "SR-PS-VC-095:setI", "SR-PS-VC-096:setI", "SR-PS-VC-097:setI", "SR-PS-VC-101:setI", "SR-PS-VC-102:setI", "SR-PS-VC-103:setI", "SR-PS-VC-104:setI", "SR-PS-VC-105:setI", "SR-PS-VC-106:setI", "SR-PS-VC-107:setI", "SR-PS-VC-111:setI", "SR-PS-VC-112:setI", "SR-PS-VC-113:setI", "SR-PS-VC-114:setI", "SR-PS-VC-115:setI", "SR-PS-VC-116:setI", "SR-PS-VC-117:setI", "SR-PS-VC-121:setI", "SR-PS-VC-122:setI", "SR-PS-VC-123:setI", "SR-PS-VC-124:setI", "SR-PS-VC-125:setI", "SR-PS-VC-126:setI", "SR-PS-VC-127:setI", "SR-PS-VC-131:setI", "SR-PS-VC-132:setI", "SR-PS-VC-133:setI", "SR-PS-VC-134:setI", "SR-PS-VC-135:setI", "SR-PS-VC-136:setI", "SR-PS-VC-137:setI", "SR-PS-VC-141:setI", "SR-PS-VC-142:setI", "SR-PS-VC-143:setI", "SR-PS-VC-144:setI", "SR-PS-VC-145:setI", "SR-PS-VC-146:setI", "SR-PS-VC-147:setI", "SR-PS-VC-151:setI", "SR-PS-VC-152:setI", "SR-PS-VC-153:setI", "SR-PS-VC-154:setI", "SR-PS-VC-155:setI", "SR-PS-VC-156:setI", "SR-PS-VC-157:setI", "SR-PS-VC-161:setI", "SR-PS-VC-162:setI", "SR-PS-VC-163:setI", "SR-PS-VC-164:setI", "SR-PS-VC-165:setI", "SR-PS-VC-166:setI", "SR-PS-VC-167:setI", "SR-PS-VC-171:setI", "SR-PS-VC-172:setI", "SR-PS-VC-173:setI", "SR-PS-VC-174:setI", "SR-PS-VC-175:setI", "SR-PS-VC-176:setI", "SR-PS-VC-177:setI", "SR-PS-VC-181:setI", "SR-PS-VC-182:setI", "SR-PS-VC-183:setI", "SR-PS-VC-184:setI", "SR-PS-VC-185:setI", "SR-PS-VC-186:setI", "SR-PS-VC-187:setI", "SR-PS-VC-191:setI", "SR-PS-VC-192:setI", "SR-PS-VC-193:setI", "SR-PS-VC-194:setI", "SR-PS-VC-195:setI", "SR-PS-VC-196:setI", "SR-PS-VC-197:setI", "SR-PS-VC-201:setI", "SR-PS-VC-202:setI", "SR-PS-VC-203:setI", "SR-PS-VC-204:setI", "SR-PS-VC-205:setI", "SR-PS-VC-206:setI", "SR-PS-VC-207:setI", "SR-PS-VC-211:setI", "SR-PS-VC-212:setI", "SR-PS-VC-213:setI", "SR-PS-VC-214:setI", "SR-PS-VC-215:setI", "SR-PS-VC-216:setI", "SR-PS-VC-217:setI", "SR-PS-VC-221:setI", "SR-PS-VC-222:setI", "SR-PS-VC-223:setI", "SR-PS-VC-224:setI", "SR-PS-VC-225:setI", "SR-PS-VC-226:setI", "SR-PS-VC-227:setI", "SR-PS-VC-231:setI", "SR-PS-VC-232:setI", "SR-PS-VC-233:setI", "SR-PS-VC-234:setI", "SR-PS-VC-235:setI", "SR-PS-VC-236:setI", "SR-PS-VC-237:setI", "SR-PS-VC-241:setI", "SR-PS-VC-242:setI", "SR-PS-VC-243:setI", "SR-PS-VC-244:setI", "SR-PS-VC-245:setI", "SR-PS-VC-246:setI", "SR-PS-VC-247:setI", "SR-PS-QL1-0101:setI", "SR-PS-QL2-0102:setI", "SR-PS-QL3-0103:setI", "SR-PS-QS4-0104:setI", "SR-PS-QS5-0105:setI", "SR-PS-QS5-0106:setI", "SR-PS-QS4-0107:setI", "SR-PS-QS3-0108:setI", "SR-PS-QS2-0109:setI", "SR-PS-QS1-0110:setI", "SR-PS-QS1-0201:setI", "SR-PS-QS2-0202:setI", "SR-PS-QS3-0203:setI", "SR-PS-QS4-0204:setI", "SR-PS-QS5-0205:setI", "SR-PS-QS5-0206:setI", "SR-PS-QS4-0207:setI", "SR-PS-QS3-0208:setI", "SR-PS-QS2-0209:setI", "SR-PS-QS1-0210:setI", "SR-PS-QS1-0301:setI", "SR-PS-QS2-0302:setI", "SR-PS-QS3-0303:setI", "SR-PS-QS4-0304:setI", "SR-PS-QS5-0305:setI", "SR-PS-QS5-0306:setI", "SR-PS-QS4-0307:setI", "SR-PS-QS3-0308:setI", "SR-PS-QS2-0309:setI", "SR-PS-QS1-0310:setI", "SR-PS-QS1-0401:setI", "SR-PS-QS2-0402:setI", "SR-PS-QS3-0403:setI", "SR-PS-QS4-0404:setI", "SR-PS-QS5-0405:setI", "SR-PS-QS5-0406:setI", "SR-PS-QS4-0407:setI", "SR-PS-QL3-0408:setI", "SR-PS-QL2-0409:setI", "SR-PS-QL1-0410:setI", "SR-PS-QL1-0501:setI", "SR-PS-QL2-0502:setI", "SR-PS-QL3-0503:setI", "SR-PS-QS4-0504:setI", "SR-PS-QS5-0505:setI", "SR-PS-QS5-0506:setI", "SR-PS-QS4-0507:setI", "SR-PS-QS3-0508:setI", "SR-PS-QS2-0509:setI", "SR-PS-QS1-0510:setI", "SR-PS-QS1-0601:setI", "SR-PS-QS2-0602:setI", "SR-PS-QS3-0603:setI", "SR-PS-QS4-0604:setI", "SR-PS-QS5-0605:setI", "SR-PS-QS5-0606:setI", "SR-PS-QS4-0607:setI", "SR-PS-QS3-0608:setI", "SR-PS-QS2-0609:setI", "SR-PS-QS1-0610:setI", "SR-PS-QS1-0701:setI", "SR-PS-QS2-0702:setI", "SR-PS-QS3-0703:setI", "SR-PS-QS4-0704:setI", "SR-PS-QS5-0705:setI", "SR-PS-QS5-0706:setI", "SR-PS-QS4-0707:setI", "SR-PS-QS3-0708:setI", "SR-PS-QS2-0709:setI", "SR-PS-QS1-0710:setI", "SR-PS-QS1-0801:setI", "SR-PS-QS2-0802:setI", "SR-PS-QS3-0803:setI", "SR-PS-QS4-0804:setI", "SR-PS-QS5-0805:setI", "SR-PS-QS5-0806:setI", "SR-PS-QS4-0807:setI", "SR-PS-QL3-0808:setI", "SR-PS-QL2-0809:setI", "SR-PS-QL1-0810:setI", "SR-PS-QL1-0901:setI", "SR-PS-QL2-0902:setI", "SR-PS-QL3-0903:setI", "SR-PS-QS4-0904:setI", "SR-PS-QS5-0905:setI", "SR-PS-QS5-0906:setI", "SR-PS-QS4-0907:setI", "SR-PS-QS3-0908:setI", "SR-PS-QS2-0909:setI", "SR-PS-QS1-0910:setI", "SR-PS-QS1-1001:setI", "SR-PS-QS2-1002:setI", "SR-PS-QS3-1003:setI", "SR-PS-QS4-1004:setI", "SR-PS-QS5-1005:setI", "SR-PS-QS5-1006:setI", "SR-PS-QS4-1007:setI", "SR-PS-QS3-1008:setI", "SR-PS-QS2-1009:setI", "SR-PS-QS1-1010:setI", "SR-PS-QS1-1101:setI", "SR-PS-QS2-1102:setI", "SR-PS-QS3-1103:setI", "SR-PS-QS4-1104:setI", "SR-PS-QS5-1105:setI", "SR-PS-QS5-1106:setI", "SR-PS-QS4-1107:setI", "SR-PS-QS3-1108:setI", "SR-PS-QS2-1109:setI", "SR-PS-QS1-1110:setI", "SR-PS-QS1-1201:setI", "SR-PS-QS2-1202:setI", "SR-PS-QS3-1203:setI", "SR-PS-QS4-1204:setI", "SR-PS-QS5-1205:setI", "SR-PS-QS5-1206:setI", "SR-PS-QS4-1207:setI", "SR-PS-QL3-1208:setI", "SR-PS-QL2-1209:setI", "SR-PS-QL1-1210:setI", "SR-PS-QL1-1301:setI", "SR-PS-QL2-1302:setI", "SR-PS-QL3-1303:setI", "SR-PS-QS4-1304:setI", "SR-PS-QS5-1305:setI", "SR-PS-QS5-1306:setI", "SR-PS-QS4-1307:setI", "SR-PS-QS3-1308:setI", "SR-PS-QS2-1309:setI", "SR-PS-QS1-1310:setI", "SR-PS-QS1-1401:setI", "SR-PS-QS2-1402:setI", "SR-PS-QS3-1403:setI", "SR-PS-QS4-1404:setI", "SR-PS-QS5-1405:setI", "SR-PS-QS5-1406:setI", "SR-PS-QS4-1407:setI", "SR-PS-QS3-1408:setI", "SR-PS-QS2-1409:setI", "SR-PS-QS1-1410:setI", "SR-PS-QS1-1501:setI", "SR-PS-QS2-1502:setI", "SR-PS-QS3-1503:setI", "SR-PS-QS4-1504:setI", "SR-PS-QS5-1505:setI", "SR-PS-QS5-1506:setI", "SR-PS-QS4-1507:setI", "SR-PS-QS3-1508:setI", "SR-PS-QS2-1509:setI", "SR-PS-QS1-1510:setI", "SR-PS-QS1-1601:setI", "SR-PS-QS2-1602:setI", "SR-PS-QS3-1603:setI", "SR-PS-QS4-1604:setI", "SR-PS-QS5-1605:setI", "SR-PS-QS5-1606:setI", "SR-PS-QS4-1607:setI", "SR-PS-QL3-1608:setI", "SR-PS-QL2-1609:setI", "SR-PS-QL1-1610:setI", "SR-PS-QL1-1701:setI", "SR-PS-QL2-1702:setI", "SR-PS-QL3-1703:setI", "SR-PS-QS4-1704:setI", "SR-PS-QS5-1705:setI", "SR-PS-QS5-1706:setI", "SR-PS-QS4-1707:setI", "SR-PS-QS3-1708:setI", "SR-PS-QS2-1709:setI", "SR-PS-QS1-1710:setI", "SR-PS-QS1-1801:setI", "SR-PS-QS2-1802:setI", "SR-PS-QS3-1803:setI", "SR-PS-QS4-1804:setI", "SR-PS-QS5-1805:setI", "SR-PS-QS5-1806:setI", "SR-PS-QS4-1807:setI", "SR-PS-QS3-1808:setI", "SR-PS-QS2-1809:setI", "SR-PS-QS1-1810:setI", "SR-PS-QS1-1901:setI", "SR-PS-QS2-1902:setI", "SR-PS-QS3-1903:setI", "SR-PS-QS4-1904:setI", "SR-PS-QS5-1905:setI", "SR-PS-QS5-1906:setI", "SR-PS-QS4-1907:setI", "SR-PS-QS3-1908:setI", "SR-PS-QS2-1909:setI", "SR-PS-QS1-1910:setI", "SR-PS-QS1-2001:setI", "SR-PS-QS2-2002:setI", "SR-PS-QS3-2003:setI", "SR-PS-QS4-2004:setI", "SR-PS-QS5-2005:setI", "SR-PS-QS5-2006:setI", "SR-PS-QS4-2007:setI", "SR-PS-QL3-2008:setI", "SR-PS-QL2-2009:setI", "SR-PS-QL1-2010:setI", "SR-PS-QL1-2101:setI", "SR-PS-QL2-2102:setI", "SR-PS-QL3-2103:setI", "SR-PS-QS4-2104:setI", "SR-PS-QS5-2105:setI", "SR-PS-QS5-2106:setI", "SR-PS-QS4-2107:setI", "SR-PS-QS3-2108:setI", "SR-PS-QS2-2109:setI", "SR-PS-QS1-2110:setI", "SR-PS-QS1-2201:setI", "SR-PS-QS2-2202:setI", "SR-PS-QS3-2203:setI", "SR-PS-QS4-2204:setI", "SR-PS-QS5-2205:setI", "SR-PS-QS5-2206:setI", "SR-PS-QS4-2207:setI", "SR-PS-QS3-2208:setI", "SR-PS-QS2-2209:setI", "SR-PS-QS1-2210:setI", "SR-PS-QS1-2301:setI", "SR-PS-QS2-2302:setI", "SR-PS-QS3-2303:setI", "SR-PS-QS4-2304:setI", "SR-PS-QS5-2305:setI", "SR-PS-QS5-2306:setI", "SR-PS-QS4-2307:setI", "SR-PS-QS3-2308:setI", "SR-PS-QS2-2309:setI", "SR-PS-QS1-2310:setI", "SR-PS-QS1-2401:setI", "SR-PS-QS2-2402:setI", "SR-PS-QS3-2403:setI", "SR-PS-QS4-2404:setI", "SR-PS-QS5-2405:setI", "SR-PS-QS5-2406:setI", "SR-PS-QS4-2407:setI", "SR-PS-QL3-2408:setI", "SR-PS-QL2-2409:setI", "SR-PS-QL1-2410:setI", "SR-PS-S1-011:setI", "SR-PS-S2-012:setI", "SR-PS-SD-013:setI", "SR-PS-SF-014:setI", "SR-PS-SD-015:setI", "SR-PS-S4-016:setI", "SR-PS-S3-017:setI", "SR-PS-S5-021:setI", "SR-PS-S6-022:setI", "SR-PS-SD-023:setI", "SR-PS-SF-024:setI", "SR-PS-SD-025:setI", "SR-PS-S6-026:setI", "SR-PS-S5-027:setI", "SR-PS-S5-031:setI", "SR-PS-S6-032:setI", "SR-PS-SD-033:setI", "SR-PS-SF-034:setI", "SR-PS-SD-035:setI", "SR-PS-S6-036:setI", "SR-PS-S5-037:setI", "SR-PS-S3-041:setI", "SR-PS-S4-042:setI", "SR-PS-SD-043:setI", "SR-PS-SF-044:setI", "SR-PS-SD-045:setI", "SR-PS-S2-046:setI", "SR-PS-S1-047:setI", "SR-PS-S1-051:setI", "SR-PS-S2-052:setI", "SR-PS-SD-053:setI", "SR-PS-SF-054:setI", "SR-PS-SD-055:setI", "SR-PS-S4-056:setI", "SR-PS-S3-057:setI", "SR-PS-S5-061:setI", "SR-PS-S6-062:setI", "SR-PS-SD-063:setI", "SR-PS-SF-064:setI", "SR-PS-SD-065:setI", "SR-PS-S6-066:setI", "SR-PS-S5-067:setI", "SR-PS-S5-071:setI", "SR-PS-S6-072:setI", "SR-PS-SD-073:setI", "SR-PS-SF-074:setI", "SR-PS-SD-075:setI", "SR-PS-S6-076:setI", "SR-PS-S5-077:setI", "SR-PS-S3-081:setI", "SR-PS-S4-082:setI", "SR-PS-SD-083:setI", "SR-PS-SF-084:setI", "SR-PS-SD-085:setI", "SR-PS-S2-086:setI", "SR-PS-S1-087:setI", "SR-PS-S1-091:setI", "SR-PS-S2-092:setI", "SR-PS-SD-093:setI", "SR-PS-SF-094:setI", "SR-PS-SD-095:setI", "SR-PS-S4-096:setI", "SR-PS-S3-097:setI", "SR-PS-S5-101:setI", "SR-PS-S6-102:setI", "SR-PS-SD-103:setI", "SR-PS-SF-104:setI", "SR-PS-SD-105:setI", "SR-PS-S6-106:setI", "SR-PS-S5-107:setI", "SR-PS-S5-111:setI", "SR-PS-S6-112:setI", "SR-PS-SD-113:setI", "SR-PS-SF-114:setI", "SR-PS-SD-115:setI", "SR-PS-S6-116:setI", "SR-PS-S5-117:setI", "SR-PS-S3-121:setI", "SR-PS-S4-122:setI", "SR-PS-SD-123:setI", "SR-PS-SF-124:setI", "SR-PS-SD-125:setI", "SR-PS-S2-126:setI", "SR-PS-S1-127:setI", "SR-PS-S1-131:setI", "SR-PS-S2-132:setI", "SR-PS-SD-133:setI", "SR-PS-SF-134:setI", "SR-PS-SD-135:setI", "SR-PS-S4-136:setI", "SR-PS-S3-137:setI", "SR-PS-S5-141:setI", "SR-PS-S6-142:setI", "SR-PS-SD-143:setI", "SR-PS-SF-144:setI", "SR-PS-SD-145:setI", "SR-PS-S6-146:setI", "SR-PS-S5-147:setI", "SR-PS-S5-151:setI", "SR-PS-S6-152:setI", "SR-PS-SD-153:setI", "SR-PS-SF-154:setI", "SR-PS-SD-155:setI", "SR-PS-S6-156:setI", "SR-PS-S5-157:setI", "SR-PS-S3-161:setI", "SR-PS-S4-162:setI", "SR-PS-SD-163:setI", "SR-PS-SF-164:setI", "SR-PS-SD-165:setI", "SR-PS-S2-166:setI", "SR-PS-S1-167:setI", "SR-PS-S1-171:setI", "SR-PS-S2-172:setI", "SR-PS-SD-173:setI", "SR-PS-SF-174:setI", "SR-PS-SD-175:setI", "SR-PS-S4-176:setI", "SR-PS-S3-177:setI", "SR-PS-S5-181:setI", "SR-PS-S6-182:setI", "SR-PS-SD-183:setI", "SR-PS-SF-184:setI", "SR-PS-SD-185:setI", "SR-PS-S6-186:setI", "SR-PS-S5-187:setI", "SR-PS-S5-191:setI", "SR-PS-S6-192:setI", "SR-PS-SD-193:setI", "SR-PS-SF-194:setI", "SR-PS-SD-195:setI", "SR-PS-S6-196:setI", "SR-PS-S5-197:setI", "SR-PS-S3-201:setI", "SR-PS-S4-202:setI", "SR-PS-SD-203:setI", "SR-PS-SF-204:setI", "SR-PS-SD-205:setI", "SR-PS-S2-206:setI", "SR-PS-S1-207:setI", "SR-PS-S1-211:setI", "SR-PS-S2-212:setI", "SR-PS-SD-213:setI", "SR-PS-SF-214:setI", "SR-PS-SD-215:setI", "SR-PS-S4-216:setI", "SR-PS-S3-217:setI", "SR-PS-S5-221:setI", "SR-PS-S6-222:setI", "SR-PS-SD-223:setI", "SR-PS-SF-224:setI", "SR-PS-SD-225:setI", "SR-PS-S6-226:setI", "SR-PS-S5-227:setI", "SR-PS-S5-231:setI", "SR-PS-S6-232:setI", "SR-PS-SD-233:setI", "SR-PS-SF-234:setI", "SR-PS-SD-235:setI", "SR-PS-S6-236:setI", "SR-PS-S5-237:setI", "SR-PS-S3-241:setI", "SR-PS-S4-242:setI", "SR-PS-SD-243:setI", "SR-PS-SF-244:setI", "SR-PS-SD-245:setI", "SR-PS-S2-246:setI", "SR-PS-S1-247:setI", "SR-PS-SKEW-011:setI", "SR-PS-SKEW-012:setI", "SR-PS-SKEW-013:setI", "SR-PS-SKEW-014:setI", "SR-PS-SKEW-015:setI", "SR-PS-SKEW-016:setI", "SR-PS-SKEW-017:setI", "SR-PS-SKEW-021:setI", "SR-PS-SKEW-022:setI", "SR-PS-SKEW-023:setI", "SR-PS-SKEW-024:setI", "SR-PS-SKEW-025:setI", "SR-PS-SKEW-026:setI", "SR-PS-SKEW-027:setI", "SR-PS-SKEW-031:setI", "SR-PS-SKEW-032:setI", "SR-PS-SKEW-033:setI", "SR-PS-SKEW-034:setI", "SR-PS-SKEW-035:setI", "SR-PS-SKEW-036:setI", "SR-PS-SKEW-037:setI", "SR-PS-SKEW-041:setI", "SR-PS-SKEW-042:setI", "SR-PS-SKEW-043:setI", "SR-PS-SKEW-044:setI", "SR-PS-SKEW-045:setI", "SR-PS-SKEW-046:setI", "SR-PS-SKEW-047:setI", "SR-PS-SKEW-051:setI", "SR-PS-SKEW-052:setI", "SR-PS-SKEW-053:setI", "SR-PS-SKEW-054:setI", "SR-PS-SKEW-055:setI", "SR-PS-SKEW-056:setI", "SR-PS-SKEW-057:setI", "SR-PS-SKEW-061:setI", "SR-PS-SKEW-062:setI", "SR-PS-SKEW-063:setI", "SR-PS-SKEW-064:setI", "SR-PS-SKEW-065:setI", "SR-PS-SKEW-066:setI", "SR-PS-SKEW-067:setI", "SR-PS-SKEW-071:setI", "SR-PS-SKEW-072:setI", "SR-PS-SKEW-073:setI", "SR-PS-SKEW-074:setI", "SR-PS-SKEW-075:setI", "SR-PS-SKEW-076:setI", "SR-PS-SKEW-077:setI", "SR-PS-SKEW-081:setI", "SR-PS-SKEW-082:setI", "SR-PS-SKEW-083:setI", "SR-PS-SKEW-084:setI", "SR-PS-SKEW-085:setI", "SR-PS-SKEW-086:setI", "SR-PS-SKEW-087:setI", "SR-PS-SKEW-091:setI", "SR-PS-SKEW-092:setI", "SR-PS-SKEW-093:setI", "SR-PS-SKEW-094:setI", "SR-PS-SKEW-095:setI", "SR-PS-SKEW-096:setI", "SR-PS-SKEW-097:setI", "SR-PS-SKEW-101:setI", "SR-PS-SKEW-102:setI", "SR-PS-SKEW-103:setI", "SR-PS-SKEW-104:setI", "SR-PS-SKEW-105:setI", "SR-PS-SKEW-106:setI", "SR-PS-SKEW-107:setI", "SR-PS-SKEW-111:setI", "SR-PS-SKEW-112:setI", "SR-PS-SKEW-113:setI", "SR-PS-SKEW-114:setI", "SR-PS-SKEW-115:setI", "SR-PS-SKEW-116:setI", "SR-PS-SKEW-117:setI", "SR-PS-SKEW-121:setI", "SR-PS-SKEW-122:setI", "SR-PS-SKEW-123:setI", "SR-PS-SKEW-124:setI", "SR-PS-SKEW-125:setI", "SR-PS-SKEW-126:setI", "SR-PS-SKEW-127:setI", "SR-PS-SKEW-131:setI", "SR-PS-SKEW-132:setI", "SR-PS-SKEW-133:setI", "SR-PS-SKEW-134:setI", "SR-PS-SKEW-135:setI", "SR-PS-SKEW-136:setI", "SR-PS-SKEW-137:setI", "SR-PS-SKEW-141:setI", "SR-PS-SKEW-142:setI", "SR-PS-SKEW-143:setI", "SR-PS-SKEW-144:setI", "SR-PS-SKEW-145:setI", "SR-PS-SKEW-146:setI", "SR-PS-SKEW-147:setI", "SR-PS-SKEW-151:setI", "SR-PS-SKEW-152:setI", "SR-PS-SKEW-153:setI", "SR-PS-SKEW-154:setI", "SR-PS-SKEW-155:setI", "SR-PS-SKEW-156:setI", "SR-PS-SKEW-157:setI", "SR-PS-SKEW-161:setI", "SR-PS-SKEW-162:setI", "SR-PS-SKEW-163:setI", "SR-PS-SKEW-164:setI", "SR-PS-SKEW-165:setI", "SR-PS-SKEW-166:setI", "SR-PS-SKEW-167:setI", "SR-PS-SKEW-171:setI", "SR-PS-SKEW-172:setI", "SR-PS-SKEW-173:setI", "SR-PS-SKEW-174:setI", "SR-PS-SKEW-175:setI", "SR-PS-SKEW-176:setI", "SR-PS-SKEW-177:setI", "SR-PS-SKEW-181:setI", "SR-PS-SKEW-182:setI", "SR-PS-SKEW-183:setI", "SR-PS-SKEW-184:setI", "SR-PS-SKEW-185:setI", "SR-PS-SKEW-186:setI", "SR-PS-SKEW-187:setI", "SR-PS-SKEW-191:setI", "SR-PS-SKEW-192:setI", "SR-PS-SKEW-193:setI", "SR-PS-SKEW-194:setI", "SR-PS-SKEW-195:setI", "SR-PS-SKEW-196:setI", "SR-PS-SKEW-197:setI", "SR-PS-SKEW-201:setI", "SR-PS-SKEW-202:setI", "SR-PS-SKEW-203:setI", "SR-PS-SKEW-204:setI", "SR-PS-SKEW-205:setI", "SR-PS-SKEW-206:setI", "SR-PS-SKEW-207:setI", "SR-PS-SKEW-211:setI", "SR-PS-SKEW-212:setI", "SR-PS-SKEW-213:setI", "SR-PS-SKEW-214:setI", "SR-PS-SKEW-215:setI", "SR-PS-SKEW-216:setI", "SR-PS-SKEW-217:setI", "SR-PS-SKEW-221:setI", "SR-PS-SKEW-222:setI", "SR-PS-SKEW-223:setI", "SR-PS-SKEW-224:setI", "SR-PS-SKEW-225:setI", "SR-PS-SKEW-226:setI", "SR-PS-SKEW-227:setI", "SR-PS-SKEW-231:setI", "SR-PS-SKEW-232:setI", "SR-PS-SKEW-233:setI", "SR-PS-SKEW-234:setI", "SR-PS-SKEW-235:setI", "SR-PS-SKEW-236:setI", "SR-PS-SKEW-237:setI", "SR-PS-SKEW-241:setI", "SR-PS-SKEW-242:setI", "SR-PS-SKEW-243:setI", "SR-PS-SKEW-244:setI", "SR-PS-SKEW-245:setI", "SR-PS-SKEW-246:setI", "SR-PS-SKEW-247:setI", "SR-RF2-LLRF:setGapVoltage", "SR-RF2-LLRF:setStationPhase", "SR-RF3-LLRF:setGapVoltage", "SR-RF3-LLRF:setStationPhase", "SR-PS-DMB09-Q1:setI", "SR-PS-DMB09-Q2:setI", "SR-PS-DMB09-Q3:setI", "SR-PS-DMB25-Q1:setI", "SR-PS-DMB25-Q2:setI", "SR-PS-DMB25-Q3:setI", "SR-PS-DMB41-Q1:setI", "SR-PS-DMB41-Q2:setI", "SR-PS-DMB41-Q3:setI", "SR-PS-DMB09-HC1:setI", "SR-PS-DMB09-HC2:setI", "SR-PS-DMB09-VC1:setI", "SR-PS-DMB09-VC2:setI", "SR-PS-DMB25-HC1:setI", "SR-PS-DMB25-HC2:setI", "SR-PS-DMB25-VC1:setI", "SR-PS-DMB25-VC2:setI", "SR-PS-DMB41-HC1:setI", "SR-PS-DMB41-HC2:setI", "SR-PS-DMB41-VC1:setI", "SR-PS-DMB41-VC2:setI"]  # PV nanes(SR)
  w15 = string[] ["LTB-PS-HC-1:setI", "LTB-PS-HC-2:setI", "LTB-PS-HC-3:setI", "LTB-PS-HC-4:setI", "LTB-PS-HC-5:setI", "LTB-PS-VC-1:setI", "LTB-PS-VC-2:setI", "LTB-PS-VC-3:setI", "LTB-PS-VC-4:setI", "LTB-PS-VC-5:setI", "LTB-PS-VC-6:setI", "LTB-PS-VC-7:setI", "LTB-PS-Q1A:setI", "LTB-PS-Q1B:setI", "LTB-PS-Q1C:setI", "LTB-PS-Q2A:setI", "LTB-PS-Q2B:setI", "LTB-PS-Q2C:setI", "LTB-PS-Q3A:setI", "LTB-PS-Q3B:setI", "LTB-PS-Q4A:setI", "LTB-PS-Q4B:setI", "LTB-PS-QQ:setI", "LTB-PS-BEND-1:setI", "LTB-PS-VC-2a:setI", "LTB-PS-HC-3a:setI", "LTB-PS-HC-3b:setI", "LTB-PS-HC-4a:setI", "LTB-PS-HC-5a:setI", "LI-DI-SLIT-motor:axis2Position1", "LI-DI-SLIT-motor:axis1Position1"]  # PV nanes(LTB)
  w16 = string[] ["BTS-PS-HC-1:setI", "BTS-PS-HC-2:setI", "BTS-PS-HC-3:setI", "BTS-PS-HC-4:setI", "BTS-PS-HC-5:setI", "BTS-PS-VC-2:setI", "BTS-PS-VC-3:setI", "BTS-PS-VC-4:setI", "BTS-PS-VC-5:setI", "BTS-PS-VC-6:setI", "BTS-PS-Q1A:setI", "BTS-PS-Q1B:setI", "BTS-PS-Q1C:setI", "BTS-PS-Q2A:setI", "BTS-PS-Q2B:setI", "BTS-PS-Q2C:setI", "BTS-PS-Q3A:setI", "BTS-PS-BEND-1:setI", "BTS-PS-BEND-2:setI", "BR-PS-EXT-K1:setHV", "BR-PS-EXT-K2:setHV", "SR-PS-INJ-SE1:setHV", "SR-PS-INJ-SE2:setHV", "SR-PS-INJ-K1:setHV", "SR-PS-INJ-K2:setHV", "SR-PS-INJ-K3:setHV", "SR-PS-INJ-K4:setHV", "CPCIPM-TI-EVR:Pulse4DelaySet", "CPCIPM-TI-EVR:Pulse5DelaySet", "CPCIPM-TI-EVR:Pulse3DelaySet", "CPCIPM-TI-EVR:Pulse6DelaySet", "CPCIPM-TI-EVR:Pulse7DelaySet", "T560:setADelay", "T560:setBDelay", "T560:setCDelay", "T560:setDDelay", "CPCIPM-TI-EVR:Pulse4DelaySet", "CPCIPM-TI-EVR:Pulse5DelaySet", "BR-PS-EXT-SE1:setHV", "BR-PS-EXT-SE2:setHV", "CPCIPM-TI-EVR:Pulse3DelaySet", "CPCIPM-TI-EVR:Pulse11DelaySet"]  # PV nanes(BTS)
  w19 = FALSE ("Trip Evt B")
  (unwired) string[] ["FE-DI-XBPM-051:SA:SA_X_MONITOR", "FE-DI-XBPM-051:SA:SA_Y_MONITOR", "FE-DI-XBPM-091:SA:SA_X_MONITOR", "FE-DI-XBPM-091:SA:SA_Y_MONITOR", "FE-DI-XBPM-211:SA:SA_X_MONITOR", "FE-DI-XBPM-211:SA:SA_Y_MONITOR", "FE-DI-XBPM-231:SA:SA_X_MONITOR", "FE-DI-XBPM-231:SA:SA_Y_MONITOR", "FE-DI-XBPM-251:SA:SA_X_MONITOR", "FE-DI-XBPM-251:SA:SA_Y_MONITOR", "FE-DI-XBPM-411:SA:SA_X_MONITOR", "FE-DI-XBPM-411:SA:SA_Y_MONITOR", "FE-DI-XBPM-451:SA:SA_X_MONITOR", "FE-DI-XBPM-451:SA:SA_Y_MONITOR"]
  (unwired) string[] ["LI-VA-VAL-01:STA:POS", "LI-VA-VAL-02:STA:POS", "LI-VA-VAL-03:STA:POS", "LI-VA-VAL-04:STA:POS", "LI-VA-VAL-05:STA:POS"]
  (unwired) string[] ["SR-DI-SOFB-H:getStatus", "SR-DI-SOFB-V:getStatus", "IGPF:TPSX:FBCTRL", "IGPF:TPSY:FBCTRL", "SR-DI-FOFB-H:getStatus", "SR-DI-FOFB-V:getStatus"]
  # "V1.4.5 \n修改shift register 儲存筆數上限(之前沒有)，改成5000\n增加fill pattern的gap值\n檢查處加入ID 的mode"
  # "這3個變動太頻繁，不紀錄"
  # "PV nanes(ID gap_phase_Taper_)"
  # "PV nanes(Feedback_ILK)"
  # "V1.4.2 改成直接用最大最小值當作scale的最大最小值"
  # "1.4.1\n將BeamCurrent 圖形的Y軸上下限\n改成取最大值的1.01倍，再無條件進位取整數\n最小值的0.99倍，再無條件捨去取整數"
  # "FE-DI-XBPM-051:SA:SA_Y_MONITOR"
  # "FE-DI-XBPM-051:SA:SA_X_MONITOR"
  # "TPS-SR-052:bpm4:ilk:enabled"
  # "0 為OPEN"
  # "VALVE(EPICS)"
  n1 = local read "last ? Hrs"() -> (w29:dbl)
  n2 = Multiply(x=3600.0 ("y"), y=w29) -> (x*y=w53:dbl)
  n3 = Get Date/Time In Seconds() -> (seconds since 1Jan1904=w24:timestamp)
  n4 = Subtract(x=w24, y=w53) -> (x-y=w23:timestamp)
  n5 = call "TimeToString.vi"("Time Stamp Control"=w24) -> ("result string"=w55:string)
  n6 = call "TimeToString.vi"("Time Stamp Control"=w23) -> ("result string"=w54:string)
  n7 = call <vilib>:"Application Directory.vi"() -> ("Application Directory"=w56:path)
  n8 = Build Path(base path=w56, name or relative path="DSN\\172-18-0-32.dsn") -> (appended path=w58:path)
  n9 = call-poly <vilib>:"DB Tools Open Connection.vi"("connection information"=w58) -> ("error out"=w47:errorcluster, "connection reference"=w46:T2)  [unwired: 7 in]
  n10 = Concatenate Strings("SELECT  float_val , smpl_time\nFROM sample \nwhere  channel_id = 104 and smpl_time between '" ("result string"), w54, "' ::timestamp and '" ("result string"), w55, "' ::timestamp" ("result string")) -> (w31:string)
  n11 = call-poly <vilib>:"DB Tools Execute Query.vi"("error in (no error)"=w47, "SQL query"=w31, "connection reference"=w46) -> ("error out"=w44:errorcluster, "recordset reference"=w45:T3)  [unwired: 5 in]
  n12 = call-poly <vilib>:"DB Tools Fetch Recordset Data.vi"("error in (no error)"=w44, "recordset reference"=w45) -> ("error out"=w42:errorcluster, "recordset data"=w39:variant[][], "recordset reference out"=w43:T3)  [unwired: 3 in]
  n13 = call-poly <vilib>:"DB Tools Free Object.vi"("error in (no error)"=w42, "recordset reference"=w43) -> ("error out"=w40:errorcluster, "connection reference"=w41:T2)  [unwired: 8 in]
  n14 = Variant To Data(type=string[][] [], Variant=w39) -> (data=w37:string[][])  [unwired: 1 in, 1 out]
  n15 = call <vilib>:"DB Tools Close Connection.vi"("error in (no error)"=w40, "connection reference"=w41) -> ()  [unwired: 5 in, 1 out]
  n16 = Transpose 2D Array(2D array=w37) -> (transposed array=w35:string[][])
  n17 = Index Array(array=w35, index (row) #1=0 ("index (row)"), index (row) #2=1 ("index (row)")) -> (element #1=w49:string[], element #2=w51:string[])  [unwired: 2 in]
  n18 = Fract/Exp String To Number(string=w49) -> (number=w25:dbl[])  [unwired: 3 in, 1 out]
  n19 = Array Max & Min(array=w25) -> (max value=w21:dbl, min value=w20:dbl)  [unwired: 2 out]
  n20 = for {
    tunnel: w51 -> [w62] mode=indexing
    tunnel: [w61] -> w50 mode=indexing
    n21 = Scan From String "Scan From String"(format string="%<%Y/%m/%d %p %I:%M:%S>T", input string=w62, initial scan location=u32 0, default 1=timestamp(-73814400 s since 1904-01-01)) -> (output 1=w65:timestamp)  [unwired: 1 in, 3 out]
    n22 = To Double Precision Float(number=w65) -> (double precision float=w61:dbl)
  }
  n23 = To Double Precision Float(number=w24) -> (double precision float=w27:dbl)
  n24 = To Double Precision Float(number=w23) -> (double precision float=w26:dbl)
  n25 = control-ref of="BeamCurrent History"() -> (w28:refnum<vi>)
  n26 = property on="Property Node" class="XYGraph (strict)"(reference=w28, "XScale.Maximum"=w27, "XScale.Minimum"=w26, "YScale.Maximum"=w21, "YScale.Minimum"=w20) -> ()  [unwired: 1 in, 2 out]
  n27 = local write "Refresh B"(w19) -> ()
  n28 = local write "Trip Evt B"(w19) -> ()
  n29 = Bundle(w50, w25) -> (w30:cluster{dbl[], dbl[]})  [unwired: 1 in]
  n30 = property on="result" class="Str"("Visible"=FALSE) -> ()  [unwired: 2 in, 2 out]
  n31 = Build Array (concatenate)(w8, w9, w4) -> (w7:string[])
  n32 = Build Array (concatenate)(w2, w15, w1, w16, w17, w7, string[] ["SR-DI-FOFB-H:setStatus", "SR-DI-FOFB-V:setStatus", "IGPF:TPSX:FBCTRL", "IGPF:TPSY:FBCTRL", "TPS-SR-022:bpm3:ilk:enabled", "SR-DI-ANGLE-ILK:StatusX", "SR-DI-ANGLE-ILK:StatusY", "SR-DI-RF-FB:setStatus", "SR-ID-EPU48-TFF:status", "SR-ID-EPU48-CFF:status", "SR-ID-EPU46-TFF:status", "SR-ID-EPU46-CFF:status"], w3, w6, w5) -> (w18:string[])
  "PV list" <- w18
  n33 = Get Date/Time In Seconds() -> (seconds since 1Jan1904=w12:timestamp)
  n34 = To Double Precision Float(number=w12) -> (double precision float=w10:dbl)
  "Program Start Time" <- w10
  n35 = while {
    shift-right: [w228] -> _
    shift-left: _ -> [w226]
    shift-right: [w227] -> _
    shift-left: _ -> [w225]
    shift-right: [w94] -> _
    shift-left: w30 -> [w93]
    tunnel: w10 -> [w89]
    shift-right: [w68] -> _
    shift-left: _ -> [w69]
    stop <- "stop" stop-if-true
    (unwired) string[] ["Event Time      ", "PV_name        ", "Ori_Value", "New_Value "] ("diff_Value")
    w88 = dbl[] [1.0, 1.1666666666666667, 1.3333333333333333, 1.5, 1.6666666666666665, 1.8333333333333333, 2.0, 2.142857142857143, 2.2857142857142856, 2.4285714285714284, 2.571428571428571, 2.7142857142857144, 2.857142857142857, 3.0, 3.142857142857143, 3.2857142857142856, 3.4285714285714284, 3.571428571428571, 3.7142857142857144, 3.857142857142857, 4.0, 4.125, 4.25, 4.375, 4.5, 4.625, 4.75, 4.875, 5.0, 5.125, 5.25, 5.375, 5.5, 5.625, 5.75, 5.875, 6.0, 6.142857142857143, 6.285714285714286, 6.428571428571429, 6.571428571428571, 6.714285714285714, 6.857142857142857, 7.0, 7.142857142857143, 7.285714285714286, 7.428571428571429, 7.571428571428571, 7.714285714285714, 7.857142857142857, 8.0, 8.142857142857142, 8.285714285714286, 8.428571428571429, 8.571428571428571, 8.714285714285714, 8.857142857142858, 9.0, 9.142857142857142, 9.285714285714286, 9.428571428571429, 9.571428571428571, 9.714285714285714, 9.857142857142858, 10.0, 10.142857142857142, 10.285714285714286, 10.428571428571429, 10.571428571428571, 10.714285714285714, 10.857142857142858, 11.0, 11.142857142857142, 11.285714285714286, 11.428571428571429, 11.571428571428571, 11.714285714285714, 11.857142857142858, 12.0, 12.125, 12.25, 12.375, 12.5, 12.625, 12.75, 12.875, 13.0, 13.125, 13.25, 13.375, 13.5, 13.625, 13.75, 13.875, 14.0, 14.142857142857142, 14.285714285714286, 14.428571428571429, 14.571428571428571, 14.714285714285714, 14.857142857142858, 15.0, 15.142857142857142, 15.285714285714286, 15.428571428571429, 15.571428571428571, 15.714285714285714, 15.857142857142858, 16.0, 16.142857142857142, 16.285714285714285, 16.428571428571427, 16.571428571428573, 16.714285714285715, 16.857142857142858, 17.0, 17.142857142857142, 17.285714285714285, 17.428571428571427, 17.571428571428573, 17.714285714285715, 17.857142857142858, 18.0, 18.142857142857142, 18.285714285714285, 18.428571428571427, 18.571428571428573, 18.714285714285715, 18.857142857142858, 19.0, 19.142857142857142, 19.285714285714285, 19.428571428571427, 19.571428571428573, 19.714285714285715, 19.857142857142858, 20.0, 20.125, 20.25, 20.375, 20.5, 20.625, 20.75, 20.875, 21.0, 21.125, 21.25, 21.375, 21.5, 21.625, 21.75, 21.875, 22.0, 22.142857142857142, 22.285714285714285, 22.428571428571427, 22.571428571428573, 22.714285714285715, 22.857142857142858, 23.0, 23.142857142857142, 23.285714285714285, 23.428571428571427, 23.571428571428573, 23.714285714285715, 23.857142857142858, 24.0, 24.166666666666668, 24.333333333333332, 24.5, 24.666666666666668, 24.833333333333332]  # Array of X axis  平均分配至各段
    w119 = string[] ["SR-ID-IU22-05:setECMode", "SR-ID-IU22A-09:setECMode", "SR-ID-IU22B-09:setECMode", "SR-ID-IUT22-21:setECMode", "SR-ID-IU22-23:setECMode", "SR-ID-IU22A-25:setECMode", "SR-ID-IU22B-25:setECMode", "SR-ID-EPU48A-41:setECMode", "SR-ID-EPU48B-41:setECMode", "SR-ID-EPU46-45:setECMode"]  # ID_mode
    w205 = string[] ["FE-05-PAB:Open", "FE-05-MGV:Open", "FE-05-FCV:Open", "FE-09-PAB:Open", "FE-09-MGV:Open", "FE-09-FCV:Open", "FE-21-PAB:Open", "FE-21-MGV:Open", "FE-21-FCV:Open", "FE-23-PAB:Open", "FE-23-PAB:Open", "FE-23-FCV:Open", "FE-25-PAB:Open", "FE-25-MGV:Open", "FE-25-FCV:Open", "FE-41-PAB:Open", "FE-41-MGV:Open", "FE-41-FCV:Open", "FE-45-PAB:Open", "FE-45-MGV:Open", "FE-45-FCV:Open"]  # PAB_MGV_FCV enable
    (unwired) "LI-DI-WCM:getWfCh1"
    (unwired) "SR-DI-FP:CurrentBuffer"
    w343 = 0.001
    w341 = string[] ["SR-DI-BPM-011:Y", "SR-DI-BPM-012:Y", "SR-DI-BPM-013:Y", "SR-DI-BPM-014:Y", "SR-DI-BPM-015:Y", "SR-DI-BPM-016:Y", "SR-DI-BPM-017:Y", "SR-DI-BPM-021:Y", "SR-DI-BPM-022:Y", "SR-DI-BPM-023:Y", "SR-DI-BPM-024:Y", "SR-DI-BPM-025:Y", "SR-DI-BPM-026:Y", "SR-DI-BPM-027:Y", "SR-DI-BPM-031:Y", "SR-DI-BPM-032:Y", "SR-DI-BPM-033:Y", "SR-DI-BPM-034:Y", "SR-DI-BPM-035:Y", "SR-DI-BPM-036:Y", "SR-DI-BPM-037:Y", "SR-DI-BPM-041:Y", "SR-DI-BPM-042:Y", "SR-DI-BPM-043:Y", "SR-DI-BPM-044:Y", "SR-DI-BPM-045:Y", "SR-DI-BPM-046:Y", "SR-DI-BPM-047:Y", "SR-DI-BPM-048:Y", "SR-DI-BPM-050:Y", "SR-DI-BPM-051:Y", "SR-DI-BPM-052:Y", "SR-DI-BPM-053:Y", "SR-DI-BPM-054:Y", "SR-DI-BPM-055:Y", "SR-DI-BPM-056:Y", "SR-DI-BPM-057:Y", "SR-DI-BPM-061:Y", "SR-DI-BPM-062:Y", "SR-DI-BPM-063:Y", "SR-DI-BPM-064:Y", "SR-DI-BPM-065:Y", "SR-DI-BPM-066:Y", "SR-DI-BPM-067:Y", "SR-DI-BPM-071:Y", "SR-DI-BPM-072:Y", "SR-DI-BPM-073:Y", "SR-DI-BPM-074:Y", "SR-DI-BPM-075:Y", "SR-DI-BPM-076:Y", "SR-DI-BPM-077:Y", "SR-DI-BPM-081:Y", "SR-DI-BPM-082:Y", "SR-DI-BPM-083:Y", "SR-DI-BPM-084:Y", "SR-DI-BPM-085:Y", "SR-DI-BPM-086:Y", "SR-DI-BPM-087:Y", "SR-DI-BPM-091:Y", "SR-DI-BPM-092:Y", "SR-DI-BPM-093:Y", "SR-DI-BPM-094:Y", "SR-DI-BPM-095:Y", "SR-DI-BPM-096:Y", "SR-DI-BPM-097:Y", "SR-DI-BPM-101:Y", "SR-DI-BPM-102:Y", "SR-DI-BPM-103:Y", "SR-DI-BPM-104:Y", "SR-DI-BPM-105:Y", "SR-DI-BPM-106:Y", "SR-DI-BPM-107:Y", "SR-DI-BPM-111:Y", "SR-DI-BPM-112:Y", "SR-DI-BPM-113:Y", "SR-DI-BPM-114:Y", "SR-DI-BPM-115:Y", "SR-DI-BPM-116:Y", "SR-DI-BPM-117:Y", "SR-DI-BPM-121:Y", "SR-DI-BPM-122:Y", "SR-DI-BPM-123:Y", "SR-DI-BPM-124:Y", "SR-DI-BPM-125:Y", "SR-DI-BPM-126:Y", "SR-DI-BPM-127:Y", "SR-DI-BPM-128:Y", "SR-DI-BPM-130:Y", "SR-DI-BPM-131:Y", "SR-DI-BPM-132:Y", "SR-DI-BPM-133:Y", "SR-DI-BPM-134:Y", "SR-DI-BPM-135:Y", "SR-DI-BPM-136:Y", "SR-DI-BPM-137:Y", "SR-DI-BPM-141:Y", "SR-DI-BPM-142:Y", "SR-DI-BPM-143:Y", "SR-DI-BPM-144:Y", "SR-DI-BPM-145:Y", "SR-DI-BPM-146:Y", "SR-DI-BPM-147:Y", "SR-DI-BPM-151:Y", "SR-DI-BPM-152:Y", "SR-DI-BPM-153:Y", "SR-DI-BPM-154:Y", "SR-DI-BPM-155:Y", "SR-DI-BPM-156:Y", "SR-DI-BPM-157:Y", "SR-DI-BPM-161:Y", "SR-DI-BPM-162:Y", "SR-DI-BPM-163:Y", "SR-DI-BPM-164:Y", "SR-DI-BPM-165:Y", "SR-DI-BPM-166:Y", "SR-DI-BPM-167:Y", "SR-DI-BPM-171:Y", "SR-DI-BPM-172:Y", "SR-DI-BPM-173:Y", "SR-DI-BPM-174:Y", "SR-DI-BPM-175:Y", "SR-DI-BPM-176:Y", "SR-DI-BPM-177:Y", "SR-DI-BPM-181:Y", "SR-DI-BPM-182:Y", "SR-DI-BPM-183:Y", "SR-DI-BPM-184:Y", "SR-DI-BPM-185:Y", "SR-DI-BPM-186:Y", "SR-DI-BPM-187:Y", "SR-DI-BPM-191:Y", "SR-DI-BPM-192:Y", "SR-DI-BPM-193:Y", "SR-DI-BPM-194:Y", "SR-DI-BPM-195:Y", "SR-DI-BPM-196:Y", "SR-DI-BPM-197:Y", "SR-DI-BPM-201:Y", "SR-DI-BPM-202:Y", "SR-DI-BPM-203:Y", "SR-DI-BPM-204:Y", "SR-DI-BPM-205:Y", "SR-DI-BPM-206:Y", "SR-DI-BPM-207:Y", "SR-DI-BPM-208:Y", "SR-DI-BPM-210:Y", "SR-DI-BPM-211:Y", "SR-DI-BPM-212:Y", "SR-DI-BPM-213:Y", "SR-DI-BPM-214:Y", "SR-DI-BPM-215:Y", "SR-DI-BPM-216:Y", "SR-DI-BPM-217:Y", "SR-DI-BPM-221:Y", "SR-DI-BPM-222:Y", "SR-DI-BPM-223:Y", "SR-DI-BPM-224:Y", "SR-DI-BPM-225:Y", "SR-DI-BPM-226:Y", "SR-DI-BPM-227:Y", "SR-DI-BPM-231:Y", "SR-DI-BPM-232:Y", "SR-DI-BPM-233:Y", "SR-DI-BPM-234:Y", "SR-DI-BPM-235:Y", "SR-DI-BPM-236:Y", "SR-DI-BPM-237:Y", "SR-DI-BPM-241:Y", "SR-DI-BPM-242:Y", "SR-DI-BPM-243:Y", "SR-DI-BPM-244:Y", "SR-DI-BPM-245:Y", "SR-DI-BPM-246:Y", "SR-DI-BPM-247:Y"]  # sorted BPMY_174
    w340 = string[] ["SR-DI-BPM-011:X", "SR-DI-BPM-012:X", "SR-DI-BPM-013:X", "SR-DI-BPM-014:X", "SR-DI-BPM-015:X", "SR-DI-BPM-016:X", "SR-DI-BPM-017:X", "SR-DI-BPM-021:X", "SR-DI-BPM-022:X", "SR-DI-BPM-023:X", "SR-DI-BPM-024:X", "SR-DI-BPM-025:X", "SR-DI-BPM-026:X", "SR-DI-BPM-027:X", "SR-DI-BPM-031:X", "SR-DI-BPM-032:X", "SR-DI-BPM-033:X", "SR-DI-BPM-034:X", "SR-DI-BPM-035:X", "SR-DI-BPM-036:X", "SR-DI-BPM-037:X", "SR-DI-BPM-041:X", "SR-DI-BPM-042:X", "SR-DI-BPM-043:X", "SR-DI-BPM-044:X", "SR-DI-BPM-045:X", "SR-DI-BPM-046:X", "SR-DI-BPM-047:X", "SR-DI-BPM-048:X", "SR-DI-BPM-050:X", "SR-DI-BPM-051:X", "SR-DI-BPM-052:X", "SR-DI-BPM-053:X", "SR-DI-BPM-054:X", "SR-DI-BPM-055:X", "SR-DI-BPM-056:X", "SR-DI-BPM-057:X", "SR-DI-BPM-061:X", "SR-DI-BPM-062:X", "SR-DI-BPM-063:X", "SR-DI-BPM-064:X", "SR-DI-BPM-065:X", "SR-DI-BPM-066:X", "SR-DI-BPM-067:X", "SR-DI-BPM-071:X", "SR-DI-BPM-072:X", "SR-DI-BPM-073:X", "SR-DI-BPM-074:X", "SR-DI-BPM-075:X", "SR-DI-BPM-076:X", "SR-DI-BPM-077:X", "SR-DI-BPM-081:X", "SR-DI-BPM-082:X", "SR-DI-BPM-083:X", "SR-DI-BPM-084:X", "SR-DI-BPM-085:X", "SR-DI-BPM-086:X", "SR-DI-BPM-087:X", "SR-DI-BPM-091:X", "SR-DI-BPM-092:X", "SR-DI-BPM-093:X", "SR-DI-BPM-094:X", "SR-DI-BPM-095:X", "SR-DI-BPM-096:X", "SR-DI-BPM-097:X", "SR-DI-BPM-101:X", "SR-DI-BPM-102:X", "SR-DI-BPM-103:X", "SR-DI-BPM-104:X", "SR-DI-BPM-105:X", "SR-DI-BPM-106:X", "SR-DI-BPM-107:X", "SR-DI-BPM-111:X", "SR-DI-BPM-112:X", "SR-DI-BPM-113:X", "SR-DI-BPM-114:X", "SR-DI-BPM-115:X", "SR-DI-BPM-116:X", "SR-DI-BPM-117:X", "SR-DI-BPM-121:X", "SR-DI-BPM-122:X", "SR-DI-BPM-123:X", "SR-DI-BPM-124:X", "SR-DI-BPM-125:X", "SR-DI-BPM-126:X", "SR-DI-BPM-127:X", "SR-DI-BPM-128:X", "SR-DI-BPM-130:X", "SR-DI-BPM-131:X", "SR-DI-BPM-132:X", "SR-DI-BPM-133:X", "SR-DI-BPM-134:X", "SR-DI-BPM-135:X", "SR-DI-BPM-136:X", "SR-DI-BPM-137:X", "SR-DI-BPM-141:X", "SR-DI-BPM-142:X", "SR-DI-BPM-143:X", "SR-DI-BPM-144:X", "SR-DI-BPM-145:X", "SR-DI-BPM-146:X", "SR-DI-BPM-147:X", "SR-DI-BPM-151:X", "SR-DI-BPM-152:X", "SR-DI-BPM-153:X", "SR-DI-BPM-154:X", "SR-DI-BPM-155:X", "SR-DI-BPM-156:X", "SR-DI-BPM-157:X", "SR-DI-BPM-161:X", "SR-DI-BPM-162:X", "SR-DI-BPM-163:X", "SR-DI-BPM-164:X", "SR-DI-BPM-165:X", "SR-DI-BPM-166:X", "SR-DI-BPM-167:X", "SR-DI-BPM-171:X", "SR-DI-BPM-172:X", "SR-DI-BPM-173:X", "SR-DI-BPM-174:X", "SR-DI-BPM-175:X", "SR-DI-BPM-176:X", "SR-DI-BPM-177:X", "SR-DI-BPM-181:X", "SR-DI-BPM-182:X", "SR-DI-BPM-183:X", "SR-DI-BPM-184:X", "SR-DI-BPM-185:X", "SR-DI-BPM-186:X", "SR-DI-BPM-187:X", "SR-DI-BPM-191:X", "SR-DI-BPM-192:X", "SR-DI-BPM-193:X", "SR-DI-BPM-194:X", "SR-DI-BPM-195:X", "SR-DI-BPM-196:X", "SR-DI-BPM-197:X", "SR-DI-BPM-201:X", "SR-DI-BPM-202:X", "SR-DI-BPM-203:X", "SR-DI-BPM-204:X", "SR-DI-BPM-205:X", "SR-DI-BPM-206:X", "SR-DI-BPM-207:X", "SR-DI-BPM-208:X", "SR-DI-BPM-210:X", "SR-DI-BPM-211:X", "SR-DI-BPM-212:X", "SR-DI-BPM-213:X", "SR-DI-BPM-214:X", "SR-DI-BPM-215:X", "SR-DI-BPM-216:X", "SR-DI-BPM-217:X", "SR-DI-BPM-221:X", "SR-DI-BPM-222:X", "SR-DI-BPM-223:X", "SR-DI-BPM-224:X", "SR-DI-BPM-225:X", "SR-DI-BPM-226:X", "SR-DI-BPM-227:X", "SR-DI-BPM-231:X", "SR-DI-BPM-232:X", "SR-DI-BPM-233:X", "SR-DI-BPM-234:X", "SR-DI-BPM-235:X", "SR-DI-BPM-236:X", "SR-DI-BPM-237:X", "SR-DI-BPM-241:X", "SR-DI-BPM-242:X", "SR-DI-BPM-243:X", "SR-DI-BPM-244:X", "SR-DI-BPM-245:X", "SR-DI-BPM-246:X", "SR-DI-BPM-247:X"]  # sorted BPMX_174
    w399 = string[] ["BL-05A:HutchA_Enable", "BL-09A:HutchA_Enable", "BL-21A:HutchA_Enable", "BL-23A:HutchA_Enable", "BL-25A:HutchA_Enable", "BL-41A:HutchA_Enable", "BL-45A:HutchA_Enable"]  # Hutch enable
    w418 = string[] ["CPCI03-adl7452-0:doBank0Ch5", "CPCI05-adl7452-0:doBank0Ch5", "CPCI11-adl7452-0:doBank0Ch5", "CPCI12-adl7452-0:doBank0Ch5", "CPCI13-adl7452-0:doBank0Ch5", "CPCI21-adl7452-0:doBank0Ch5", "CPCI23-adl7452-0:doBank0Ch5"]  # FE enable
    w495 = 578.303 ("y")
    w500 = 1.202 ("y")
    # "SR-DI-RF-FB:getStatus"
    # "V1.4.2 改成直接用最大最小值當作scale的最大最小值"
    # "D:\\LOG運轉紀錄\\2016"
    # "45"
    # "41"
    # "25"
    # "23"
    # "21"
    # "09"
    # "05"
    # "05\n09\n21\n23\n25\n41\n45"
    # "gapMotorOff"
    n36 = event shown="[4] \"Switch Tab\": Value Change" {
      selector: _ -> [_ _ _ _ _ _ _ _ _ _ _]
      dyn-events: _ -> [_ _ _ _ _ _ _ _ _ _ _]
      timeout: 233 -> [_ _ _ _ _ _ _ _ _ _ _]
      tunnel: [_ w555 _ _ _ _ _ _ _ _ _] -> w95
      tunnel: [w541 w554 w561 w575 w612 w619 w646 w658 w684 w715 w733] -> w94
      tunnel: w93 -> [w541 w554 w561 _ w612 _ w646 w658 w684 w715 w733]
      tunnel: "last ? Hrs" -> [_ _ _ w582 _ w620 _ _ _ _ _]
      tunnel: w89 -> [_ w542 _ _ _ _ _ w657 _ w709 w717]
      tunnel: "T:Slow\nF:Fast" -> [_ _ _ w578 _ w615 _ _ _ _ _]
      tunnel: 0.004 ("最新時間") -> [_ _ _ w577 _ w614 _ _ _ _ _]
      event Timeout {
        n37 = event-data() -> ()  [unwired: 1 in, 3 out]
      }
      event "stop": Value Change {
        n38 = event-data() -> ("NewVal"=w555:bool)  [unwired: 1 in, 3 out]
        n39 = Get Date/Time In Seconds() -> (seconds since 1Jan1904=w548:timestamp)
        n40 = To Double Precision Float(number=w548) -> (double precision float=w547:dbl)
        n41 = Subtract(x=w547, y=43200.0) -> (x-y=w544:dbl)
        n42 = call "Main_Daily_path.vi"() -> ("Directory path"=w549:path)  [unwired: 10 in, 1 out]
        n43 = Greater?(x=w544, y=w542) -> (0:w545:bool)
        n44 = Select(t=w544, s=w545, f=w542) -> ()  [unwired: 1 out]
        n45 = call "B09_Save_new_lattice_files.vi"("For Test"=TRUE, "Directory Path"=w549) -> ()  [unwired: 10 in]
        n46 = call <vilib>:"Application Directory.vi"() -> ("Application Directory"=w543:path)
        n47 = local read "Diff list"() -> (w552:string[][])
        n48 = call "B07_Save_changed_PVs.vi"("For Test"=FALSE, "想要限制的筆數"=1000, "Directory Path"=w543, "紀錄起始時間  門檻"=w542, "diff_Value 2"=w552) -> ()  [unwired: 5 in, 2 out]
      }
      event "Open Button": Value Change {
        n49 = event-data() -> ()  [unwired: 1 in, 6 out]
        n50 = call <vilib>:"Beep.vi"("use system alert? (T)"=FALSE, "duration (msec)"=u32 40, "frequency (Hz)"=u32 1700) -> ()  [unwired: 9 in]
        n51 = call "Main_Daily_path.vi"() -> ("Directory path(STR)"=w560:string, "Directory path"=w559:path)  [unwired: 10 in]
        n52 = call <vilib>:"Check if File or Folder Exists.vi"("path"=w559) -> ("error out"=w565:errorcluster, "file or folder exists?"=w563:bool, "dup path"=w564:path)  [unwired: 8 in]
        n53 = case shown="False" w563 {
          tunnel: w564 -> [w572 w574]
          tunnel: w565 -> [w571 w573]
          tunnel: [w570 w574] -> _
          tunnel: [w569 w573] -> w562
          frame False {
            n54 = Create Folder(path (use dialog)=w572, error in=w571) -> (created path=w570:path, error out=w569:errorcluster)  [unwired: 1 in, 1 out]
          }
          frame True {
          }
        }
        n55 = Concatenate Strings("explorer ", w560) -> (w567:string)
        n56 = call <vilib>:"System Exec.vi"("wait until completion? (T)"=FALSE, "error in (no error)"=w562, "command line"=w567) -> ()  [unwired: 5 in, 4 out]
      }
      event "Trip Evt B": Value Change {
        n57 = event-data() -> ()  [unwired: 1 in, 1 out]
        n58 = flat-sequence {
          tunnel: w582 -> [w589]
          tunnel: [w589] -> w580
          tunnel: [w584] -> w579
          tunnel: w578 -> [w584]
          tunnel: w577 -> [w583]
          tunnel: [w583] -> w576
          tunnel: [w590] -> w581
          tunnel: w580 -> [w601]
          tunnel: w579 -> [w600]
          tunnel: w576 -> [w599]
          tunnel: [w607] -> w575
          tunnel: w581 -> [w607]
          frame #0 {
            n59 = property on="result" class="Str"("Visible"=FALSE) -> ()  [unwired: 2 in, 2 out]
            n60 = call <vilib>:"Beep.vi"("use system alert? (T)"=FALSE, "duration (msec)"=u32 40, "frequency (Hz)"=u32 1700) -> ()  [unwired: 9 in]
          }
          frame #1 {
            n61 = call "sub_plot_beamCurrent_and_trip_events.vi"("要看前幾個小時"=w601, "最新時間"=w599, "T:Slow\nF:Fast"=w600) -> ("Y min value"=w592:dbl, "Y max value"=w593:dbl, "X min value"=w594:dbl, "X max value"=w595:dbl, "BeamCurrent History"=w597:cluster{dbl[], dbl[]}[], "result"=→"result":string)  [unwired: 3 in]
            n62 = control-ref of="BeamCurrent History"() -> (w591:refnum<vi>)
            n63 = Index Array(array=w597, index=1) -> (element=w590:cluster{dbl[], dbl[]})
            n64 = property on="Property Node" class="XYGraph (strict)"(reference=w591, "XScale.Maximum"=w595, "XScale.Minimum"=w594, "YScale.Maximum"=w593, "YScale.Minimum"=w592) -> ()  [unwired: 1 in, 2 out]
          }
          frame #2 {
            n65 = local write "Trip Evt B"(FALSE ("Trip Evt B")) -> ()
            n66 = property on="result" class="Str"("Visible"=TRUE) -> ()  [unwired: 2 in, 2 out]
            n67 = call <vilib>:"Beep.vi"("use system alert? (T)"=FALSE, "duration (msec)"=u32 40, "frequency (Hz)"=u32 2000) -> ()  [unwired: 9 in]
          }
        }
      }
      event "Switch Tab": Value Change {
        n68 = event-data() -> ("NewVal"=w611:bool)  [unwired: 1 in, 1 out]
        n69 = Select(t=enum32{"_____", "           "}."_____" ("Tab Control"), s=w611, f=enum32{"_____", "           "}."           " ("Tab Control")) -> (s? t:f=→"Tab Control":enum32{"_____", "           "})
      }
      event "Refresh B": Value Change {
        n70 = event-data() -> ()  [unwired: 1 in, 6 out]
        n71 = flat-sequence {
          tunnel: w620 -> [w627]
          tunnel: [w627] -> w617
          tunnel: [w622] -> w616
          tunnel: w615 -> [w622]
          tunnel: w614 -> [w621]
          tunnel: [w621] -> w613
          tunnel: [w628] -> w618
          tunnel: w617 -> [w636]
          tunnel: w616 -> [w638]
          tunnel: w613 -> [w637]
          tunnel: [w645] -> w619
          tunnel: w618 -> [w645]
          frame #0 {
            n72 = property on="result" class="Str"("Visible"=FALSE) -> ()  [unwired: 2 in, 2 out]
            n73 = call <vilib>:"Beep.vi"("use system alert? (T)"=FALSE, "duration (msec)"=u32 40, "frequency (Hz)"=u32 1700) -> ()  [unwired: 9 in]
          }
          frame #1 {
            # "032  OPStatus    2195\n037  OPStatus    1899"
            n74 = call "sub_plot_beamCurrent_and_trip_events.vi"("要看前幾個小時"=w636, "最新時間"=w637, "T:Slow\nF:Fast"=w638) -> ("Y min value"=w632:dbl, "Y max value"=w633:dbl, "X min value"=w634:dbl, "X max value"=w635:dbl, "BeamCurrent History"=w630:cluster{dbl[], dbl[]}[], "result"=w631:string)  [unwired: 3 in]
            n75 = local write "result"(w631) -> ()
            n76 = control-ref of="BeamCurrent History"() -> (w639:refnum<vi>)
            n77 = property on="Property Node" class="XYGraph (strict)"(reference=w639, "XScale.Maximum"=w635, "XScale.Minimum"=w634, "YScale.Maximum"=w633, "YScale.Minimum"=w632) -> ()  [unwired: 1 in, 2 out]
            n78 = Index Array(array=w630, index=1) -> (element=w628:cluster{dbl[], dbl[]})
          }
          frame #2 {
            n79 = local write "Refresh B"(FALSE ("Trip Evt B")) -> ()
            n80 = property on="result" class="Str"("Visible"=TRUE) -> ()  [unwired: 2 in, 2 out]
            n81 = call <vilib>:"Beep.vi"("use system alert? (T)"=FALSE, "duration (msec)"=u32 40, "frequency (Hz)"=u32 2000) -> ()  [unwired: 9 in]
          }
        }
      }
      event "Save Lattice Button": Value Change {
        n82 = event-data() -> ()  [unwired: 1 in, 2 out]
        n83 = flat-sequence {
          frame #0 {
            n84 = call <vilib>:"Beep.vi"("use system alert? (T)"=FALSE, "duration (msec)"=u32 40, "frequency (Hz)"=u32 1700) -> ()  [unwired: 9 in]
          }
          frame #1 {
            n85 = call "Main_Daily_path.vi"() -> ("Directory path"=w650:path)  [unwired: 10 in, 1 out]
            n86 = call "B09_Save_new_lattice_files.vi"("For Test"=FALSE, "Directory Path"=w650) -> ()  [unwired: 10 in]
          }
          frame #2 {
            n87 = call <vilib>:"Beep.vi"("use system alert? (T)"=FALSE, "duration (msec)"=u32 40, "frequency (Hz)"=u32 2000) -> ()  [unwired: 9 in]
          }
        }
      }
      event "View Diff Button": Value Change {
        n88 = event-data() -> ()  [unwired: 1 in, 1 out]
        n89 = flat-sequence {
          tunnel: w657 -> [w663]
          tunnel: [w669] -> w655
          tunnel: [w674] -> w656
          tunnel: w655 -> [w674]
          tunnel: w656 -> [w676]
          frame #0 {
            # "12小時為43200sec"
            # "Save file"
            n90 = Get Date/Time In Seconds() -> (seconds since 1Jan1904=w668:timestamp)
            n91 = To Double Precision Float(number=w668) -> (double precision float=w667:dbl)
            n92 = call <vilib>:"Beep.vi"("use system alert? (T)"=FALSE, "duration (msec)"=u32 40, "frequency (Hz)"=u32 1700) -> ()  [unwired: 9 in]
            n93 = Subtract(x=w667, y=43200.0) -> (x-y=w664:dbl)
            n94 = Greater?(x=w664, y=w663) -> (0:w665:bool)
            n95 = Select(t=w664, s=w665, f=w663) -> (s? t:f=w662:dbl)
            n96 = local read "Diff list"() -> (w673:string[][])
            n97 = call "Main_Daily_path.vi"() -> ("Directory path"=w672:path)  [unwired: 10 in, 1 out]
            n98 = call "B07_Save_changed_PVs.vi"("For Test"=FALSE, "想要限制的筆數"=1000, "Directory Path"=w672, "紀錄起始時間  門檻"=w662, "diff_Value 2"=w673) -> ("saved file path"=w669:path)  [unwired: 5 in, 1 out]
          }
          frame #1 {
            # "Wait"
            n99 = Wait (ms)(milliseconds to wait=u32 300) -> ()  [unwired: 1 out]
          }
          frame #2 {
            # "Show"
            n100 = Path To String(path=w676) -> (string=w678:string)
            n101 = Concatenate Strings("explorer ", w678) -> (w677:string)
            n102 = call <vilib>:"System Exec.vi"("command line"=w677) -> ()  [unwired: 7 in, 4 out]
          }
          frame #3 {
            n103 = local write "View Diff Button"(FALSE ("View Diff Button")) -> ()
            n104 = call <vilib>:"Beep.vi"("use system alert? (T)"=FALSE, "duration (msec)"=u32 40, "frequency (Hz)"=u32 2000) -> ()  [unwired: 9 in]
          }
        }
      }
      event "Show Check list Button": Value Change {
        n105 = event-data() -> ()  [unwired: 1 in, 1 out]
        n106 = flat-sequence {
          frame #0 {
            n107 = call <vilib>:"Beep.vi"("use system alert? (T)"=FALSE, "duration (msec)"=u32 40, "frequency (Hz)"=u32 1700) -> ()  [unwired: 9 in]
          }
          frame #1 {
            n108 = local read "PV list"() -> (w688:string[])
            n109 = Array Size(array=w688) -> (size(s)=w689:i32)
            n110 = Array To Spreadsheet String(delimiter (Tab)="</BR>\n\r", array=w688, 3:"%s" ("format string")) -> (spreadsheet string=w700:string)
            n111 = Number To Decimal String(number=w689) -> (decimal integer string=w699:string)  [unwired: 1 in]
            n112 = call <vilib>:"Application Directory.vi"() -> ("Application Directory"=w690:path)
            n113 = Concatenate Strings("Tatal Checked PVs: ", w699, "</BR>\n\r" ("string"), w700) -> (w701:string)
            n114 = Build Path(base path=w690, name or relative path="Checked PV list.html") -> (appended path=w702:path)
            n115 = Write to Text File(file (use dialog)=w702, text=w701) -> ()  [unwired: 2 in, 3 out]
            n116 = flat-sequence {
              tunnel: w702 -> [w704]
              tunnel: [w704] -> w703
              frame #0 {
                n117 = Wait (ms)(milliseconds to wait=u32 500) -> ()  [unwired: 1 out]
              }
            }
            n118 = Path To String(path=w703) -> (string=w693:string)
            n119 = Concatenate Strings("explorer ", w693) -> (w692:string)
            n120 = call <vilib>:"System Exec.vi"("command line"=w692) -> ()  [unwired: 7 in, 4 out]
          }
          frame #2 {
            n121 = call <vilib>:"Beep.vi"("use system alert? (T)"=FALSE, "duration (msec)"=u32 40, "frequency (Hz)"=u32 2000) -> ()  [unwired: 9 in]
          }
        }
      }
      event Panel Close? {
        n122 = event-data() -> ()  [unwired: 1 in, 4 out]
        n123 = call "Main_Daily_path.vi"() -> ("Directory path"=w711:path)  [unwired: 10 in, 1 out]
        n124 = call "B09_Save_new_lattice_files.vi"("For Test"=TRUE, "Directory Path"=w711) -> ()  [unwired: 10 in]
        n125 = call <vilib>:"Application Directory.vi"() -> ("Application Directory"=w710:path)
        n126 = local read "Diff list"() -> (w714:string[][])
        n127 = call "B07_Save_changed_PVs.vi"("For Test"=FALSE, "想要限制的筆數"=1000, "Directory Path"=w710, "紀錄起始時間  門檻"=w709, "diff_Value 2"=w714) -> ()  [unwired: 5 in, 2 out]
        n128 = event-data() -> ()  [unwired: 2 in, 1 out]
      }
      event "Save Button": Value Change {
        n129 = event-data() -> ()  [unwired: 1 in, 1 out]
        n130 = Get Date/Time In Seconds() -> (seconds since 1Jan1904=w723:timestamp)
        n131 = To Double Precision Float(number=w723) -> (double precision float=w722:dbl)
        n132 = call <vilib>:"Beep.vi"("use system alert? (T)"=FALSE, "duration (msec)"=u32 40, "frequency (Hz)"=u32 1700) -> ()  [unwired: 9 in]
        n133 = Subtract(x=w722, y=43200.0) -> (x-y=w719:dbl)
        n134 = Greater?(x=w719, y=w717) -> (0:w720:bool)
        n135 = Select(t=w719, s=w720, f=w717) -> (s? t:f=w718:dbl)
        n136 = local read "Diff list"() -> (w727:string[][])
        n137 = call "Main_Daily_path.vi"() -> ("Directory path"=w726:path)  [unwired: 10 in, 1 out]
        n138 = call "B07_Save_changed_PVs.vi"("For Test"=FALSE, "想要限制的筆數"=1000, "Directory Path"=w726, "紀錄起始時間  門檻"=w718, "diff_Value 2"=w727) -> ()  [unwired: 5 in, 2 out]
        n139 = Get Date/Time In Seconds() -> (seconds since 1Jan1904=w736:timestamp)
        n140 = Format Date/Time String(time format string (%c)="%Y", seconds (now)=w736, UTC format=FALSE) -> (date/time string=w755:string)
        n141 = Format Date/Time String(time format string (%c)="%d", seconds (now)=w736, UTC format=FALSE) -> (date/time string=w764:string)
        n142 = call "to_be_2_string.vi"("string 2"=w764) -> ("substring 2"=w765:string)  [unwired: 10 in]
        n143 = Format Date/Time String(time format string (%c)="%m", seconds (now)=w736, UTC format=FALSE) -> (date/time string=w759:string)
        n144 = Format Date/Time String(time format string (%c)="%Y%m%d%H%M%S", seconds (now)=w736) -> (date/time string=w743:string)  [unwired: 1 in]
        n145 = Concatenate Strings("D" ("磁碟位置"), ":\\LOG運轉紀錄\\", w755, "\\", w759, "\\", w765) -> (w748:string)
        n146 = String To Path(string=w748) -> (path=w751:path)
        n147 = call <vilib>:"Check if File or Folder Exists.vi"("path"=w751) -> ("error out"=w749:errorcluster, "file or folder exists?"=w763:bool, "dup path"=w750:path)  [unwired: 8 in]
        n148 = invoke on="Cluster" class="Clust (strict)" method="Get Image"() -> ("image data"=w734:T4)  [unwired: 6 in, 5 out]
        n149 = case shown="False" w763 {
          tunnel: w750 -> [w769 w771]
          tunnel: w749 -> [w768 w770]
          tunnel: [w767 w771] -> w735
          tunnel: [w766 w770] -> _
          frame False {
            n150 = Create Folder(path (use dialog)=w769, error in=w768) -> (created path=w767:path, error out=w766:errorcluster)  [unwired: 1 in, 1 out]
          }
          frame True {
          }
        }
        n151 = Path To String(path=w735) -> (string=w747:string)
        n152 = Concatenate Strings(w747, "\\" ("string"), w743) -> (w737:string)
        n153 = Concatenate Strings(w737, ".jpg" ("file format")) -> (w738:string)
        n154 = String To Path(string=w738) -> (path=w742:path)
        n155 = call <vilib>:"Write JPEG File.vi"("quality (80)"=100, "image data"=w734, "path to JPEG file"=w742) -> ("error out"=→"error out 3":errorcluster)  [unwired: 7 in, 1 out]
        n156 = call "Main_Daily_path.vi"() -> ("Directory path"=w728:path)  [unwired: 10 in, 1 out]
        n157 = call "B09_Save_new_lattice_files.vi"("For Test"=FALSE, "Directory Path"=w728) -> ()  [unwired: 10 in]
      }
    }
    n158 = call-poly <userlib>:"CaLabGet.vi"("PV Names"=string[] ["FE-DI-XBPM-051:signals:sa.X", "FE-DI-XBPM-051:signals:sa.Y", "FE-DI-XBPM-091:SA:SA_X_MONITOR", "FE-DI-XBPM-091:SA:SA_Y_MONITOR", "FE-DI-XBPM-211:SA:SA_X_MONITOR", "FE-DI-XBPM-211:SA:SA_Y_MONITOR", "FE-DI-XBPM-231:SA:SA_X_MONITOR", "FE-DI-XBPM-231:SA:SA_Y_MONITOR", "FE-DI-XBPM-251:SA:SA_X_MONITOR", "FE-DI-XBPM-251:SA:SA_Y_MONITOR", "FE-DI-XBPM-411:SA:SA_X_MONITOR", "FE-DI-XBPM-411:SA:SA_Y_MONITOR", "FE-DI-XBPM-451:SA:SA_X_MONITOR", "FE-DI-XBPM-451:SA:SA_Y_MONITOR", "FE-DI-XBPM-052:signals:sa.X", "FE-DI-XBPM-052:signals:sa.Y", "FE-DI-XBPM-092:SA:SA_X_MONITOR", "FE-DI-XBPM-092:SA:SA_Y_MONITOR", "FE-DI-XBPM-212:SA:SA_X_MONITOR", "FE-DI-XBPM-212:SA:SA_Y_MONITOR", "FE-DI-XBPM-232:SA:SA_X_MONITOR", "FE-DI-XBPM-232:SA:SA_Y_MONITOR", "FE-DI-XBPM-252:SA:SA_X_MONITOR", "FE-DI-XBPM-252:SA:SA_Y_MONITOR", "FE-DI-XBPM-412:SA:SA_X_MONITOR", "FE-DI-XBPM-412:SA:SA_Y_MONITOR", "FE-DI-XBPM-452:SA:SA_X_MONITOR", "FE-DI-XBPM-452:SA:SA_Y_MONITOR"] ("appended array")) -> ("1rst Value (number)"=w366:dbl[])  [unwired: 8 in, 6 out]
    n159 = Multiply(x=w366, y=0.001) -> (x*y=w365:dbl[])
    n160 = disable-structure shown="Disabled" {
      frame Disabled {
        n161 = To Long Integer() -> (32bit integer=w816:i32)  [unwired: 1 in]
        n162 = case shown="1" w816 {
          tunnel: ["Decay" "Top-Up"] -> _
          frame 0, Default {
          }
          frame 1 {
          }
        }
      }
      frame Enabled {
      }
    }
    n163 = call-poly <userlib>:"CaLabGet.vi"("PV Names"=string[] ["SR-DI-FP:CurrentBuffer", "BR-DI-FP:CurrentBuffer"]) -> ("Value Array (number)"=w436:dbl[][])  [unwired: 8 in, 6 out]
    n164 = Index Array(array=w436, index (row) #1=0 ("index"), index (row) #2=1 ("index (row)")) -> (element #1=w81:dbl[], element #2=w70:dbl[])  [unwired: 2 in]
    n165 = Index Array(array=w365, index #1=0 ("index"), index #2=1 ("index"), index #3=2 ("index"), index #4=3 ("index"), index #5=4 ("index"), index #6=5 ("index"), index #7=6 ("index"), index #8=7 ("index"), index #9=8 ("index"), index #10=9 ("index"), index #11=10 ("index"), index #12=11 ("index"), index #13=12 ("index"), index #14=13 ("index"), index #15=14 ("index"), index #16=15 ("index"), index #17=16 ("index"), index #18=17 ("index"), index #19=18 ("index"), index #20=19 ("index"), index #21=20 ("index"), index #22=21 ("index"), index #23=22 ("index"), index #24=23 ("index"), index #25=24 ("index"), index #26=25 ("index"), index #27=26 ("index"), index #28=27 ("index")) -> (element #1=w283:dbl, element #2=w276:dbl, element #3=w282:dbl, element #4=w275:dbl, element #5=w281:dbl, element #6=w274:dbl, element #7=w280:dbl, element #8=w273:dbl, element #9=w279:dbl, element #10=w272:dbl, element #11=w278:dbl, element #12=w271:dbl, element #13=w277:dbl, element #14=w270:dbl, element #15=w175:dbl, element #16=w174:dbl, element #17=w173:dbl, element #18=w172:dbl, element #19=w163:dbl, element #20=w162:dbl, element #21=w157:dbl, element #22=w156:dbl, element #23=w155:dbl, element #24=w154:dbl, element #25=w123:dbl, element #26=w122:dbl, element #27=w121:dbl, element #28=w120:dbl)
    n166 = Build Array (concatenate)(w81, w81) -> (w79:dbl[])
    n167 = for {
      tunnel: w79 -> [w539] mode=indexing
      shift-right: [w533] -> _
      shift-left: _ -> [w532]
      shift-right: [w536] -> _
      shift-left: 0 -> [w537]
      tunnel: [w534] -> w83 mode=indexing if=w527
      w538 = 0.05  # Threshold
      n168 = Increment(x=w537) -> (x+1=w534:i32)
      n169 = Less Or Equal?(x=w539, y=w538) -> (x <= y?=w533:bool)
      n170 = Not Equal?(x=w533, y=w532) -> ()  [unwired: 1 out]
      n171 = Equal?(x=w533, y=TRUE) -> (x = y?=w524:bool)
      n172 = Equal?(x=w532, y=FALSE) -> (x = y?=w523:bool)
      n173 = Equal?(x=w533, y=FALSE) -> (x = y?=w529:bool)
      n174 = Equal?(x=w532, y=TRUE) -> (x = y?=w528:bool)
      n175 = And(x=w524, y=w523) -> (x .and. y?=w522:bool)
      n176 = And(x=w529, y=w528) -> (x .and. y?=w527:bool)
      n177 = Select(t=0, s=w522, f=w534) -> (s? t:f=w536:i32)
    }
    n178 = Array Max & Min(array=w83) -> (max value=w84:i32)  [unwired: 3 out]
    n179 = Multiply(x=w84, y=2) -> (x*y=w80:i32)
    n180 = Add Array Elements(numeric array=w70) -> (sum=w73:dbl)
    n181 = call-poly <userlib>:"CaLabGet.vi"("PV Names"=string[] ["LI-ES-CPS-01:PULSEMODE", "LI-ES-BPS-01:SETU:GRID", "LI-ES-BPS-01:SETU:MBM", "LI-ES-BPS-01:SETU:SBM", "LI-RF-HVP-31:SET:U", "CPCITM-TI-EVRTG:Pulse6DelaySet", "CPCITM-TI-EVRTG:Pulse7DelaySet", "CPCITM-TI-EVRTG:Pulse6WidthSet", "CPCITM-TI-EVRTG:Pulse7WidthSet", "CPCITM-TI-EVRTG:GTX6CtrlGTXPHSet", "CPCITM-TI-EVRTG:GTX7CtrlGTXPHSet", "CPCITM-TI-EVRTG:GTX6DlySet", "CPCITM-TI-EVRTG:GTX7DlySet"]) -> ("1rst Value (string)"=w428:string[], "1rst Value (number)"=w479:dbl[])  [unwired: 8 in, 5 out]
    n182 = call-poly <userlib>:"CaLabGet.vi"("PV Names"=string[] ["BR-PS-INJ-SE:setHV", "BR-PS-INJ-KI:setHV", "BR-PS-EXT-K1:setHV", "BR-PS-EXT-K2:setHV", "BR-PS-EXT-SE1:setHV", "BR-PS-EXT-SE2:setHV", "SR-PS-INJ-SE1:setHV", "SR-PS-INJ-SE2:setHV", "SR-PS-INJ-K1:setHV", "SR-PS-INJ-K2:setHV", "SR-PS-INJ-K3:setHV", "SR-PS-INJ-K4:setHV"]) -> ("1rst Value (number)"=w481:dbl[])  [unwired: 8 in, 6 out]
    n183 = call-poly <userlib>:"CaLabGet.vi"("PV Names"=string[] ["SR-RF-MSG:setFreq", "SR-RF2-LLRF:local", "SR-RF2-LLRF:getOperationMode", "SR-RF2-LLRF:getGapVoltage", "SR-RF2-LLRF:setGapVoltage", "SR-RF2-LLRF:setStationPhase", "SR-RF3-LLRF:local", "SR-RF3-LLRF:getOperationMode", "SR-RF3-LLRF:getGapVoltage", "SR-RF3-LLRF:setGapVoltage", "SR-RF3-LLRF:setStationPhase"]) -> ("1rst Value (number)"=w454:dbl[])  [unwired: 8 in, 6 out]
    n184 = Greater Or Equal?(x=w73, y=0.05) -> (x >= y?=w71:bool)
    n185 = call-poly <userlib>:"CaLabGet.vi"("PV Names"=string[] ["TI-INJ-PROC:TopupHiLowStart", "SR-DI-DCCT:BeamCurrent", "SR-DI-DCCT:BeamLifetime", "SR-DI-XPC-40:SigmaX", "SR-DI-XPC-40:SigmaY", "SR-DI-TUNE:nux", "SR-DI-TUNE:nuy", "IGPF:TPSX:SRAM:VEC:PEAKFREQ2", "IGPF:TPSY:SRAM:VEC:PEAKFREQ2", "TI-INJ-PROC:setBucketAddressStart", "TI-INJ-PROC:setBucketAddressLast", "TI-INJ-PROC:setBucketAddressStep"]) -> ("1rst Value (number)"=w515:dbl[])  [unwired: 8 in, 6 out]
    n186 = call-poly <userlib>:"CaLabGet.vi"("PV Names"=string[] ["LI:restoreFilename", "LTB:restoreFilename", "BR:restoreFilename", "BTS:restoreFilename", "SR:restoreFilename"]) -> ("1rst Value (string)"=w438:string[])  [unwired: 8 in, 6 out]
    n187 = Index Array(array=w428, index=0) -> (element=w426:string)
    n188 = Index Array(array=w479, index #1=0 ("index"), index #2=1 ("index"), index #3=2 ("index"), index #4=3 ("index"), index #5=4 ("index"), index #6=5 ("index"), index #7=6 ("index"), index #8=7 ("index"), index #9=8 ("index"), index #10=9 ("index"), index #11=10 ("index"), index #12=11 ("index"), index #13=12 ("index")) -> (element #2=w315:dbl, element #3=w430:dbl, element #4=w429:dbl, element #5=w313:dbl, element #8=w425:dbl, element #9=w424:dbl, element #10=w423:dbl, element #11=w422:dbl, element #12=w421:dbl, element #13=w420:dbl)  [unwired: 3 out]
    n189 = Index Array(array=w481, index #1=0 ("index"), index #2=1 ("index"), index #3=2 ("index"), index #4=3 ("index"), index #5=4 ("index"), index #6=5 ("index"), index #7=6 ("index"), index #8=7 ("index"), index #9=8 ("index"), index #10=9 ("index"), index #11=10 ("index"), index #12=11 ("index")) -> (element #1=w328:dbl, element #2=w327:dbl, element #3=w326:dbl, element #4=w325:dbl, element #5=w324:dbl, element #6=w323:dbl, element #7=w322:dbl, element #8=w321:dbl, element #9=w320:dbl, element #10=w319:dbl, element #11=w318:dbl, element #12=w317:dbl)
    n190 = Index Array(array=w454, index #1=0 ("index"), index #2=1 ("index"), index #3=2 ("index"), index #4=3 ("index"), index #5=4 ("index"), index #6=5 ("index"), index #7=6 ("index"), index #8=7 ("index"), index #9=8 ("index"), index #10=9 ("index"), index #11=10 ("index")) -> (element #1=w307:dbl, element #2=w451:dbl, element #3=w449:dbl, element #5=w231:dbl, element #6=w232:dbl, element #7=w446:dbl, element #8=w445:dbl, element #10=w303:dbl, element #11=w304:dbl)  [unwired: 2 out]
    n191 = Index Array(array=w515, index #1=0 ("index"), index #2=1 ("index"), index #3=2 ("index"), index #4=3 ("index"), index #5=4 ("index"), index #6=5 ("index"), index #7=6 ("index"), index #8=7 ("index"), index #9=8 ("index"), index #10=9 ("index"), index #11=10 ("index"), index #12=11 ("index")) -> (element #1=w513:dbl, element #2=w337:dbl, element #3=w336:dbl, element #4=w501:dbl, element #5=w499:dbl, element #6=w498:dbl, element #7=w497:dbl, element #8=w496:dbl, element #9=w494:dbl, element #10=w331:dbl, element #11=w330:dbl, element #12=w329:dbl)
    n192 = call-poly <userlib>:"CaLabGet.vi"("PV Names"=w205) -> ("1rst Value (number)"=w207:dbl[])  [unwired: 8 in, 6 out]
    n193 = Index Array(array=w438, index #1=0 ("index"), index #2=1 ("index"), index #3=2 ("index"), index #4=3 ("index"), index #5=4 ("index")) -> (element #1=w299:string, element #2=w298:string, element #3=w302:string, element #4=w301:string, element #5=w300:string)
    n194 = call-poly <userlib>:"CaLabGet.vi"("PV Names"=w399) -> ("1rst Value (string)"=w407:string[])  [unwired: 8 in, 6 out]
    n195 = To Byte Integer(number=w207) -> (8bit integer=w206:i8[])
    n196 = feedback #1() -> (w66:string)  [unwired: 1 in]
    n197 = case shown="True" w71 {
      tunnel: w70 -> [_ w521]
      tunnel: [w519 w521] -> w68
      tunnel: w69 -> [w519 _]
      tunnel: [w518 w520] -> w67
      tunnel: w66 -> [w518 _]
      frame False {
      }
      frame True {
        n198 = local read "NOW time"() -> (w520:string)
      }
    }
    n199 = feedback-in #1(w67) -> ()
    n200 = for {
      tunnel: w206 -> [w775] mode=indexing
      tunnel: [w772] -> w183 mode=indexing
      n201 = Number To Boolean Array(number=w775) -> (Boolean array=w774:bool[])
      n202 = Index Array(array=w774, index=0) -> (element=w772:bool)
    }
    n203 = for {
      tunnel: w407 -> [w785] mode=indexing
      tunnel: [w784] -> w408 mode=indexing
      n204 = case shown="\"Enable\"" w785 {
        tunnel: [FALSE TRUE] -> w784
        frame "Disable", Default {
        }
        frame "Enable" {
        }
      }
    }
    n205 = call-poly <userlib>:"CaLabGet.vi"("PV Names"=w418) -> ("1rst Value (string)"=w410:string[])  [unwired: 8 in, 6 out]
    n206 = call-poly <userlib>:"CaLabGet.vi"("PV Names"=string[] ["SR-ID-IU22-05:getGap", "SR-ID-IU22A-09:getGap", "SR-ID-IU22B-09:getGap", "SR-ID-IUT22-21:getGap", "SR-ID-IU22-23:getGap", "SR-ID-IU22A-25:getGap", "SR-ID-IU22B-25:getGap", "SR-ID-EPU48A-41:getGap", "SR-ID-EPU48A-41:getPhase", "SR-ID-EPU48B-41:getGap", "SR-ID-EPU48B-41:getPhase", "SR-ID-EPU46-45:getGap", "SR-ID-EPU46-45:getPhase", "SR-ID-IUT22-21:getGapTaper", "SR-ID-EPU48PS-41:getGap"]) -> ("1rst Value (number)"=w398:dbl[])  [unwired: 8 in, 6 out]
    n207 = for {
      tunnel: w410 -> [w789] mode=indexing
      tunnel: [w788] -> w409 mode=indexing
      n208 = case shown="\"enable\"" w789 {
        tunnel: [FALSE TRUE] -> w788
        frame "disable", Default {
        }
        frame "enable" {
        }
      }
    }
    n209 = call-poly <userlib>:"CaLabGet.vi"("PV Names"=string[] ["SR-ID-IU22-05:gapMotorOff", "SR-ID-IU22A-09:gapMotorOff", "SR-ID-IU22B-09:gapMotorOff", "SR-ID-IUT22-21:gapMotorOff", "SR-ID-IU22-23:gapMotorOff", "SR-ID-IU22A-25:gapMotorOff", "SR-ID-IU22B-25:gapMotorOff", "SR-ID-EPU48A-41:gapMotorOff", "SR-ID-EPU48B-41:gapMotorOff", "SR-ID-EPU46-45:gapMotorOff", "SR-ID-EPU48A-41:phaseMotorOff", "SR-ID-EPU48B-41:phaseMotorOff", "SR-ID-EPU46-45:phaseMotorOff"]) -> ("1rst Value (string)"=w350:string[])  [unwired: 8 in, 6 out]
    n210 = To Long Integer(number=w449) -> (32bit integer=w450:i32)
    n211 = To Long Integer(number=w451) -> (32bit integer=w452:i32)
    n212 = To Long Integer(number=w445) -> (32bit integer=w448:i32)
    n213 = To Long Integer(number=w446) -> (32bit integer=w447:i32)
    n214 = Index Array(array=w398, index #1=0 ("index"), index #2=1 ("index"), index #3=2 ("index"), index #4=3 ("index"), index #5=4 ("index"), index #6=5 ("index"), index #7=6 ("index"), index #8=7 ("index"), index #9=8 ("index"), index #10=9 ("index"), index #11=10 ("index"), index #12=11 ("index"), index #13=12 ("index"), index #14=13 ("index"), index #15=14 ("index")) -> (element #1=w297:dbl, element #2=w296:dbl, element #3=w295:dbl, element #4=w294:dbl, element #5=w293:dbl, element #6=w292:dbl, element #7=w291:dbl, element #8=w290:dbl, element #9=w289:dbl, element #10=w288:dbl, element #11=w287:dbl, element #12=w286:dbl, element #13=w285:dbl, element #14=w230:dbl, element #15=w284:dbl)
    n215 = for {
      tunnel: w350 -> [w781] mode=indexing
      tunnel: [w780] -> w349 mode=indexing
      n216 = case shown="\"1\", Default" w781 {
        tunnel: [FALSE TRUE] -> w780
        frame "1", Default {
        }
        frame "0" {
        }
      }
    }
    n217 = Index Array(array=w183, index #1=0 ("index"), index #2=1 ("index"), index #3=2 ("index"), index #4=3 ("index"), index #5=4 ("index"), index #6=5 ("index"), index #7=6 ("index"), index #8=7 ("index"), index #9=8 ("index"), index #10=9 ("index"), index #11=10 ("index"), index #12=11 ("index"), index #13=12 ("index"), index #14=13 ("index"), index #15=14 ("index"), index #16=15 ("index"), index #17=16 ("index"), index #18=17 ("index"), index #19=18 ("index"), index #20=19 ("index"), index #21=20 ("index")) -> (element #1=w180:bool, element #2=w179:bool, element #3=w178:bool, element #4=w167:bool, element #5=w166:bool, element #6=w165:bool, element #7=w160:bool, element #8=w159:bool, element #9=w158:bool, element #10=w149:bool, element #11=w148:bool, element #12=w147:bool, element #13=w142:bool, element #14=w141:bool, element #15=w140:bool, element #16=w139:bool, element #17=w138:bool, element #18=w137:bool, element #19=w136:bool, element #20=w135:bool, element #21=w134:bool)
    n218 = case shown="1" w452 {
      tunnel: [FALSE TRUE] -> w309
      frame 0, Default {
      }
      frame 1 {
      }
    }
    n219 = case shown="1" w447 {
      tunnel: [FALSE TRUE] -> w306
      frame 0, Default {
      }
      frame 1 {
      }
    }
    n220 = case shown="0" w450 {
      tunnel: [TRUE FALSE] -> w308
      frame 0 {
      }
      frame 1, Default {
      }
    }
    n221 = case shown="0" w448 {
      tunnel: [TRUE FALSE] -> w305
      frame 0 {
      }
      frame 1, Default {
      }
    }
    n222 = To Long Integer(number=w513) -> (32bit integer=w516:i32)
    n223 = Negate(x=w230) -> (-x=w229:dbl)
    n224 = case shown="1" w516 {
      tunnel: ["Decay" "Top-Up"] -> w338
      frame 0, Default {
      }
      frame 1 {
      }
    }
    n225 = Index Array(array=w408, index #1=0 ("index"), index #2=1 ("index"), index #3=2 ("index"), index #4=3 ("index"), index #5=4 ("index"), index #6=5 ("index"), index #7=6 ("index")) -> (element #1=w181:bool, element #2=w177:bool, element #3=w161:bool, element #4=w144:bool, element #5=w143:bool, element #6=w125:bool, element #7=w124:bool)
    n226 = case shown="\"MBM\", Default" w426 {
      tunnel: ["MBM" "SBM"] -> w316
      tunnel: w430 -> [w795 _]
      tunnel: [w795 w800] -> w314
      tunnel: w429 -> [_ w800]
      tunnel: w425 -> [_ w799]
      tunnel: w424 -> [w794 _]
      tunnel: [w794 w799] -> w312
      tunnel: w423 -> [_ w798]
      tunnel: w422 -> [w793 _]
      tunnel: [w793 w798] -> w311
      tunnel: w421 -> [_ w797]
      tunnel: w420 -> [w792 _]
      tunnel: [w792 w797] -> w310
      frame "MBM", Default {
      }
      frame "SBM" {
      }
    }
    n227 = Multiply(x=w501, y=w500) -> (x*y=w335:dbl)
    n228 = Divide(x=w496, y=w495) -> (x/y=w333:dbl)
    n229 = Multiply(x=w499, y=w500) -> (x*y=w334:dbl)
    n230 = Divide(x=w494, y=w495) -> (x/y=w332:dbl)
    n231 = Index Array(array=w409, index #1=0 ("index"), index #2=1 ("index"), index #3=2 ("index"), index #4=3 ("index"), index #5=4 ("index"), index #6=5 ("index"), index #7=6 ("index")) -> (element #1=w182:bool, element #2=w176:bool, element #3=w164:bool, element #4=w146:bool, element #5=w145:bool, element #6=w127:bool, element #7=w126:bool)
    n232 = call "FE_PAB_OpenState.vi"("FE"=w182, "XBPMX 2"=w175, "XBPMY 2"=w174, "Hutch"=w181, "PAB"=w180, "MGV"=w179, "FCV"=w178) -> ("XBPMX 2"=w171:string, "XBPMY 2"=w170:string)  [unwired: 7 in]
    n233 = call "FE_PAB_OpenState.vi"("FE"=w176, "XBPMX 2"=w173, "XBPMY 2"=w172, "Hutch"=w177, "PAB"=w167, "MGV"=w166, "FCV"=w165) -> ("XBPMX 2"=w169:string, "XBPMY 2"=w168:string)  [unwired: 7 in]
    n234 = call-poly <userlib>:"CaLabGet.vi"("PV Name"="TI-INJ-PROC:getTrig-SR-KICKER") -> ("1rst Value (string)"=w433:string)  [unwired: 8 in, 6 out]
    n235 = Index Array(array=w349, index #1=0 ("index"), index #2=1 ("index"), index #3=2 ("index"), index #4=3 ("index"), index #5=4 ("index"), index #6=5 ("index"), index #7=6 ("index"), index #8=7 ("index"), index #9=8 ("index"), index #10=9 ("index"), index #11=10 ("index"), index #12=11 ("index"), index #13=12 ("index")) -> (element #1=w269:bool, element #2=w268:bool, element #3=w267:bool, element #4=w266:bool, element #5=w265:bool, element #6=w264:bool, element #7=w263:bool, element #8=w262:bool, element #9=w261:bool, element #10=w260:bool, element #11=w259:bool, element #12=w258:bool, element #13=w257:bool)
    n236 = call-poly <userlib>:"CaLabGet.vi"("PV Names"=w340) -> ("1rst Value (number)"=w342:dbl[])  [unwired: 8 in, 6 out]
    n237 = call-poly <userlib>:"CaLabGet.vi"("PV Names"=w341) -> ("1rst Value (number)"=w344:dbl[])  [unwired: 8 in, 6 out]
    n238 = call "FE_PAB_OpenState.vi"("FE"=w164, "XBPMX 2"=w163, "XBPMY 2"=w162, "Hutch"=w161, "PAB"=w160, "MGV"=w159, "FCV"=w158) -> ("XBPMX 2"=w153:string, "XBPMY 2"=w152:string)  [unwired: 7 in]
    n239 = call-poly <userlib>:"CaLabGet.vi"("PV Names"=string[] ["SR-DI-FOFB-H:getStatus", "SR-DI-FOFB-V:getStatus", "IGPF:TPSX:FBCTRL", "IGPF:TPSY:FBCTRL", "TPS-SR-022:bpm3:ilk:enabled", "SR-DI-ANGLE-ILK:StatusX", "SR-DI-ANGLE-ILK:StatusY", "SR-DI-RF-FB:getStatus"]) -> ("1rst Value (string)"=w245:string[], "1rst Value (number)"=w246:dbl[])  [unwired: 8 in, 5 out]
    n240 = call "FE_PAB_OpenState.vi"("FE"=w146, "XBPMX 2"=w157, "XBPMY 2"=w156, "Hutch"=w144, "PAB"=w149, "MGV"=w148, "FCV"=w147) -> ("XBPMX 2"=w151:string, "XBPMY 2"=w150:string)  [unwired: 7 in]
    n241 = Multiply(x=w342, y=w343) -> (x*y=w223:dbl[])
    n242 = To Byte Integer(number=w246) -> (8bit integer=w242:i8[])
    n243 = Multiply(x=w344, y=w343) -> (x*y=w224:dbl[])
    n244 = for {
      tunnel: w242 -> [w777] mode=indexing
      tunnel: [w776] -> w252 mode=indexing
      n245 = case shown="1" w777 {
        tunnel: [TRUE FALSE] -> w776
        frame 1 {
        }
        frame 0, Default {
        }
      }
    }
    n246 = call "FE_PAB_OpenState.vi"("FE"=w145, "XBPMX 2"=w155, "XBPMY 2"=w154, "Hutch"=w143, "PAB"=w142, "MGV"=w141, "FCV"=w140) -> ("XBPMX 2"=w133:string, "XBPMY 2"=w132:string)  [unwired: 7 in]
    n247 = Index Array(array=w245, index #1=0 ("index"), index #2=1 ("index"), index #3=7 ("index")) -> (element #1=w240:string, element #2=w239:string, element #3=w90:string)
    n248 = call "FE_PAB_OpenState.vi"("FE"=w127, "XBPMX 2"=w123, "XBPMY 2"=w122, "Hutch"=w125, "PAB"=w139, "MGV"=w138, "FCV"=w137) -> ("XBPMX 2"=w131:string, "XBPMY 2"=w130:string)  [unwired: 7 in]
    n249 = call "FE_PAB_OpenState.vi"("FE"=w126, "XBPMX 2"=w121, "XBPMY 2"=w120, "Hutch"=w124, "PAB"=w136, "MGV"=w135, "FCV"=w134) -> ("XBPMX 2"=w129:string, "XBPMY 2"=w128:string)  [unwired: 7 in]
    n250 = Bundle("Array of X axis  平均分配至各段"=w88, w223) -> (w87:cluster{"Array of X axis  平均分配至各段":dbl[], dbl[]})  [unwired: 1 in]
    n251 = Bundle("Array of X axis  平均分配至各段"=w88, w224) -> (w86:cluster{"Array of X axis  平均分配至各段":dbl[], dbl[]})  [unwired: 1 in]
    n252 = Index Array(array=w252, index #1=2 ("index"), index #2=3 ("index"), index #3=4 ("index"), index #4=5 ("index"), index #5=6 ("index")) -> (element #1=w238:bool, element #2=w237:bool, element #3=w236:bool)  [unwired: 2 out]
    n253 = Equal?(x="1" ("1rst Value (string)"), y=w433) -> (x = y?=w431:bool)
    "x = y?" <- w431
    n254 = case shown="True" TRUE {
      tunnel: w95 -> [_ w540]
      frame False {
      }
      frame True {
        n255 = Quit LabVIEW(quit? (T)=w540) -> ()
      }
    }
    n256 = case shown="True" w431 {
      tunnel: w498 -> [_ w805]
      tunnel: w497 -> [_ w804]
      tunnel: [w803 w805] -> w228
      tunnel: [w802 w804] -> w227
      tunnel: w226 -> [w803 _]
      tunnel: w225 -> [w802 _]
      frame False {
      }
      frame True {
        n257 = local read "NOW date"() -> (→"date kickeron":string)
        n258 = local read "NOW time"() -> (→"time kickeron":string)
      }
    }
    n259 = Wait Until Next ms Multiple(millisecond multiple=u32 630) -> ()  [unwired: 1 out]
    n260 = local read "date kickeron"() -> (w234:string)
    n261 = local read "time kickeron"() -> (w233:string)
    n262 = Get Date/Time In Seconds() -> (seconds since 1Jan1904=w346:timestamp)
    n263 = call-poly <userlib>:"CaLabGet.vi"("PV Names"=w119) -> ("1rst Value (string)"=w108:string[])  [unwired: 8 in, 6 out]
    n264 = Format Date/Time String(time format string (%c)="%Y/%m/%d", seconds (now)=w346) -> (date/time string=→"NOW date":string)  [unwired: 1 in]
    n265 = Format Date/Time String(time format string (%c)="%Y/%m/%d", seconds (now)=w346) -> (date/time string=w256:string)  [unwired: 1 in]
    n266 = Format Date/Time String(time format string (%c)="%H:%M:%S", seconds (now)=w346) -> (date/time string=w255:string)  [unwired: 1 in]
    "NOW time" <- w255
    n267 = Index Array(array=w108, index #1=0 ("index"), index #2=1 ("index"), index #3=2 ("index"), index #4=3 ("index"), index #5=4 ("index"), index #6=5 ("index"), index #7=6 ("index"), index #8=7 ("index"), index #9=8 ("index"), index #10=9 ("index")) -> (element #1=w107:string, element #2=w106:string, element #3=w105:string, element #4=w104:string, element #5=w103:string, element #6=w102:string, element #7=w101:string, element #8=w100:string, element #9=w99:string, element #10=w98:string)
    n268 = Bundle By Name(cluster=T1 {"SR Fill Pattern"=array[864 elements], "Beam Current(mA"=320.769453, "Beam Lifetime(min)"=354.3939151043138, "Beamsize X(um)"=63.15189373514937, "Beamsize Y(um)"=38.03691397287648, "Tune X(from BPM)"=0.1487279843444227, "Tune Y(from BPM)"=0.2309197651663405, "Mode"="Top-Up", "NuX(from BBF) "=0.15142063757609414, "NuY(from BBF)"=0.22496346361412184, "IU22-23gap(R)"=7.0, "IU22-05gap(R)"=7.372, "IU22-05M"=TRUE, "IU22A-09gap(R)"=8.05, "IU22A-09M"=TRUE, "IU22B-09gap(R)"=40.001, "IU22B-09M"=FALSE, "IUT22-21gap(R)"=7.0, "IUT22-21M"=TRUE, "IU22-23M"=TRUE, "IU22A-25gap(R)"=7.0, "IU22A-25M"=TRUE, "IU22B-25gap(R)"=40.0, "IU22B-25M"=FALSE, "EPU48A-41gap(R)"=65.00055, "EPU48A-41gM"=FALSE, "EPU48B-41gap(R)"=27.450000000000003, "EPU48B-41gM"=TRUE, "EPU46-45gap(R)"=44.99850000000001, "EPU46-45gM"=FALSE, "EPU48A-41phase(R)"=0.00055, "EPU48B-41phase(R)"=0.0, "EPU46-45phase(R)"=5e-05, "Grid volt.(V)[S]"=33.0, "Gun mode"="MBM", "Mod.3 HV(kV)[S]"=35.37999999999996, "SR"="SR_DMB_2017_1024_0300LOCO.data", "BR"="Booster_2017_1023_0900.data", "LI"="Linac_2017_0413_1015.data", "LTB"="LTB_JT_2017_0828_1050.data", "BTS"="BTS_2017_1023_0900.data", "RF2 remote"=TRUE, "RF2 OP mode"=TRUE, "RF2 phase.[S]"=-42.0, "RF Freq.(s)"=499655365.67399085, "RF2 gap volt[S]"=1600.0, "RF3 remote"=TRUE, "RF3 OP mode"=TRUE, "RF3 phase.[S]"=1.1999999999999995, "RF3 gap volt.[S]"=1600.0, "BBF V"=TRUE, "BBF H"=TRUE, "BR ext. kicker1(kV)"=17.666, "BR ext. kicker2(kV)"=17.666, "BR ext. sep.1(V)"=322.14, "BR ext. sep.2(V)"=441.1, "BR inj. sep.(V)"=104.95, "BR inj. kicker(kV)"=13.449999999999969, "SR kicker4(kV)"=7.945, "SR kicker3(kV)"=8.02, "SR kicker2(kV)"=8.142, "SR kicker1(kV)"=8.1, "SR inj. sep.2(V)"=397.2, "SR inj. sep.1(V)"=398.04, "Bucket Start"=100.0, "Bucket Last"=450.0, "Bucket Step"=10.0, "Orbit ILK(P)"=TRUE, "IU22-05 Hutch Enable"=TRUE, "IU22A-09M Hutch Enable"=TRUE, "IUT22-21M Hutch Enable"=TRUE, "IU22-23M Hutch Enable"=TRUE, "IU22A-25M Hutch Enable"=TRUE, "EPU48A-41M Hutch Enable"=TRUE, "EPU46-45M Hutch Enable"=FALSE, "EPU46-45 FE Enable"=TRUE, "EPU48A-41 FE Enable"=TRUE, "IU22A-25 FE Enable"=TRUE, "IU22-23 FE Enable"=TRUE, "IUT22-21 FE Enable"=TRUE, "IU22A-09 FE Enable"=TRUE, "IU22-05 FE Enable"=TRUE, "EPU48A-41pM"=FALSE, "EPU48B-41pM"=TRUE, "EPU46-45pM"=FALSE, "Gun volt.(V)[S]"=23.5, "Width count"=75.0, "2ns step"=2.0, "10ps delay"=150.0, "phase shifter"=130.0015, "Taper"=1.0899999999999999, "05XBPMX 1"=14.279, "09XBPMX 1"=-34.837, "21XBPMX 1"=-36.466, "23XBPMX 1"=-38.547000000000004, "25XBPMX 1"=-40.08, "41XBPMX 1"=-513.551, "45XBPMX 1"=-12.86, "05XBPMY 1"=51.999, "09XBPMY 1"=30.004, "21XBPMY 1"=-4.771, "23XBPMY 1"=19.080000000000002, "25XBPMY 1"=-4.366, "41XBPMY 1"=309.241, "45XBPMY 1"=1.842, "FOFB H"="On", "FOFB V"="On", "time string"="15:45:09", "date"="2017/10/28", "date (last kicker ON)"="2017/10/28", "time string (last kicker ON)"="15:43:52", "Radio Buttons 2"=enum."absolute", "09XBPMX 2"="23.77", "09XBPMY 2"="-18.01", "05XBPMY 2"="-459.85", "05XBPMX 2"="-403.56", "21XBPMY 2"="-134.87", "21XBPMX 2"="-31.92", "23XBPMY 2"="233.82", "23XBPMX 2"="11.09", "25XBPMY 2"="5171.53", "25XBPMX 2"="2152.43", "41XBPMY 2"=" closed", "41XBPMX 2"=" PAB ", "45XBPMX 2"=" Hutch ", "45XBPMY 2"=" closed", "05 mode"="Follow", "09A mode"="Follow", "09B mode"="Follow", "21 mode"="Follow", "23 mode"="Follow", "25A mode"="Follow", "25B mode"="Follow", "41A mode"="Follow", "41B mode"="Follow", "46 mode"="Follow", "BeamCurrent History"={"BPM NO.  1_172"=array[4319 elements], array[4319 elements]}, "SR Beam Current in            hours"=12.0, "RF FB"="On", "BPMX Graph 2"={"Array of X axis  平均分配至各段"=[1.0, 1.1666666666666667, 1.3333333333333333, 1.5, 1.6666666666666665, 1.8333333333333333, 2.0, 2.142857142857143, 2.2857142857142856, 2.4285714285714284, 2.571428571428571, 2.7142857142857144, 2.857142857142857, 3.0, 3.142857142857143, 3.2857142857142856, 3.4285714285714284, 3.571428571428571, 3.7142857142857144, 3.857142857142857, 4.0, 4.125, 4.25, 4.375, 4.5, 4.625, 4.75, 4.875, 5.0, 5.125, 5.25, 5.375, 5.5, 5.625, 5.75, 5.875, 6.0, 6.142857142857143, 6.285714285714286, 6.428571428571429, 6.571428571428571, 6.714285714285714, 6.857142857142857, 7.0, 7.142857142857143, 7.285714285714286, 7.428571428571429, 7.571428571428571, 7.714285714285714, 7.857142857142857, 8.0, 8.142857142857142, 8.285714285714286, 8.428571428571429, 8.571428571428571, 8.714285714285714, 8.857142857142858, 9.0, 9.142857142857142, 9.285714285714286, 9.428571428571429, 9.571428571428571, 9.714285714285714, 9.857142857142858, 10.0, 10.142857142857142, 10.285714285714286, 10.428571428571429, 10.571428571428571, 10.714285714285714, 10.857142857142858, 11.0, 11.142857142857142, 11.285714285714286, 11.428571428571429, 11.571428571428571, 11.714285714285714, 11.857142857142858, 12.0, 12.125, 12.25, 12.375, 12.5, 12.625, 12.75, 12.875, 13.0, 13.125, 13.25, 13.375, 13.5, 13.625, 13.75, 13.875, 14.0, 14.142857142857142, 14.285714285714286, 14.428571428571429, 14.571428571428571, 14.714285714285714, 14.857142857142858, 15.0, 15.142857142857142, 15.285714285714286, 15.428571428571429, 15.571428571428571, 15.714285714285714, 15.857142857142858, 16.0, 16.142857142857142, 16.285714285714285, 16.428571428571427, 16.571428571428573, 16.714285714285715, 16.857142857142858, 17.0, 17.142857142857142, 17.285714285714285, 17.428571428571427, 17.571428571428573, 17.714285714285715, 17.857142857142858, 18.0, 18.142857142857142, 18.285714285714285, 18.428571428571427, 18.571428571428573, 18.714285714285715, 18.857142857142858, 19.0, 19.142857142857142, 19.285714285714285, 19.428571428571427, 19.571428571428573, 19.714285714285715, 19.857142857142858, 20.0, 20.125, 20.25, 20.375, 20.5, 20.625, 20.75, 20.875, 21.0, 21.125, 21.25, 21.375, 21.5, 21.625, 21.75, 21.875, 22.0, 22.142857142857142, 22.285714285714285, 22.428571428571427, 22.571428571428573, 22.714285714285715, 22.857142857142858, 23.0, 23.142857142857142, 23.285714285714285, 23.428571428571427, 23.571428571428573, 23.714285714285715, 23.857142857142858, 24.0, 24.166666666666668, 24.333333333333332, 24.5, 24.666666666666668, 24.833333333333332], [-104.35000000000001, -27.61, -81.269, 31.074, 6.062, -136.0, 99.494, -88.141, -46.889, -165.06900000000002, 6.021, -84.98, 1.75, -8.811, 8.532, -133.949, -96.848, 24.799, 5.059, -100.301, 144.643, -9.353, 21.271, -55.053000000000004, 53.308, 191.175, 158.868, 222.566, -123.501, -26.869, 534.8770000000001, 573.141, -225.076, -6.779, 120.711, -75.419, 85.256, 50.948, -59.4, -203.09900000000002, -20.847, 130.465, -112.508, 76.115, 15.039, -35.207, -105.659, -16.897000000000002, 68.91, -141.159, 107.378, 144.351, -55.053000000000004, -193.076, 129.21, 58.157000000000004, -162.566, 153.643, 28.149, 9.358, -84.211, 85.112, 22.422, -31.252, 89.379, -47.49, 54.793, -68.275, 110.611, -118.584, -371.90500000000003, -20.115000000000002, -329.103, -249.097, -146.817, 118.556, -25.749, -98.32600000000001, 55.269, -122.093, 50.967, -55.89, 88.019, -0.462, -608.1560000000001, -139.752, -304.999, -215.022, 93.23400000000001, 44.699, -65.235, 37.049, -3.491, -169.852, 216.458, 50.398, -92.285, -132.13400000000001, -12.869, 66.74, -188.53300000000002, 148.653, -5.112, -71.334, -177.681, 41.168, -12.532, -184.913, 194.919, 52.414, -75.628, -80.415, -36.814, 105.73100000000001, -104.36800000000001, 110.101, 49.669000000000004, -67.327, -157.372, 29.624000000000002, 22.156, -105.663, 47.799, 11.591000000000001, -75.285, -79.821, 34.331, -24.937, -158.703, 177.15, 200.872, -165.849, -60.67, 20.183, -15.311, -111.206, 107.58800000000001, 26.489, 69.547, -41.230000000000004, 81.986, 54.43, 253.076, 378.43600000000004, -117.003, -304.999, 131.013, 2.21, -158.435, 94.489, 63.017, -82.94500000000001, 99.147, 65.752, -37.261, -102.577, 41.791000000000004, 66.599, -163.73, 160.137, -7.15, -51.275, -140.353, 33.772, 54.203, -147.597, 128.696, 58.22, -47.144, -184.493, 56.980000000000004, 67.437, -54.227000000000004, -0.031]}, "BPMY Graph 2"={"Array of X axis  平均分配至各段"=[1.0, 1.1666666666666667, 1.3333333333333333, 1.5, 1.6666666666666665, 1.8333333333333333, 2.0, 2.142857142857143, 2.2857142857142856, 2.4285714285714284, 2.571428571428571, 2.7142857142857144, 2.857142857142857, 3.0, 3.142857142857143, 3.2857142857142856, 3.4285714285714284, 3.571428571428571, 3.7142857142857144, 3.857142857142857, 4.0, 4.125, 4.25, 4.375, 4.5, 4.625, 4.75, 4.875, 5.0, 5.125, 5.25, 5.375, 5.5, 5.625, 5.75, 5.875, 6.0, 6.142857142857143, 6.285714285714286, 6.428571428571429, 6.571428571428571, 6.714285714285714, 6.857142857142857, 7.0, 7.142857142857143, 7.285714285714286, 7.428571428571429, 7.571428571428571, 7.714285714285714, 7.857142857142857, 8.0, 8.142857142857142, 8.285714285714286, 8.428571428571429, 8.571428571428571, 8.714285714285714, 8.857142857142858, 9.0, 9.142857142857142, 9.285714285714286, 9.428571428571429, 9.571428571428571, 9.714285714285714, 9.857142857142858, 10.0, 10.142857142857142, 10.285714285714286, 10.428571428571429, 10.571428571428571, 10.714285714285714, 10.857142857142858, 11.0, 11.142857142857142, 11.285714285714286, 11.428571428571429, 11.571428571428571, 11.714285714285714, 11.857142857142858, 12.0, 12.125, 12.25, 12.375, 12.5, 12.625, 12.75, 12.875, 13.0, 13.125, 13.25, 13.375, 13.5, 13.625, 13.75, 13.875, 14.0, 14.142857142857142, 14.285714285714286, 14.428571428571429, 14.571428571428571, 14.714285714285714, 14.857142857142858, 15.0, 15.142857142857142, 15.285714285714286, 15.428571428571429, 15.571428571428571, 15.714285714285714, 15.857142857142858, 16.0, 16.142857142857142, 16.285714285714285, 16.428571428571427, 16.571428571428573, 16.714285714285715, 16.857142857142858, 17.0, 17.142857142857142, 17.285714285714285, 17.428571428571427, 17.571428571428573, 17.714285714285715, 17.857142857142858, 18.0, 18.142857142857142, 18.285714285714285, 18.428571428571427, 18.571428571428573, 18.714285714285715, 18.857142857142858, 19.0, 19.142857142857142, 19.285714285714285, 19.428571428571427, 19.571428571428573, 19.714285714285715, 19.857142857142858, 20.0, 20.125, 20.25, 20.375, 20.5, 20.625, 20.75, 20.875, 21.0, 21.125, 21.25, 21.375, 21.5, 21.625, 21.75, 21.875, 22.0, 22.142857142857142, 22.285714285714285, 22.428571428571427, 22.571428571428573, 22.714285714285715, 22.857142857142858, 23.0, 23.142857142857142, 23.285714285714285, 23.428571428571427, 23.571428571428573, 23.714285714285715, 23.857142857142858, 24.0, 24.166666666666668, 24.333333333333332, 24.5, 24.666666666666668, 24.833333333333332], [-143.858, -13.775, -13.785, 122.665, -66.475, 31.541, 2.118, -24.67, 28.275000000000002, 0.139, -36.578, -28.396, 48.925000000000004, 9.287, -3.412, 70.053, -21.479, 14.89, -7.234, 5.521, -3.164, 19.558, -37.538000000000004, 37.11, -77.159, -13.755, 77.63, 28.249000000000002, -209.114, -44.569, 92.851, 173.641, -70.156, -22.722, 17.795, -6.59, 25.654, -41.882, 53.713, 9.237, -26.164, 18.357, 63.695, -8.542, 5.183, -5.99, 9.508000000000001, -5.462, -29.446, 36.574, -52.552, 51.439, -48.502, 0.73, -23.836000000000002, -3.648, -9.628, -5.485, -68.679, 95.486, -62.041000000000004, 54.633, -58.791000000000004, 68.305, -49.682, 29.838, -8.459, 3.213, -5.561, -80.617, 58.144, 15.346, -158.743, -40.726, 5.259, 3.258, 41.128, -54.377, 5.01, 18.84, 11.403, -20.73, 21.792, -17.296, 27.29, 0.783, -6.804, -137.476, 116.70700000000001, -6.929, 17.846, -3.586, 11.754, 6.341, 0.292, -0.911, -8.236, -5.312, 14.939, -29.945, 30.573, -9.991, -49.344, 82.117, -27.45, 22.291, -6.636, -9.389, 10.034, -14.218, 14.215, -7.3, 12.409, -44.302, 50.197, -36.089, -9.120000000000001, 45.881, 14.836, -27.324, 10.765, -10.139, -33.252, 2.737, -9.99, -6.019, -53.329, -28.159, 2.676, -36.9, -2.372, 8.92, 13.599, -25.723, -16.436, 7.722, -0.088, -29.122, 32.814, -20.521, 30.155, -45.734, 36.611000000000004, 74.528, 68.482, -22.548000000000002, -31.398, 134.603, -45.587, -0.981, -40.156, 24.441, 20.477, -31.424, 19.5, -11.789, 16.394000000000002, -38.567, 9.523, 0.09, -0.058, -4.8500000000000005, 11.71, 25.637, -10.51, -18.101, -12.389000000000001, 95.417, -138.726, 30.355, 96.245, -48.666000000000004, 40.851, -0.71]}, "gap value："=0, "BR Fill Pattern"=[], "time string (last INJ) "=""} ("Cluster"), "Tune X(from BPM)"=w228, "Tune Y(from BPM)"=w227, "date (last kicker ON)"=w234, "time string (last kicker ON)"=w233, "date"=w256, "time string"=w255, "Mode"=w338, "Beam Current(mA"=w337, "Beam Lifetime(min)"=w336, "Beamsize X(um)"=w335, "Beamsize Y(um)"=w334, "NuX(from BBF)"=w333, "NuY(from BBF)"=w332, "Bucket Start"=w331, "Bucket Last"=w330, "Bucket Step"=w329, "BR inj. sep.(V)"=w328, "BR inj. kicker(kV)"=w327, "BR ext. kicker1(kV)"=w326, "BR ext. kicker2(kV)"=w325, "BR ext. sep.1(V)"=w324, "BR ext. sep.2(V)"=w323, "SR inj. sep.1(V)"=w322, "SR inj. sep.2(V)"=w321, "SR kicker1(kV)"=w320, "SR kicker2(kV)"=w319, "SR kicker3(kV)"=w318, "SR kicker4(kV)"=w317, "Gun mode"=w316, "Grid volt.(V)[S]"=w315, "Gun volt.(V)[S]"=w314, "Mod.3 HV(kV)[S]"=w313, "Width count"=w312, "2ns step"=w311, "10ps delay"=w310, "RF2 remote"=w309, "RF2 OP mode"=w308, "RF2 phase.[S]"=w232, "RF Freq.(s)"=w307, "RF2 gap volt[S]"=w231, "RF3 remote"=w306, "RF3 OP mode"=w305, "RF3 phase.[S]"=w304, "RF3 gap volt.[S]"=w303, "BR"=w302, "BTS"=w301, "LI"=w299, "LTB"=w298, "SR"=w300, "SR Fill Pattern"=w81, "IU22-05 Hutch Enable"=w181, "IU22A-09M Hutch Enable"=w177, "IUT22-21M Hutch Enable"=w161, "IU22-23M Hutch Enable"=w144, "IU22A-25M Hutch Enable"=w143, "EPU48A-41M Hutch Enable"=w125, "EPU46-45M Hutch Enable"=w124, "EPU46-45 FE Enable"=w126, "EPU48A-41 FE Enable"=w127, "IU22A-25 FE Enable"=w145, "IU22-23 FE Enable"=w146, "IUT22-21 FE Enable"=w164, "IU22A-09 FE Enable"=w176, "IU22-05 FE Enable"=w182, "IU22-05gap(R)"=w297, "IU22A-09gap(R)"=w296, "IU22B-09gap(R)"=w295, "IUT22-21gap(R)"=w294, "IU22-23gap(R)"=w293, "IU22A-25gap(R)"=w292, "IU22B-25gap(R)"=w291, "EPU48A-41gap(R)"=w290, "EPU48A-41phase(R)"=w289, "EPU48B-41gap(R)"=w288, "EPU48B-41phase(R)"=w287, "EPU46-45gap(R)"=w286, "EPU46-45phase(R)"=w285, "Taper"=w229, "phase shifter"=w284, "05XBPMX 1"=w283, "09XBPMX 1"=w282, "21XBPMX 1"=w281, "23XBPMX 1"=w280, "25XBPMX 1"=w279, "41XBPMX 1"=w278, "45XBPMX 1"=w277, "05XBPMY 1"=w276, "09XBPMY 1"=w275, "21XBPMY 1"=w274, "23XBPMY 1"=w273, "25XBPMY 1"=w272, "41XBPMY 1"=w271, "45XBPMY 1"=w270, "IU22-05M"=w269, "IU22A-09M"=w268, "IU22B-09M"=w267, "IUT22-21M"=w266, "IU22-23M"=w265, "IU22A-25M"=w264, "IU22B-25M"=w263, "EPU48A-41gM"=w262, "EPU48B-41gM"=w261, "EPU46-45gM"=w260, "EPU48A-41pM"=w259, "EPU48B-41pM"=w258, "EPU46-45pM"=w257, "BPMX Graph 2"=w87, "BPMY Graph 2"=w86, "Radio Buttons 2"=enum32{"absolute", "different with"}."absolute", "FOFB H"=w240, "FOFB V"=w239, "BBF H"=w238, "BBF V"=w237, "Orbit ILK(P)"=w236, "05XBPMX 2"=w171, "05XBPMY 2"=w170, "09XBPMX 2"=w169, "09XBPMY 2"=w168, "21XBPMX 2"=w153, "21XBPMY 2"=w152, "23XBPMX 2"=w151, "23XBPMY 2"=w150, "25XBPMX 2"=w133, "25XBPMY 2"=w132, "41XBPMX 2"=w131, "41XBPMY 2"=w130, "45XBPMX 2"=w129, "45XBPMY 2"=w128, "05 mode"=w107, "09A mode"=w106, "09B mode"=w105, "21 mode"=w104, "23 mode"=w103, "25A mode"=w102, "25B mode"=w101, "41A mode"=w100, "41B mode"=w99, "46 mode"=w98, "BeamCurrent History"=w94, "RF FB"=w90, "gap value："=w80, "BR Fill Pattern"=w68, "time string (last INJ)"=w66) -> (→"Cluster":T1)
  }
  n269 = while {
    tunnel: w10 -> [_]
    shift-right: [w838] -> _
    shift-left: string[] [] -> [w835]
    shift-right: [w825] -> _
    shift-left: string[][] [] -> [w828]
    tunnel: w18 -> [w831]
    i -> [w829]
    stop <- w830 stop-if-true
    w822 = 1000  # limit
    # "為了使檯面上記憶體不要使用太多而做的筆數限制"
    n270 = flat-sequence {
      tunnel: [w869] -> w839
      tunnel: [w868] -> w836
      tunnel: w835 -> [w868]
      tunnel: [w867] -> w832
      tunnel: w831 -> [w867]
      tunnel: [w879] -> w840
      tunnel: w839 -> [w879]
      tunnel: [w877] -> w837
      tunnel: w836 -> [w878]
      tunnel: [w871] -> w834
      tunnel: w832 -> [w870]
      tunnel: w840 -> [w902]
      tunnel: [w900] -> w838
      tunnel: w837 -> [w900]
      tunnel: w834 -> [w899]
      tunnel: [w899] -> w833
      frame #0 {
        n271 = Tick Count (ms)() -> (millisecond timer value=w869:u32)
      }
      frame #1 {
        n272 = Get Date/Time In Seconds() -> (seconds since 1Jan1904=w874:timestamp)
        n273 = To Double Precision Float(number=w874) -> (double precision float=w873:dbl)
        n274 = Format Date/Time String(time format string (%c)="%Y/%m/%d %H:%M:%S", seconds (now)=w874) -> (date/time string=w875:string)  [unwired: 1 in]
        n275 = Number To Fractional String(number=w873) -> (F-format string=w872:string)  [unwired: 3 in]
        n276 = call-poly <userlib>:"CaLabGet.vi"("PV Names"=w870) -> ("1rst Value (string)"=w877:string[])  [unwired: 8 in, 6 out]
        n277 = for {
          tunnel: w878 -> [w881] mode=indexing
          tunnel: w877 -> [w880] mode=indexing
          tunnel: w870 -> [w889] mode=indexing
          tunnel: w875 -> [w888]
          tunnel: [w887] -> w871 mode=indexing if=w885
          tunnel: w872 -> [w886]
          i -> [w884]
          n278 = Greater Or Equal?(x=w884, y=1) -> (x >= y?=w882:bool)
          n279 = case shown="True" w882 {
            tunnel: w889 -> [_ w898]
            tunnel: w881 -> [_ w897]
            tunnel: w880 -> [_ w896]
            tunnel: w888 -> [_ w895]
            tunnel: [string[] [] w894] -> w887
            tunnel: w886 -> [_ w893]
            tunnel: [FALSE w892] -> w885
            frame False {
            }
            frame True {
              n280 = Not Equal?(x=w897, y=w896) -> (x != y?=w892:bool)
              n281 = Build Array(w895, w898, w897, w896, w893) -> (w894:string[])
            }
          }
        }
      }
      frame #2 {
        n282 = Tick Count (ms)() -> (millisecond timer value=w903:u32)
        n283 = Subtract(x=w903, y=w902) -> (x-y=→"dT":u32)
      }
    }
    n284 = while {
      i -> [w860]
      stop <- w864 stop-if-true
      # "每60秒，表示法:\n100 600"
      # "每十秒，表示法:\n100 100"
      n285 = local read "stop"() -> (w863:bool)
      n286 = Multiply(x="Check period", y=10) -> (x*y=w861:i32)
      n287 = Greater Or Equal?(x=w860, y=w861) -> (x >= y?=w865:bool)
      n288 = Wait Until Next ms Multiple(millisecond multiple=u32 99) -> ()  [unwired: 1 out]
      n289 = Or(x=w865, y=w863) -> (x .or. y?=w864:bool)
    }
    n290 = Array Size(array=w828) -> (size(s)=w827:i32[])
    n291 = Build Array (concatenate)(w828, w833) -> (w824:string[][])
    n292 = Index Array(array=w827, index=0) -> (element=w823:i32)
    "EVENTs" <- w823
    n293 = Greater Or Equal?(x=w823, y=w822) -> (x >= y?=w821:bool)
    n294 = case shown="True" w821 {
      tunnel: w824 -> [w841 w852]
      tunnel: [w841 w856] -> w825
      tunnel: w823 -> [_ w847]
      tunnel: w822 -> [_ w846]
      frame False {
      }
      frame True {
        n295 = call "Main_Daily_path.vi"() -> ("Directory path"=w843:path)  [unwired: 10 in, 1 out]
        n296 = Array Subset(array=w852, index (row)=0 ("index"), length (row)=w846, index (col)=0 ("index"), length (col)=5 ("length")) -> (w851:string[][])
        n297 = Build Path(base path=w843, name or relative path="Association\\changedPVsBKUP.csv" ("string")) -> (appended path=w842:path)
        n298 = Subtract(x=w847, y=w846) -> (x-y=w845:i32)
        n299 = call-poly <vilib>:"Write To Spreadsheet File.vi"("delimiter (\\t)"="," ("delimiter (\\t)"), "transpose? (no:F)"=FALSE, "append to file? (new file:F)"=TRUE, "2D data"=w851, "file path (dialog if empty)"=w842) -> ()  [unwired: 3 in, 1 out]
        n300 = Array Subset(array=w852, index (row)=w846, length (row)=w845, index (col)=0 ("index"), length (col)=5 ("length")) -> (w856:string[][])
      }
    }
    "Diff list" <- w825
    n301 = local read "stop"() -> (w830:bool)
    "check loop" <- w829
  }
  n302 = local write "stop"(FALSE ("stop")) -> ()
